vi "Lab Panel V4.0.vi"() -> ()   [LabVIEW 2013]
uses:
  <vilib>/Platform/TimedLoop/XDataNode/timing_clust.ctl
  <vilib>/Platform/TimedLoop/XDataNode/nitl_modes.ctl
  <vilib>/Platform/TimedLoop/XDataNode/wakeup.ctl
  Global 1.vi
  <vilib>/platform/TimedLoop/XDataNode/XDataNode.xnode
  <vilib>/Platform/TimedLoop/XDataNode/XDNodeRunTimeDep.lvlib
panel:
  out "TEMP update":bool
  out "AI update":bool
  in  "stop":bool
  in  "Tab Control 2":T1(tab)
  out "SIG LAB05-2":T2 {"PF" format="%.2f"; "AMPS" format="%.1f"}
  out "SIG LAB05-1":T2 {"PF" format="%.2f"; "AMPS" format="%.1f"}
  out "SIG LAB04-2":T2 {"PF" format="%.2f"; "AMPS" format="%.1f"}
  out "SIG LAB04-1":T2 {"PF" format="%.2f"; "AMPS" format="%.1f"}
  out "SIG LAB03-2":T2 {"PF" format="%.2f"; "AMPS" format="%.1f"}
  out "SIG LAB03-1":T2 {"PF" format="%.2f"; "AMPS" format="%.1f"}
  out "SIG LAB02-2":T2 {"PF" format="%.2f"; "AMPS" format="%.1f"}
  in  "RUN LAB01-1":bool
  in  "O/I  LAB05-1":bool
  in  "O/I  LAB05-2":bool
  in  "O/I  LAB04-1":bool
  in  "O/I  LAB04-2":bool
  in  "O/I  LAB02-1":bool
  in  "O/1  LAB02-2":bool
  in  "O/I  LAB01-2":bool
  in  "O/I  LAB01-1":bool
  in  "O/I  LAB03-1":bool
  in  "RUN LAB05-2":bool
  in  "RUN LAB05-1":bool
  in  "RUN LAB04-2":bool
  in  "RUN LAB04-1":bool
  in  "RUN LAB03-2":bool
  in  "RUN LAB03-1":bool
  in  "RUN LAB02-2":bool
  in  "RUN LAB02-1":bool
  in  "RUN LAB01-2":bool
  in  "SELECT LAB05-2":T3(radio)
  in  "SELECT LAB05-1":T3(radio)
  in  "SELECT LAB04-2":T3(radio)
  in  "SELECT LAB04-1":T3(radio)
  in  "SELECT LAB03-2":T3(radio)
  in  "SELECT LAB03-1":T3(radio)
  in  "SELECT LAB02-2":T3(radio)
  in  "SELECT LAB02-1":T3(radio)
  in  "SELECT LAB01-2":T3(radio)
  in  "SELECT LAB01-1":T3(radio)
  in  "O/I  LAB03-2":bool
  out "SIG LAB01-1":T2 {"PF" format="%.2f"; "AMPS" format="%.1f"}
  out "SIG LAB01-2":T2 {"PF" format="%.2f"; "AMPS" format="%.1f"}
  out "SIG LAB02-1":T2 {"PF" format="%.2f"; "AMPS" format="%.1f"}
  out "DISP LAB05-2":T4 {"MINS" format="%.2g"}
  out "DISP LAB05-1":T4 {"MINS" format="%.2g"}
  out "DISP LAB04-2":T4 {"MINS" format="%.2g"}
  out "DISP LAB04-1":T4 {"MINS" format="%.2g"}
  out "DISP LAB03-2":T4 {"MINS" format="%.2g"}
  out "DISP LAB03-1":T4 {"MINS" format="%.2g"}
  in  "SET LAB05-2":T5={"NAME"="", "DESCRIPTION"="", "CYCLES"=5.0, "T-RISE mins"=0.0, "T-RISE deg C"=0.0} {"CYCLES" min=5.0 step=1.0}
  in  "SET LAB05-1":T5={"NAME"="", "DESCRIPTION"="", "CYCLES"=5.0, "T-RISE mins"=0.0, "T-RISE deg C"=0.0} {"CYCLES" min=5.0 step=1.0}
  in  "SET LAB04-2":T5={"NAME"="", "DESCRIPTION"="", "CYCLES"=5.0, "T-RISE mins"=0.0, "T-RISE deg C"=0.0} {"CYCLES" min=5.0 step=1.0}
  in  "SET LAB04-1":T5={"NAME"="", "DESCRIPTION"="", "CYCLES"=5.0, "T-RISE mins"=0.0, "T-RISE deg C"=0.0} {"CYCLES" min=5.0 step=1.0}
  in  "SET LAB03-2":T5={"NAME"="", "DESCRIPTION"="", "CYCLES"=5.0, "T-RISE mins"=0.0, "T-RISE deg C"=0.0} {"CYCLES" min=5.0 step=1.0}
  in  "SET LAB03-1":T5={"NAME"="", "DESCRIPTION"="", "CYCLES"=5.0, "T-RISE mins"=0.0, "T-RISE deg C"=0.0} {"CYCLES" min=5.0 step=1.0}
  out "DISP LAB02-2":T4 {"MINS" format="%.2g"}
  out "DISP LAB02-1":T4 {"MINS" format="%.2g"}
  in  "SET LAB02-2":T5={"NAME"="", "DESCRIPTION"="", "CYCLES"=5.0, "T-RISE mins"=0.0, "T-RISE deg C"=0.0} {"CYCLES" min=5.0 step=1.0}
  in  "SET LAB02-1":T5={"NAME"="", "DESCRIPTION"="", "CYCLES"=5.0, "T-RISE mins"=0.0, "T-RISE deg C"=0.0} {"CYCLES" min=5.0 step=1.0}
  out "RESULT LAB05-2":bool
  out "RESULT LAB05-1":bool
  out "RESULT LAB04-2":bool
  out "RESULT LAB04-1":bool
  out "RESULT LAB03-2":bool
  out "RESULT LAB03-1":bool
  out "RESULT LAB02-2":bool
  out "RESULT LAB02-1":bool
  out "RESULT LAB01-2":bool
  out "RESULT LAB01-1":bool
  in  "SET LAB01-1":T5={"NAME"="", "DESCRIPTION"="", "CYCLES"=5.0, "T-RISE mins"=0.0, "T-RISE deg C"=0.0} {"CYCLES" min=5.0 step=1.0}
  in  "SET LAB01-2":T5={"NAME"="", "DESCRIPTION"="", "CYCLES"=5.0, "T-RISE mins"=0.0, "T-RISE deg C"=0.0} {"CYCLES" min=5.0 step=1.0}
  out "DISP LAB01-1":T4 {"MINS" format="%.2g"}
  out "DISP LAB01-2":T4 {"MINS" format="%.2f"}
  out "TEMP RISE LAB05-2":cluster{"TL":dbl, "TN":dbl}
  out "TEMP RISE LAB05-1":cluster{"TL":dbl, "TN":dbl}
  out "TEMP RISE LAB04-2":cluster{"TL":dbl, "TN":dbl}
  out "TEMP RISE LAB04-1":cluster{"TL":dbl, "TN":dbl}
  out "TEMP RISE LAB03-2":cluster{"TL":dbl, "TN":dbl}
  out "TEMP RISE LAB03-1":cluster{"TL":dbl, "TN":dbl}
  out "TEMP RISE LAB02-2":cluster{"TL":dbl, "TN":dbl}
  out "TEMP RISE LAB02-1":cluster{"TL":dbl, "TN":dbl}
  out "TEMP RISE LAB01-2":cluster{"TL":dbl, "TN":dbl}
  out "TEMP RISE LAB01-1":cluster{"TL":dbl, "TN":dbl}
  in  "JIG OFF TIME (S)":dbl=2.0 min=2.0 max=10.0 step=0.5 format="%.1g"
  in  "JIG ON TIME (S)":dbl=1.0 min=1.0 max=10.0 step=0.5 format="%.1g"
  out "JIG LAB05-2":bool
  out "JIG LAB05-1":bool
  out "JIG LAB04-2":bool
  out "JIG LAB04-1":bool
  out "JIG LAB03-2":bool
  out "JIG LAB03-1":bool
  out "JIG LAB02-2":bool
  out "JIG LAB02-1":bool
  out "JIG LAB01-2":bool
  out "JIG LAB01-1":bool
  out "TEMP START LAB01-1":cluster{"TL":dbl, "TN":dbl}
  out "TEMP START LAB02-1":cluster{"TL":dbl, "TN":dbl}
  out "TEMP START LAB03-1":cluster{"TL":dbl, "TN":dbl}
  out "TEMP START LAB04-1":cluster{"TL":dbl, "TN":dbl}
  out "TEMP START LAB01-2":cluster{"TL":dbl, "TN":dbl}
  out "TEMP START LAB02-2":cluster{"TL":dbl, "TN":dbl}
  out "TEMP START LAB03-2":cluster{"TL":dbl, "TN":dbl}
  out "TEMP START LAB04-2":cluster{"TL":dbl, "TN":dbl}
  out "TEMP START LAB05-2":cluster{"TL":dbl, "TN":dbl}
  out "TEMP START LAB05-1":cluster{"TL":dbl, "TN":dbl}
  in  "MAIL SETTINGS":T6
  out "MAIL REPORT":string
  in  "TO (string):":string
  in  "Send Mail Now":bool
  in  "Auto Mail Send":bool
  in  "Network Directory":path
  out "CAL LAB01":T7 {"2 (TN) cal" min=0.0 step=0.01 format="%.2f"; "2 (TL) cal" min=0.0 step=0.01 format="%.2f"; "2 (PF) cal" min=0.0 step=0.01 format="%.2f"; "2 (V) cal" min=0.0 step=0.01 format="%.2f"; "2 (A) cal" min=0.0 step=0.01 format="%.2f"; "1 (TN) cal" min=0.0 step=0.01 format="%.2f"; "1 (TL) cal" min=0.0 step=0.01 format="%.2f"; "1 (PF) cal" min=0.0 step=0.01 format="%.2f"; "1 (V) cal" min=0.0 step=0.01 format="%.2f"; "1  (A) cal" min=0.0 step=0.01 format="%.2f"}
  out "CAL LAB03":T7 {"2 (TN) cal" min=0.0 step=0.01 format="%.2f"; "2 (TL) cal" min=0.0 step=0.01 format="%.2f"; "2 (PF) cal" min=0.0 step=0.01 format="%.2f"; "2 (V) cal" min=0.0 step=0.01 format="%.2f"; "2 (A) cal" min=0.0 step=0.01 format="%.2f"; "1 (TN) cal" min=0.0 step=0.01 format="%.2f"; "1 (TL) cal" min=0.0 step=0.01 format="%.2f"; "1 (PF) cal" min=0.0 step=0.01 format="%.2f"; "1 (V) cal" min=0.0 step=0.01 format="%.2f"; "1  (A) cal" min=0.0 step=0.01 format="%.2f"}
  out "CAL LAB02":T8 {"2 (TN) cal" min=0.0 step=0.01 format="%.2f"; "2 (TL) cal" min=0.0 step=0.01 format="%.2f"; "2 (PF) cal" min=0.0 step=0.01 format="%.2f"; "2 (V) cal" min=0.0 step=0.01 format="%.2f"; "2 (A) cal" min=0.0 step=0.01 format="%.2f"; "1 (TN) cal" min=0.0 step=0.01 format="%.2f"; "1 (TL) cal" min=0.0 step=0.01 format="%.2f"; "1 (PF) cal" min=0.0 step=0.01 format="%.2f"; "1 (V) cal" min=0.0 step=0.01 format="%.2f"; "1 (A) cal" min=0.0 step=0.01 format="%.2f"}
  out "CAL LAB05":T7 {"2 (TN) cal" min=0.0 step=0.01 format="%.2f"; "2 (TL) cal" min=0.0 step=0.01 format="%.2f"; "2 (PF) cal" min=0.0 step=0.01 format="%.2f"; "2 (V) cal" min=0.0 step=0.01 format="%.2f"; "2 (A) cal" min=0.0 step=0.01 format="%.2f"; "1 (TN) cal" min=0.0 step=0.01 format="%.2f"; "1 (TL) cal" min=0.0 step=0.01 format="%.2f"; "1 (PF) cal" min=0.0 step=0.01 format="%.2f"; "1 (V) cal" min=0.0 step=0.01 format="%.2f"; "1  (A) cal" min=0.0 step=0.01 format="%.2f"}
  out "CAL LAB04":T7 {"2 (TN) cal" min=0.0 step=0.01 format="%.2f"; "2 (TL) cal" min=0.0 step=0.01 format="%.2f"; "2 (PF) cal" min=0.0 step=0.01 format="%.2f"; "2 (V) cal" min=0.0 step=0.01 format="%.2f"; "2 (A) cal" min=0.0 step=0.01 format="%.2f"; "1 (TN) cal" min=0.0 step=0.01 format="%.2f"; "1 (TL) cal" min=0.0 step=0.01 format="%.2f"; "1 (PF) cal" min=0.0 step=0.01 format="%.2f"; "1 (V) cal" min=0.0 step=0.01 format="%.2f"; "1  (A) cal" min=0.0 step=0.01 format="%.2f"}
  out "calibration file error out":errorcluster
  in  "CALIBRATE":bool
  in  "SHOW ADMIN PAGE":bool
  out "FAIL LAB05-2":cluster{"LO":dbl, "HI":dbl}
  out "FAIL LAB05-1":cluster{"LO":dbl, "HI":dbl}
  out "FAIL LAB04-2":cluster{"LO":dbl, "HI":dbl}
  out "FAIL LAB04-1":cluster{"LO":dbl, "HI":dbl}
  out "FAIL LAB03-2":cluster{"LO":dbl, "HI":dbl}
  out "FAIL LAB03-1":cluster{"LO":dbl, "HI":dbl}
  out "FAIL LAB02-2":cluster{"LO":dbl, "HI":dbl}
  out "FAIL LAB02-1":cluster{"LO":dbl, "HI":dbl}
  out "FAIL LAB01-2":cluster{"LO":dbl, "HI":dbl}
  out "FAIL LAB01-1":cluster{"LO":dbl, "HI":dbl}
  out "DATA LAB05-2":refnum<k1>
  out "DATA LAB05-1":refnum<k1>
  out "DATA LAB04-2":refnum<k1>
  out "DATA LAB04-1":refnum<k1>
  out "DATA LAB03-2":refnum<k1>
  out "DATA LAB03-1":refnum<k1>
  out "DATA LAB02-2":refnum<k1>
  out "DATA LAB02-1":refnum<k1>
  out "DATA LAB01-2":refnum<k1>
  in  "C drive data root dir":path
  out "run lab05-2":bool
  out "run lab05-1":bool
  out "run lab04-2":bool
  out "run lab04-1":bool
  out "run lab03-2":bool
  out "run lab03-1":bool
  out "run lab02-2":bool
  out "run lab02-1":bool
  out "run lab01-2":bool
  out "run lab01-1":bool
  out "stop2":bool
  in  "Tab Control":T9(tab)
  out "LAB01-2 (GRAPH)":dynamicdata(graph)
  out "LAB01-1 (GRAPH)":dynamicdata(graph)
  out "LAB02-2 (GRAPH)":dynamicdata(graph)
  out "LAB02-1 (GRAPH)":dynamicdata(graph)
  out "LAB03-2 (GRAPH)":dynamicdata(graph)
  out "LAB03-1 (GRAPH)":dynamicdata(graph)
  out "LAB04-2 (GRAPH)":dynamicdata(graph)
  out "LAB04-1 (GRAPH)":dynamicdata(graph)
  out "LAB05-2 (GRAPH)":dynamicdata(graph)
  out "LAB05-1 (GRAPH)":dynamicdata(graph)
  out "LAB05 TEMP":T10
  out "LAB04 TEMP":T10
  out "LAB02 TEMP":T10
  out "LAB01 TEMP":T10
  out "LAB03 TEMP":T10
  out "Analog Error Array":errorcluster[](array[cluster])
  out "AI loop time":dbl format="%.6g"
  out "loops":dbl
  in  "loop  delay(mS)":dbl
  out "on loops":dbl
  out "off loops":dbl
  out "jig cycle":dbl
  out "data file error":errorcluster
  out "mail control":string
  out "DATA LAB01-1":refnum<k1>
  # "LAB01"
  # "LAB02"
  # "LAB05"
  # "LAB03"
  # "LAB04"
  # "LAB01"
  # "LAB02"
  # "LAB03"
  # "LAB04"
  # "LAB05"
  # "JIG SET"
  # "(Enter recipients address seperated by comma)"
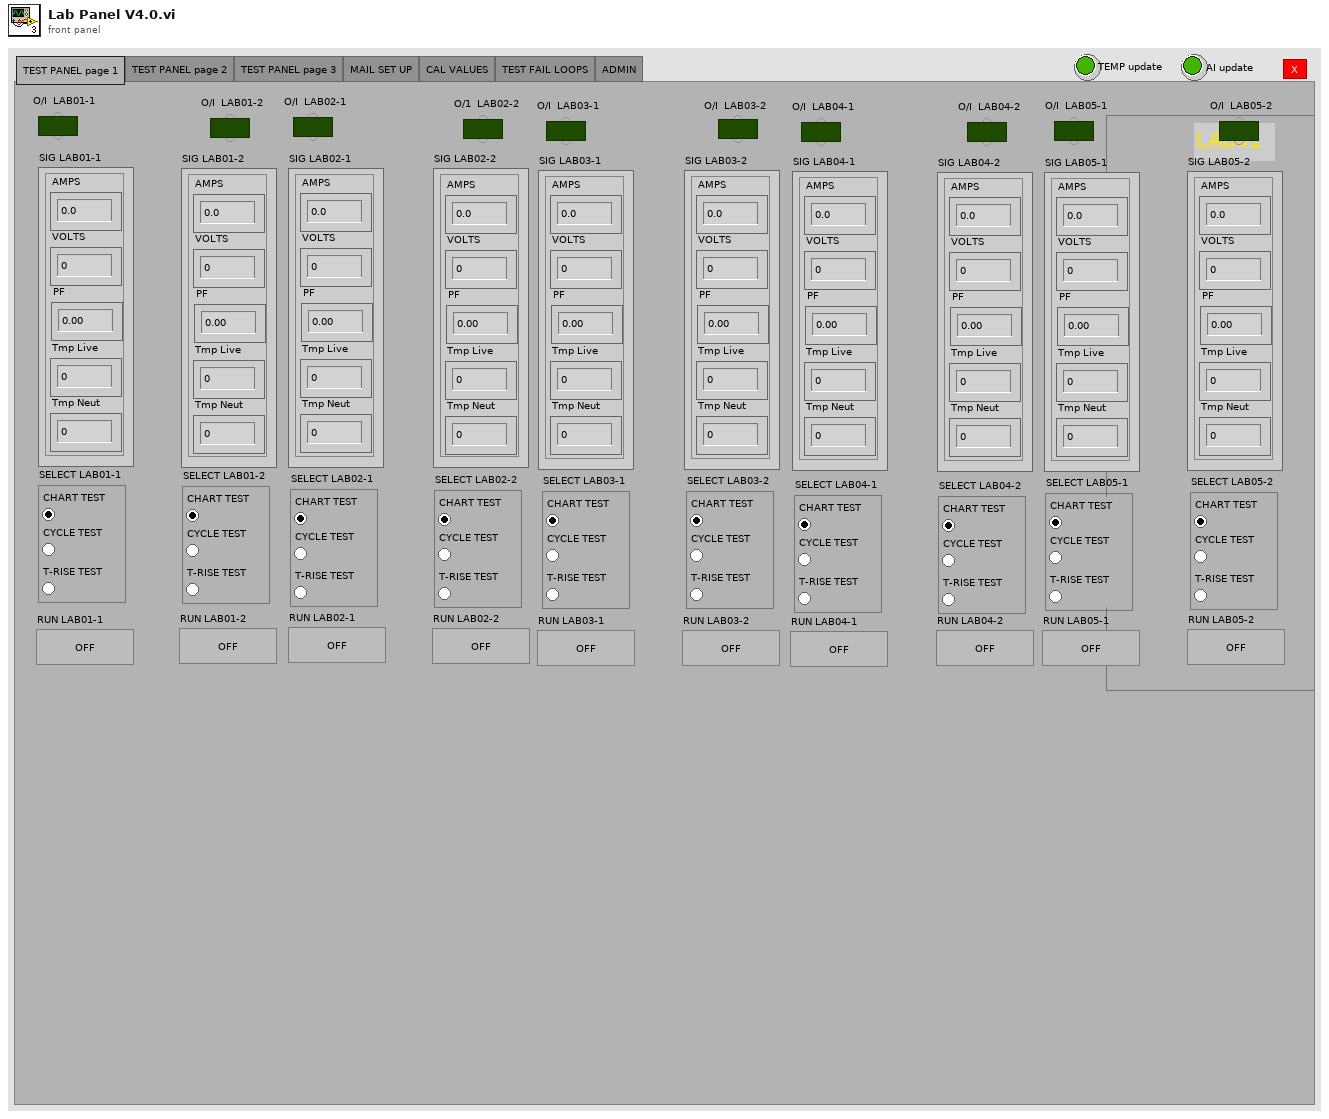
[diagram p1: front panel]
types:
  T1 = enum32{"TEST PANEL page 1", "TEST PANEL page 2", "TEST PANEL page 3", "MAIL SET UP", "CAL VALUES", "TEST FAIL LOOPS", "ADMIN"}
  T2 = cluster{"AMPS":dbl, "VOLTS":dbl, "PF":dbl, "Tmp Live":dbl, "Tmp Neut":dbl}
  T3 = enum32{"CHART TEST", "CYCLE TEST", "T-RISE TEST"}
  T4 = cluster{"CYCLE":dbl, "MINS":dbl, "STATUS":string}
  T5 = cluster{"NAME":string, "DESCRIPTION":string, "CYCLES":dbl, "T-RISE mins":dbl, "T-RISE deg C":dbl}
  T6 = cluster{"OUT SERVER ADDRESS":string, "FROM ACCOUNT":string, "USER NAME":string, "PASSWORD":string, "TEST MAIL":bool, "TEST MAIL STATUS":string, "mail error":errorcluster}
  T7 = cluster{"1  (A) cal":dbl, "1 (V) cal":dbl, "1 (PF) cal":dbl, "1 (TL) cal":dbl, "1 (TN) cal":dbl, "2 (A) cal":dbl, "2 (V) cal":dbl, "2 (PF) cal":dbl, "2 (TL) cal":dbl, "2 (TN) cal":dbl}
  T8 = cluster{"1 (A) cal":dbl, "1 (V) cal":dbl, "1 (PF) cal":dbl, "1 (TL) cal":dbl, "1 (TN) cal":dbl, "2 (A) cal":dbl, "2 (V) cal":dbl, "2 (PF) cal":dbl, "2 (TL) cal":dbl, "2 (TN) cal":dbl}
  T9 = enum32{"LAB01", "LAB02", "LAB03", "LAB04", "LAB05", "TEMPERATURE", "ERROR"}
  T10 = cluster{"T1 Live":dbl, "T1 Neut":dbl, "T2 Live":dbl, "T2 Neut":dbl, "ID":dbl, "ER":dbl}
  T11 = enum8{"Enabled", "Disabled", "Disabled and Grayed Out"}
  T12 = typedef "XDNodeRunTimeDep.lvlib/timing_clust.ctl" = cluster{"Expected End [f-1]":u64, "Actual End [f-1]":u64, "Finished Late? [f-1]":bool, "Expected End [i-1]":u64, "Actual End [i-1]":u64, "Finished Late? [i-1]":bool, "Expected Start [i]":u64, "Actual Start [i]":u64, "Expected Start [f]":u64, "Actual Start [f]":u64, "Source Name":string, "Structure Name":string, "Period":i64, "Deadline":i64, "Offset":i64, "Start":i64, "Priority":i32, "Timeout":i32, "Mode":T13, "Wakeup Reason":T14, "Error":errorcluster, "Source Type":string, "Secondary Source Type":string, "Global End Time":u64, "Global Start Time":u64, "Frame Duration":u64, "Iteration Duration":u64, "Assigned CPU":i32, "I/O Scan Engine Mode":u32}
  T13 = typedef "XDNodeRunTimeDep.lvlib/nitl_modes.ctl" = enum32{"No Change", "Process missed periods, maintain original phase", "Discard missed periods, maintain original phase", "Process missed periods, ignore original phase", "Discard missed periods, ignore original phase"}
  T14 = typedef "XDNodeRunTimeDep.lvlib/wakeup.ctl" = enum32{"Normal", "Aborted", "Asynchronous wakeup", "Timing source error", "Timed loop error", "Timeout"}
  T15 = enum16{"open", "replace", "create", "open or create", "replace or create", "replace or create with confirmation"}
  T16 = cluster{"SET LAB01-1":cluster{"NAME":string, "DESCRIPTION":string, "CYCLES":dbl, "T-RISE mins":dbl, "T-RISE deg C":dbl}, "SET LAB01-2":cluster{"NAME":string, "DESCRIPTION":string, "CYCLES":dbl, "T-RISE mins":dbl, "T-RISE deg C":dbl}, "SET LAB02-1":cluster{"NAME":string, "DESCRIPTION":string, "CYCLES":dbl, "T-RISE mins":dbl, "T-RISE deg C":dbl}, "SET LAB02-2":cluster{"NAME":string, "DESCRIPTION":string, "CYCLES":dbl, "T-RISE mins":dbl, "T-RISE deg C":dbl}, "SET LAB03-1":cluster{"NAME":string, "DESCRIPTION":string, "CYCLES":dbl, "T-RISE mins":dbl, "T-RISE deg C":dbl}, "SET LAB03-2":cluster{"NAME":string, "DESCRIPTION":string, "CYCLES":dbl, "T-RISE mins":dbl, "T-RISE deg C":dbl}, "SET LAB04-1":cluster{"NAME":string, "DESCRIPTION":string, "CYCLES":dbl, "T-RISE mins":dbl, "T-RISE deg C":dbl}, "SET LAB04-2":cluster{"NAME":string, "DESCRIPTION":string, "CYCLES":dbl, "T-RISE mins":dbl, "T-RISE deg C":dbl}, "SET LAB05-1":cluster{"NAME":string, "DESCRIPTION":string, "CYCLES":dbl, "T-RISE mins":dbl, "T-RISE deg C":dbl}, "SET LAB05-2":cluster{"NAME":string, "DESCRIPTION":string, "CYCLES":dbl, "T-RISE mins":dbl, "T-RISE deg C":dbl}, "Network Directory":path, "C drive data root dir":path}
  T17 = cluster{"MAIL SETTINGS":cluster{"OUT SERVER ADDRESS":string, "FROM ACCOUNT":string, "USER NAME":string, "PASSWORD":string, "TEST MAIL":bool, "TEST MAIL STATUS":string, "mail error":errorcluster}, "Auto Mail Send":bool, string}
  T18 = cluster{"SET LAB01-1":cluster{"NAME":string, "DESCRIPTION":string, "CYCLES":dbl, "T-RISE mins":dbl, "T-RISE deg C":dbl}, "SIG LAB01-1":cluster{"AMPS":dbl, "VOLTS":dbl, "PF":dbl, "Tmp Live":dbl, "Tmp Neut":dbl}, "DISP LAB01-1":cluster{"CYCLE":dbl, "MINS":dbl, "STATUS":string}}
  T19 = cluster{"SET LAB02-1":cluster{"NAME":string, "DESCRIPTION":string, "CYCLES":dbl, "T-RISE mins":dbl, "T-RISE deg C":dbl}, "SIG LAB02-1":cluster{"AMPS":dbl, "VOLTS":dbl, "PF":dbl, "Tmp Live":dbl, "Tmp Neut":dbl}, "DISP LAB02-1":cluster{"CYCLE":dbl, "MINS":dbl, "STATUS":string}}
  T20 = cluster{"SET LAB02-2":cluster{"NAME":string, "DESCRIPTION":string, "CYCLES":dbl, "T-RISE mins":dbl, "T-RISE deg C":dbl}, "SIG LAB02-2":cluster{"AMPS":dbl, "VOLTS":dbl, "PF":dbl, "Tmp Live":dbl, "Tmp Neut":dbl}, "DISP LAB02-2":cluster{"CYCLE":dbl, "MINS":dbl, "STATUS":string}}
  T21 = cluster{"SET LAB03-1":cluster{"NAME":string, "DESCRIPTION":string, "CYCLES":dbl, "T-RISE mins":dbl, "T-RISE deg C":dbl}, "SIG LAB03-1":cluster{"AMPS":dbl, "VOLTS":dbl, "PF":dbl, "Tmp Live":dbl, "Tmp Neut":dbl}, "DISP LAB03-1":cluster{"CYCLE":dbl, "MINS":dbl, "STATUS":string}}
  T22 = cluster{"SET LAB03-2":cluster{"NAME":string, "DESCRIPTION":string, "CYCLES":dbl, "T-RISE mins":dbl, "T-RISE deg C":dbl}, "SIG LAB03-2":cluster{"AMPS":dbl, "VOLTS":dbl, "PF":dbl, "Tmp Live":dbl, "Tmp Neut":dbl}, "DISP LAB03-2":cluster{"CYCLE":dbl, "MINS":dbl, "STATUS":string}}
  T23 = cluster{"SET LAB04-1":cluster{"NAME":string, "DESCRIPTION":string, "CYCLES":dbl, "T-RISE mins":dbl, "T-RISE deg C":dbl}, "SIG LAB04-1":cluster{"AMPS":dbl, "VOLTS":dbl, "PF":dbl, "Tmp Live":dbl, "Tmp Neut":dbl}, "DISP LAB04-1":cluster{"CYCLE":dbl, "MINS":dbl, "STATUS":string}}
  T24 = cluster{"SET LAB04-2":cluster{"NAME":string, "DESCRIPTION":string, "CYCLES":dbl, "T-RISE mins":dbl, "T-RISE deg C":dbl}, "SIG LAB04-2":cluster{"AMPS":dbl, "VOLTS":dbl, "PF":dbl, "Tmp Live":dbl, "Tmp Neut":dbl}, "DISP LAB04-2":cluster{"CYCLE":dbl, "MINS":dbl, "STATUS":string}}
  T25 = cluster{"SET LAB05-1":cluster{"NAME":string, "DESCRIPTION":string, "CYCLES":dbl, "T-RISE mins":dbl, "T-RISE deg C":dbl}, "SIG LAB05-1":cluster{"AMPS":dbl, "VOLTS":dbl, "PF":dbl, "Tmp Live":dbl, "Tmp Neut":dbl}, "DISP LAB05-1":cluster{"CYCLE":dbl, "MINS":dbl, "STATUS":string}}
  T26 = cluster{"SET LAB05-2":cluster{"NAME":string, "DESCRIPTION":string, "CYCLES":dbl, "T-RISE mins":dbl, "T-RISE deg C":dbl}, "SIG LAB05-2":cluster{"AMPS":dbl, "VOLTS":dbl, "PF":dbl, "Tmp Live":dbl, "Tmp Neut":dbl}, "DISP LAB05-2":cluster{"CYCLE":dbl, "MINS":dbl, "STATUS":string}}
  T27 = cluster{"T1":dbl, "T2":dbl, "T3":dbl, "T4":dbl, "ID":dbl, "ER":dbl}
  T28 = cluster{"LAB01-1 (A)":dbl, "LAB01-1 (V)":dbl, "LAB01-1 (PF)":dbl, "LAB01-2 (A)":dbl, "LAB01-2 (V)":dbl, "LAB01-2 (PF)":dbl}
  T29 = cluster{"LAB02-1 (A)":dbl, "LAB02-1 (V)":dbl, "LAB02-1 (PF)":dbl, "LAB02-2 (A)":dbl, "LAB02-2 (V)":dbl, "LAB02-2 (PF)":dbl}
  T30 = cluster{"LAB03-1 (A)":dbl, "LAB03-1 (V)":dbl, "LAB03-1 (PF)":dbl, "LAB03-2 (A)":dbl, "LAB03-2 (V)":dbl, "LAB03-2 (PF)":dbl}
  T31 = cluster{"LAB04-1 (A)":dbl, "LAB04-1 (V)":dbl, "LAB04-1 (PF)":dbl, "LAB04-2 (A)":dbl, "LAB04-2 (V)":dbl, "LAB04-2 (PF)":dbl}
  T32 = cluster{"LAB05-1 (A)":dbl, "LAB05-1 (V)":dbl, "LAB05-1 (PF)":dbl, "LAB05-2 (A)":dbl, "LAB05-2 (V)":dbl, "LAB05-2 (PF)":dbl}
  T33 = cluster{"SET LAB01-2":cluster{"NAME":string, "DESCRIPTION":string, "CYCLES":dbl, "T-RISE mins":dbl, "T-RISE deg C":dbl}, "SIG LAB01-2":cluster{"AMPS":dbl, "VOLTS":dbl, "PF":dbl, "Tmp Live":dbl, "Tmp Neut":dbl}, "DISP LAB01-2":cluster{"CYCLE":dbl, "MINS":dbl, "STATUS":string}}
  T34 = cluster{"FAIL LAB01-1":cluster{"LO":dbl, "HI":dbl}, "SIG LAB01-1":cluster{"AMPS":dbl, "VOLTS":dbl, "PF":dbl, "Tmp Live":dbl, "Tmp Neut":dbl}, "TEMP START LAB01-1":cluster{"TL":dbl, "TN":dbl}, "DISP LAB01-1":cluster{"CYCLE":dbl, "MINS":dbl, "STATUS":string}, "SET LAB01-1":cluster{"NAME":string, "DESCRIPTION":string, "CYCLES":dbl, "T-RISE mins":dbl, "T-RISE deg C":dbl}, "DATA LAB01-1":refnum<k1>}
  T35 = cluster{"FAIL LAB01-2":cluster{"LO":dbl, "HI":dbl}, "SIG LAB01-2":cluster{"AMPS":dbl, "VOLTS":dbl, "PF":dbl, "Tmp Live":dbl, "Tmp Neut":dbl}, "TEMP START LAB01-2":cluster{"TL":dbl, "TN":dbl}, "DISP LAB01-2":cluster{"CYCLE":dbl, "MINS":dbl, "STATUS":string}, "SET LAB01-2":cluster{"NAME":string, "DESCRIPTION":string, "CYCLES":dbl, "T-RISE mins":dbl, "T-RISE deg C":dbl}, "DATA LAB01-2":refnum<k1>}
  T36 = cluster{"FAIL LAB02-1":cluster{"LO":dbl, "HI":dbl}, "SIG LAB02-1":cluster{"AMPS":dbl, "VOLTS":dbl, "PF":dbl, "Tmp Live":dbl, "Tmp Neut":dbl}, "TEMP START LAB02-1":cluster{"TL":dbl, "TN":dbl}, "DISP LAB02-1":cluster{"CYCLE":dbl, "MINS":dbl, "STATUS":string}, "SET LAB02-1":cluster{"NAME":string, "DESCRIPTION":string, "CYCLES":dbl, "T-RISE mins":dbl, "T-RISE deg C":dbl}, "DATA LAB02-1":refnum<k1>}
  T37 = cluster{"FAIL LAB02-2":cluster{"LO":dbl, "HI":dbl}, "SIG LAB02-2":cluster{"AMPS":dbl, "VOLTS":dbl, "PF":dbl, "Tmp Live":dbl, "Tmp Neut":dbl}, "TEMP START LAB02-2":cluster{"TL":dbl, "TN":dbl}, "DISP LAB02-2":cluster{"CYCLE":dbl, "MINS":dbl, "STATUS":string}, "SET LAB02-2":cluster{"NAME":string, "DESCRIPTION":string, "CYCLES":dbl, "T-RISE mins":dbl, "T-RISE deg C":dbl}, "DATA LAB02-2":refnum<k1>}
  T38 = cluster{"FAIL LAB03-1":cluster{"LO":dbl, "HI":dbl}, "SIG LAB03-1":cluster{"AMPS":dbl, "VOLTS":dbl, "PF":dbl, "Tmp Live":dbl, "Tmp Neut":dbl}, "TEMP START LAB03-1":cluster{"TL":dbl, "TN":dbl}, "DISP LAB03-1":cluster{"CYCLE":dbl, "MINS":dbl, "STATUS":string}, "SET LAB03-1":cluster{"NAME":string, "DESCRIPTION":string, "CYCLES":dbl, "T-RISE mins":dbl, "T-RISE deg C":dbl}, "DATA LAB03-1":refnum<k1>}
  T39 = cluster{"FAIL LAB03-2":cluster{"LO":dbl, "HI":dbl}, "SIG LAB03-2":cluster{"AMPS":dbl, "VOLTS":dbl, "PF":dbl, "Tmp Live":dbl, "Tmp Neut":dbl}, "TEMP START LAB03-2":cluster{"TL":dbl, "TN":dbl}, "DISP LAB03-2":cluster{"CYCLE":dbl, "MINS":dbl, "STATUS":string}, "SET LAB03-2":cluster{"NAME":string, "DESCRIPTION":string, "CYCLES":dbl, "T-RISE mins":dbl, "T-RISE deg C":dbl}, "DATA LAB03-2":refnum<k1>}
  T40 = cluster{"FAIL LAB04-1":cluster{"LO":dbl, "HI":dbl}, "SIG LAB04-1":cluster{"AMPS":dbl, "VOLTS":dbl, "PF":dbl, "Tmp Live":dbl, "Tmp Neut":dbl}, "TEMP START LAB04-1":cluster{"TL":dbl, "TN":dbl}, "DISP LAB04-1":cluster{"CYCLE":dbl, "MINS":dbl, "STATUS":string}, "SET LAB04-1":cluster{"NAME":string, "DESCRIPTION":string, "CYCLES":dbl, "T-RISE mins":dbl, "T-RISE deg C":dbl}, "DATA LAB04-1":refnum<k1>}
  T41 = cluster{"FAIL LAB04-2":cluster{"LO":dbl, "HI":dbl}, "SIG LAB04-2":cluster{"AMPS":dbl, "VOLTS":dbl, "PF":dbl, "Tmp Live":dbl, "Tmp Neut":dbl}, "TEMP START LAB04-2":cluster{"TL":dbl, "TN":dbl}, "DISP LAB04-2":cluster{"CYCLE":dbl, "MINS":dbl, "STATUS":string}, "SET LAB04-2":cluster{"NAME":string, "DESCRIPTION":string, "CYCLES":dbl, "T-RISE mins":dbl, "T-RISE deg C":dbl}, "DATA LAB04-2":refnum<k1>}
  T42 = cluster{"FAIL LAB05-1":cluster{"LO":dbl, "HI":dbl}, "SIG LAB05-1":cluster{"AMPS":dbl, "VOLTS":dbl, "PF":dbl, "Tmp Live":dbl, "Tmp Neut":dbl}, "TEMP START LAB05-1":cluster{"TL":dbl, "TN":dbl}, "DISP LAB05-1":cluster{"CYCLE":dbl, "MINS":dbl, "STATUS":string}, "SET LAB05-1":cluster{"NAME":string, "DESCRIPTION":string, "CYCLES":dbl, "T-RISE mins":dbl, "T-RISE deg C":dbl}, "DATA LAB05-1":refnum<k1>}
  T43 = cluster{"FAIL LAB05-2":cluster{"LO":dbl, "HI":dbl}, "SIG LAB05-2":cluster{"AMPS":dbl, "VOLTS":dbl, "PF":dbl, "Tmp Live":dbl, "Tmp Neut":dbl}, "TEMP START LAB05-2":cluster{"TL":dbl, "TN":dbl}, "DISP LAB05-2":cluster{"CYCLE":dbl, "MINS":dbl, "STATUS":string}, "SET LAB05-2":cluster{"NAME":string, "DESCRIPTION":string, "CYCLES":dbl, "T-RISE mins":dbl, "T-RISE deg C":dbl}, "DATA LAB05-2":refnum<k1>}
  T44 = cluster{"MAIL SETTINGS":cluster{"OUT SERVER ADDRESS":string, "FROM ACCOUNT":string, "USER NAME":string, "PASSWORD":string, "TEST MAIL":bool, "TEST MAIL STATUS":string, "mail error":errorcluster}, "Auto Mail Send":bool, "TO (string):":string}
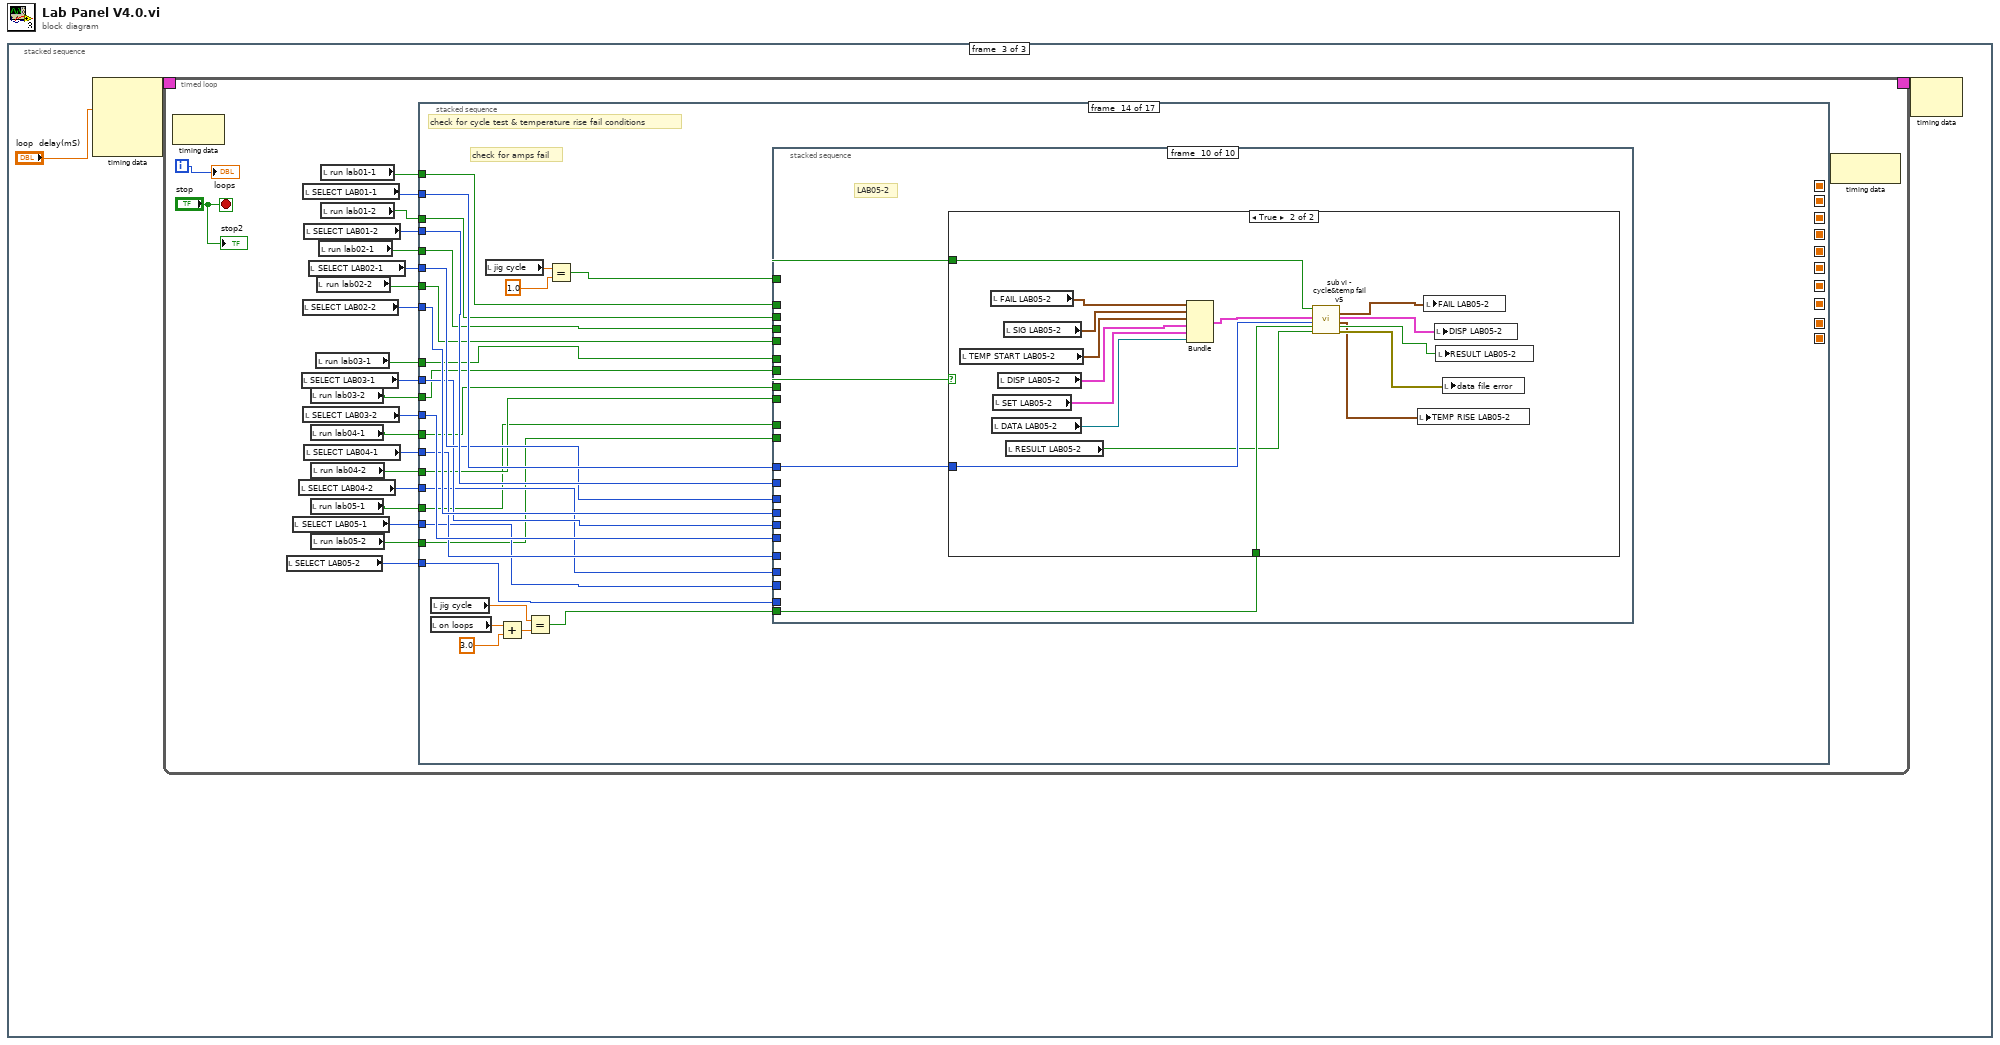
[diagram p0: block diagram]
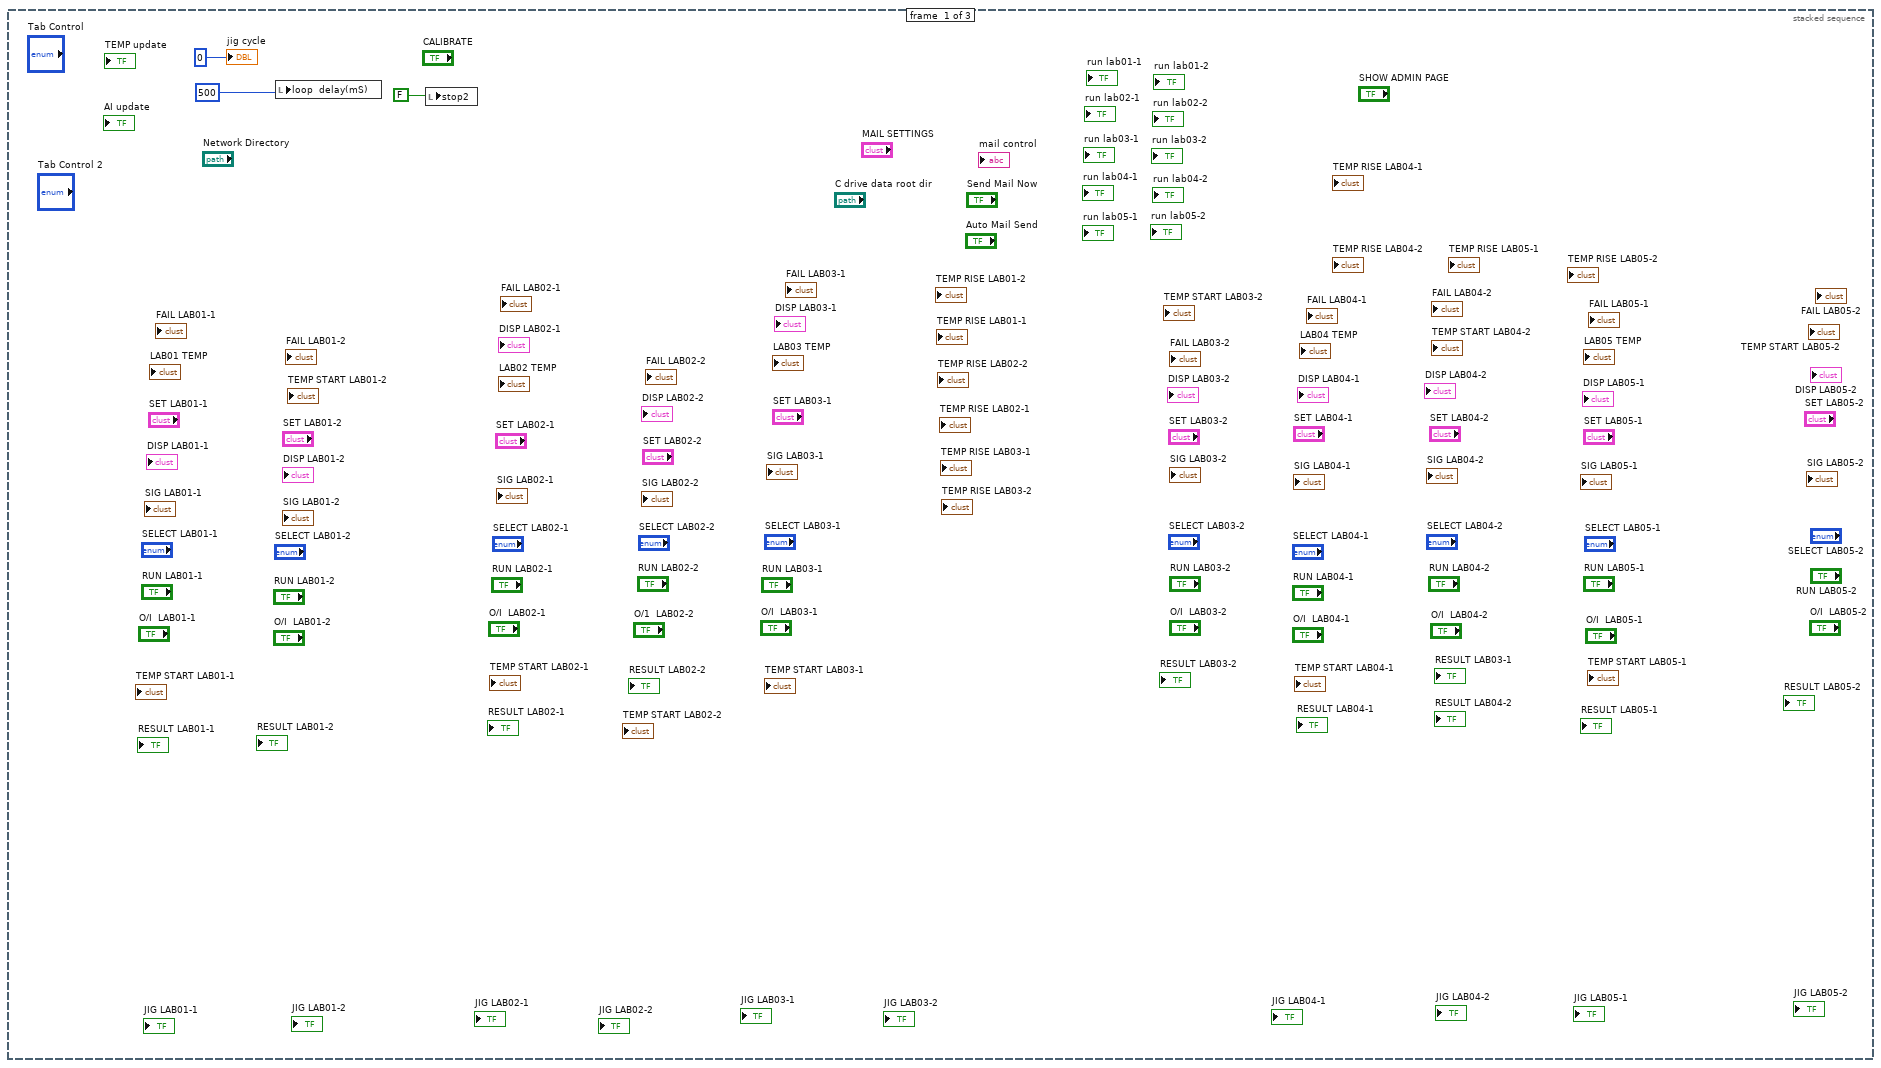
[diagram p2: hidden frame]
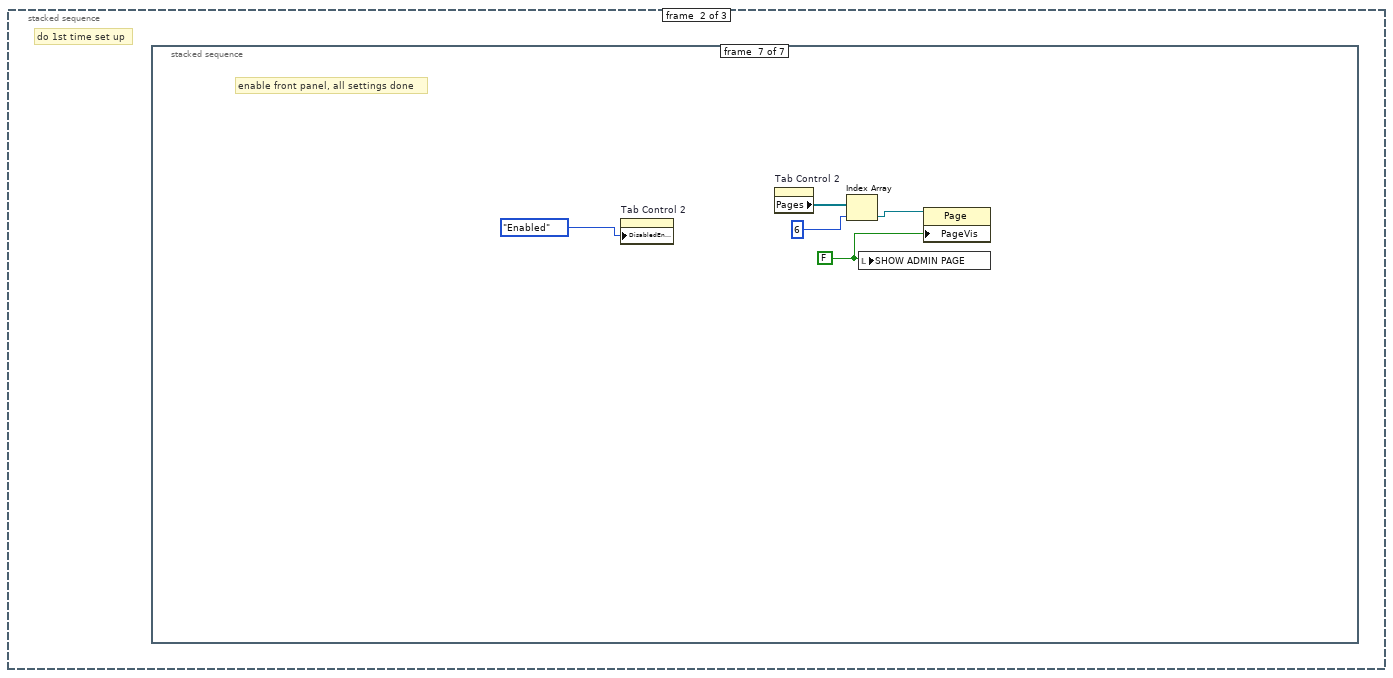
[diagram p3: hidden frame]
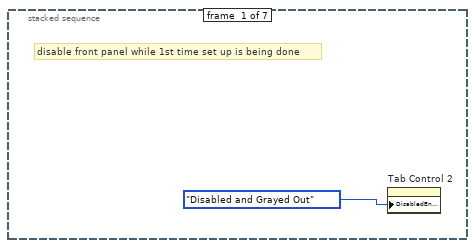
[diagram p4: hidden frame]
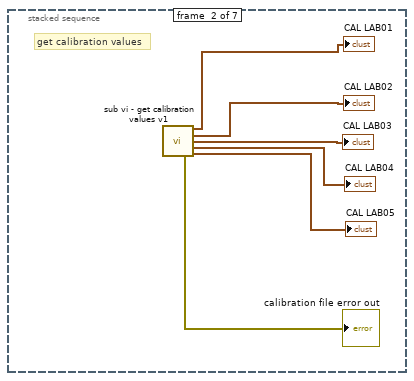
[diagram p5: hidden frame]
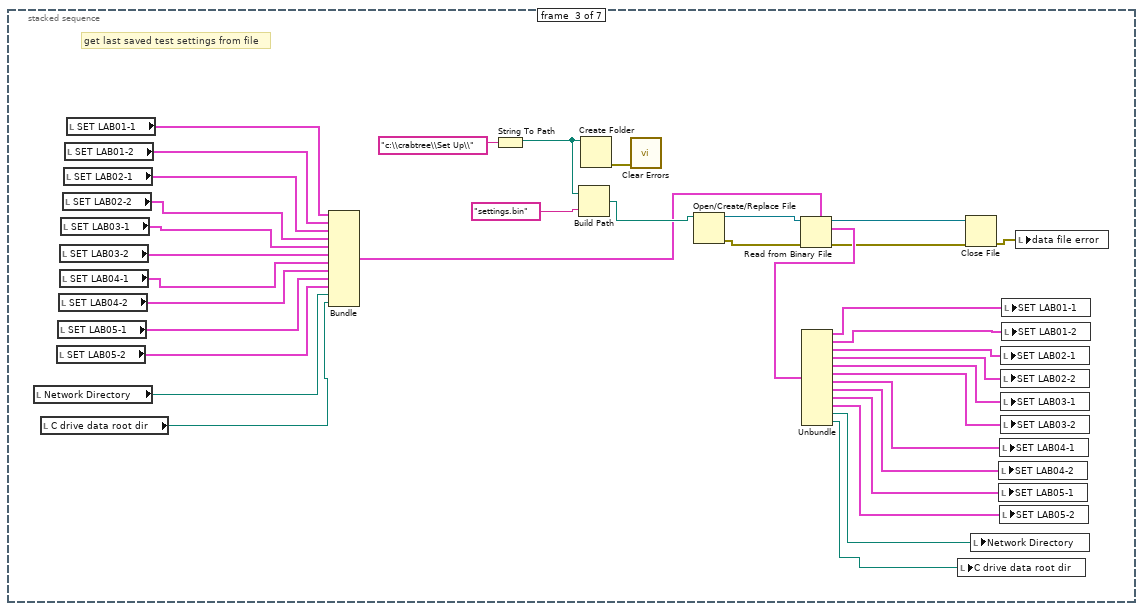
[diagram p6: hidden frame]
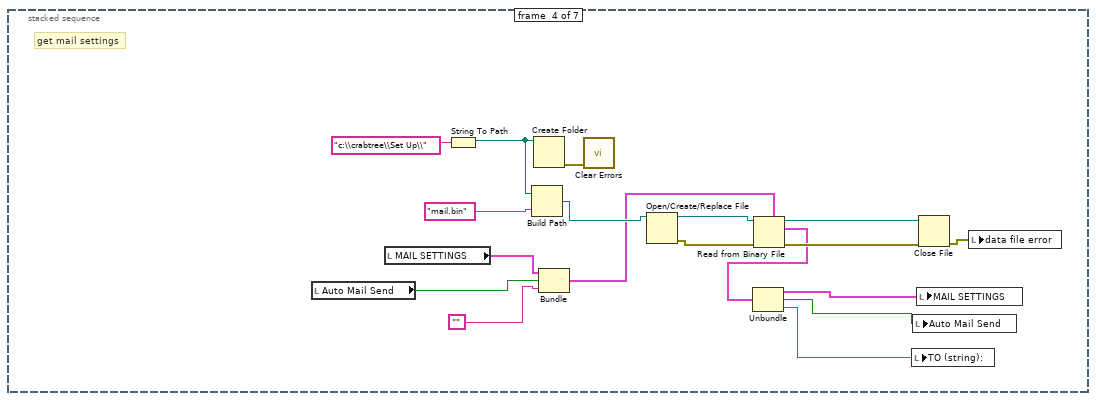
[diagram p7: hidden frame]
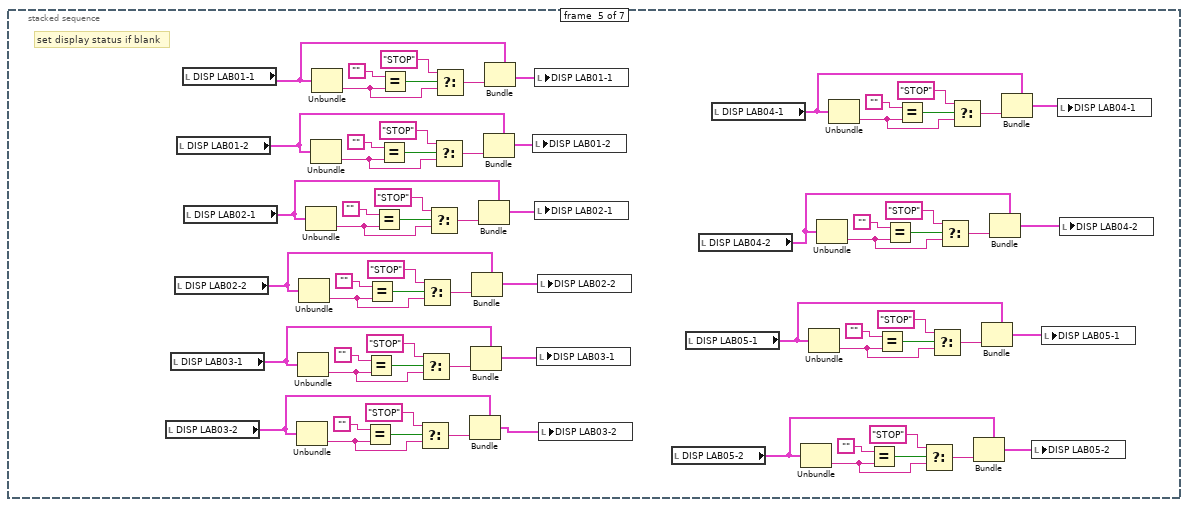
[diagram p8: hidden frame]
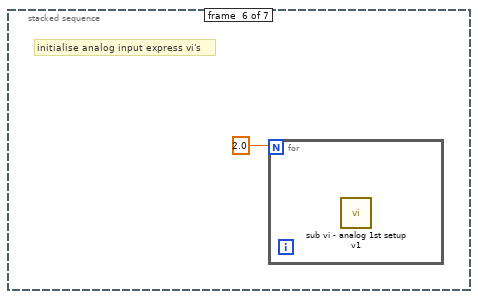
[diagram p9: hidden frame]
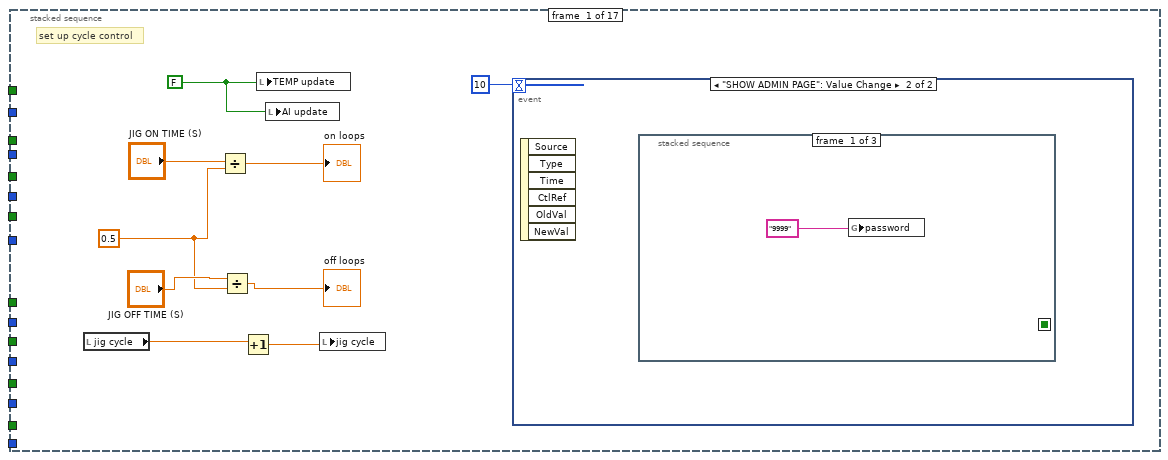
[diagram p10: hidden frame]
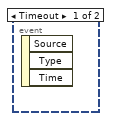
[diagram p11: hidden frame]
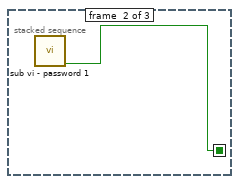
[diagram p12: hidden frame]
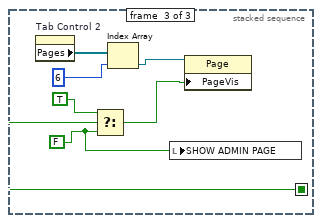
[diagram p13: hidden frame]
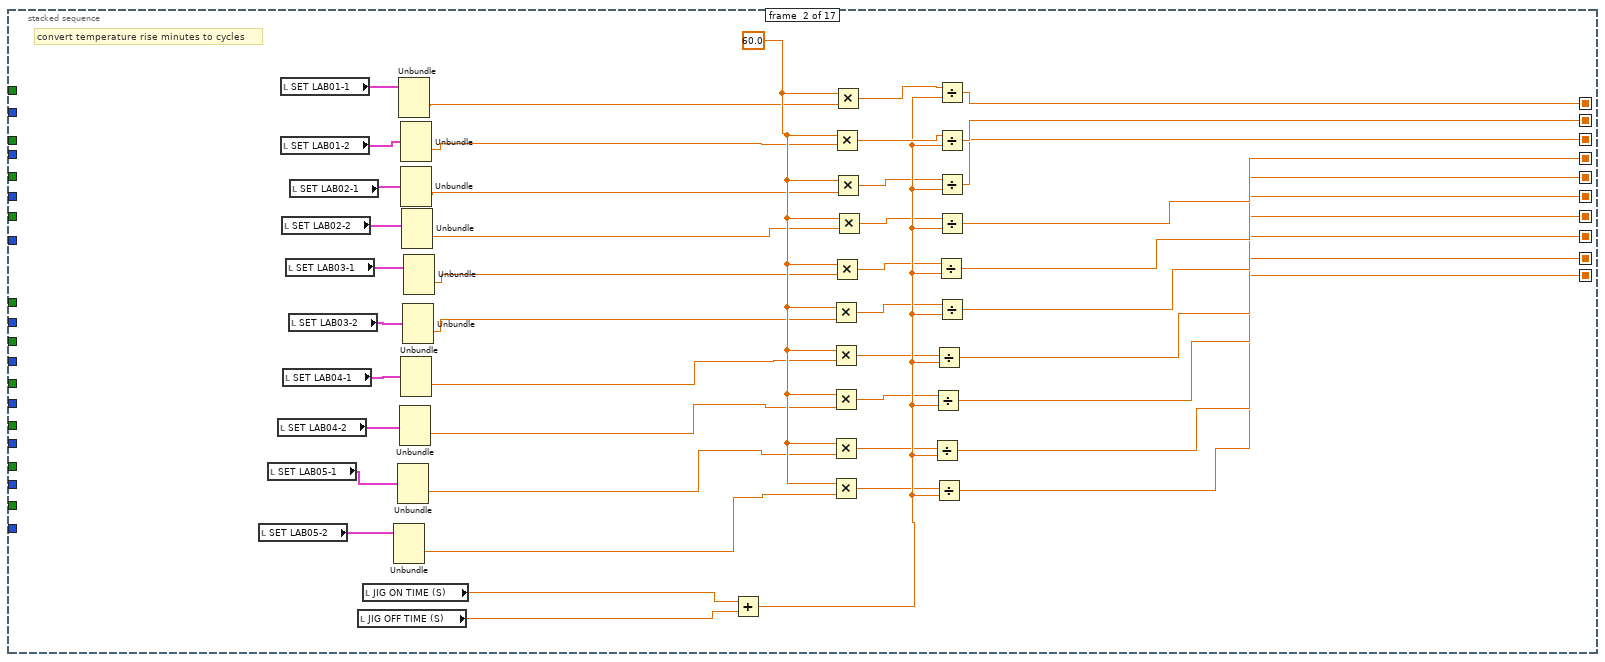
[diagram p14: hidden frame]
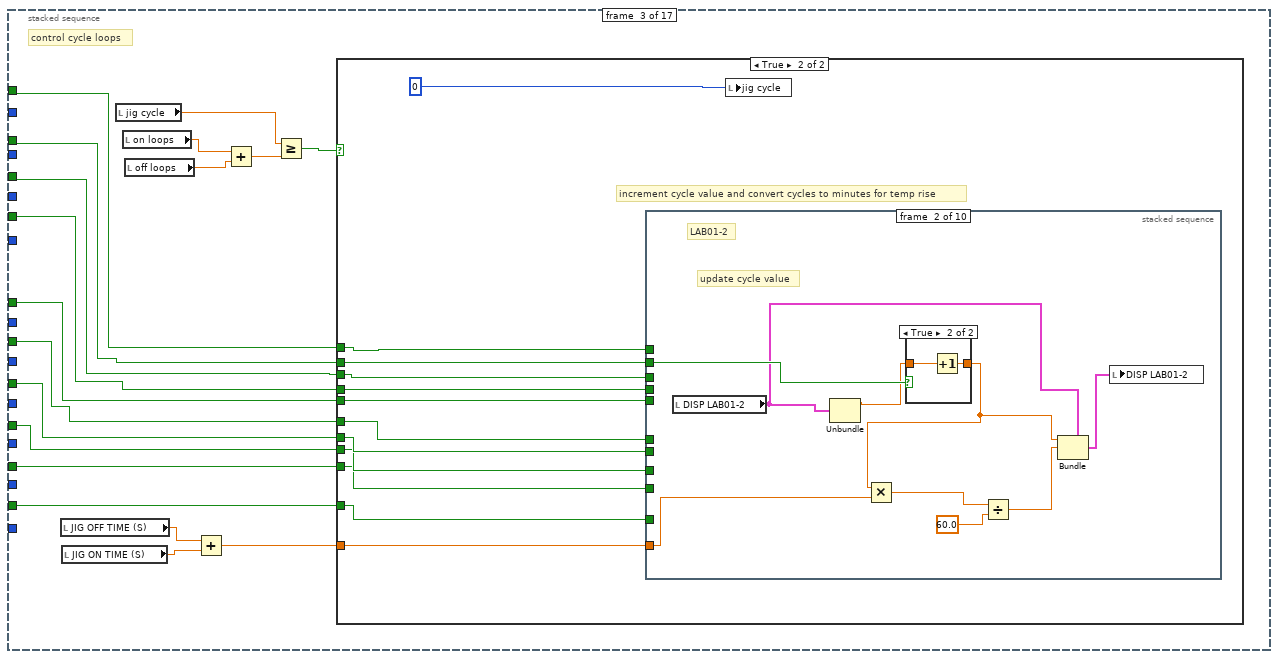
[diagram p15: hidden frame]
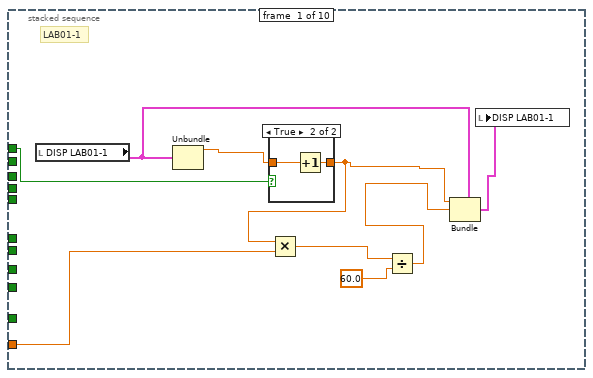
[diagram p17: hidden frame]
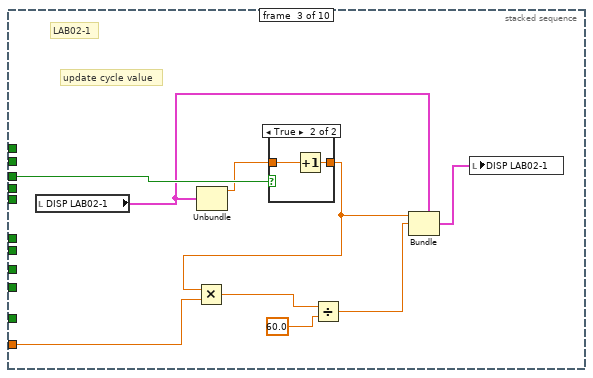
[diagram p20: hidden frame]
diagram:
  n1 = stacked-sequence {
    frame #0 {
      n2 = local write "loop  delay(mS)"(500) -> ()
      n3 = local write "stop2"(FALSE) -> ()
      "jig cycle" <- 0
    }
    frame #1 {
      # "do 1st time set up"
      n4 = stacked-sequence {
        frame #0 {
          # "disable front panel while 1st time set up is being done"
          n5 = property on="Tab Control 2" class="TabCtl (strict)"("DisabledEnum"=T11."Disabled and Grayed Out" ("Disabled")) -> ()  [unwired: 2 in, 2 out]
        }
        frame #1 {
          # "get calibration values"
          n6 = call "sub vi - get calibration values v1.vi"() -> ("LAB01 (CAL)"=→"CAL LAB01":T7, "LAB02 (CAL)"=→"CAL LAB02":T8, "LAB03 (CAL)"=→"CAL LAB03":T7, "LAB04 (CAL)"=→"CAL LAB04":T7, "calibration file error out"=→"calibration file error out":errorcluster, "LAB05 (CAL)"=→"CAL LAB05":T7)  [unwired: 10 in]
        }
        frame #2 {
          # "get last saved test settings from file"
          n7 = local read "Network Directory"() -> (w13:path)
          n8 = local read "C drive data root dir"() -> (w11:path)
          n9 = local read "SET LAB05-2"() -> (w43:T5)
          n10 = local read "SET LAB05-1"() -> (w44:T5)
          n11 = local read "SET LAB04-2"() -> (w45:T5)
          n12 = local read "SET LAB03-2"() -> (w42:T5)
          n13 = local read "SET LAB04-1"() -> (w46:T5)
          n14 = local read "SET LAB03-1"() -> (w41:T5)
          n15 = local read "SET LAB02-2"() -> (w40:T5)
          n16 = local read "SET LAB02-1"() -> (w39:T5)
          n17 = local read "SET LAB01-2"() -> (w38:T5)
          n18 = local read "SET LAB01-1"() -> (w37:T5)
          n19 = Bundle("SET LAB01-1"=w37, "SET LAB01-2"=w38, "SET LAB02-1"=w39, "SET LAB02-2"=w40, "SET LAB03-1"=w41, "SET LAB03-2"=w42, "SET LAB04-1"=w46, "SET LAB04-2"=w45, "SET LAB05-1"=w44, "SET LAB05-2"=w43, "Network Directory"=w13, "C drive data root dir"=w11) -> (w30:T16)  [unwired: 1 in]
          n20 = String To Path(string="c:\\crabtree\\Set Up\\") -> (path=w34:path)
          n21 = Build Path(base path=w34, name or relative path="settings.bin") -> (appended path=w32:path)
          n22 = Create Folder(path (use dialog)=w34) -> (error out=w36:errorcluster)  [unwired: 2 in, 2 out]
          n23 = call <vilib>:"Clear Errors.vi"("error in (no error)"=w36) -> ()  [unwired: 6 in, 1 out]
          n24 = Open/Create/Replace File(file path (use dialog)=w32) -> (refnum out=w29:refnum<file>, error out=w31:errorcluster)  [unwired: 5 in, 1 out]
          n25 = Read from Binary File(5:w30, 8:w31, 11:w29) -> (0:w26:errorcluster, 2:w28:T16, 3:w27:refnum<file>)  [unwired: 3 in, 1 out]
          n26 = Unbundle(w28) -> ("SET LAB01-1"=w24:T5, "SET LAB01-2"=w23:T5, "SET LAB02-1"=w22:T5, "SET LAB02-2"=w21:T5, "SET LAB03-1"=w20:T5, "SET LAB03-2"=w19:T5, "SET LAB04-1"=w18:T5, "SET LAB04-2"=w17:T5, "SET LAB05-1"=w16:T5, "SET LAB05-2"=w15:T5, "Network Directory"=w14:path, "C drive data root dir"=w12:path)
          n27 = local write "C drive data root dir"(w12) -> ()
          n28 = Close File(refnum=w27, error in=w26) -> (error out=w25:errorcluster)  [unwired: 1 out]
          n29 = local write "Network Directory"(w14) -> ()
          n30 = local write "SET LAB04-2"(w17) -> ()
          n31 = local write "SET LAB05-1"(w16) -> ()
          n32 = local write "SET LAB04-1"(w18) -> ()
          n33 = local write "SET LAB05-2"(w15) -> ()
          n34 = local write "SET LAB02-1"(w22) -> ()
          n35 = local write "SET LAB02-2"(w21) -> ()
          n36 = local write "SET LAB03-1"(w20) -> ()
          n37 = local write "SET LAB03-2"(w19) -> ()
          n38 = local write "SET LAB01-1"(w24) -> ()
          n39 = local write "SET LAB01-2"(w23) -> ()
          n40 = local write "data file error"(w25) -> ()
        }
        frame #3 {
          # "get mail settings"
          n41 = local read "Auto Mail Send"() -> (w50:bool)
          n42 = local read "MAIL SETTINGS"() -> (w54:T6)
          n43 = String To Path(string="c:\\crabtree\\Set Up\\") -> (path=w62:path)
          n44 = Build Path(base path=w62, name or relative path="mail.bin") -> (appended path=w60:path)
          n45 = Create Folder(path (use dialog)=w62) -> (error out=w64:errorcluster)  [unwired: 2 in, 2 out]
          n46 = Bundle("MAIL SETTINGS"=w54, "Auto Mail Send"=w50, "") -> (w53:T17)  [unwired: 1 in]
          n47 = call <vilib>:"Clear Errors.vi"("error in (no error)"=w64) -> ()  [unwired: 6 in, 1 out]
          n48 = Open/Create/Replace File(file path (use dialog)=w60) -> (refnum out=w58:refnum<file>, error out=w59:errorcluster)  [unwired: 5 in, 1 out]
          n49 = Read from Binary File(5:w53, 8:w59, 11:w58) -> (0:w56:errorcluster, 2:w52:T17, 3:w57:refnum<file>)  [unwired: 3 in, 1 out]
          n50 = Unbundle(w52) -> ("MAIL SETTINGS"=w51:T6, "Auto Mail Send"=w49:bool, w48:string)
          n51 = local write "TO (string):"(w48) -> ()
          n52 = local write "Auto Mail Send"(w49) -> ()
          n53 = local write "MAIL SETTINGS"(w51) -> ()
          n54 = Close File(refnum=w57, error in=w56) -> (error out=w55:errorcluster)  [unwired: 1 out]
          n55 = local write "data file error"(w55) -> ()
        }
        frame #4 {
          # "set display status if blank"
          n56 = local read "DISP LAB03-2"() -> (w94:T4)
          n57 = local read "DISP LAB03-1"() -> (w101:T4)
          n58 = local read "DISP LAB02-2"() -> (w108:T4)
          n59 = local read "DISP LAB01-2"() -> (w121:T4)
          n60 = local read "DISP LAB01-1"() -> (w130:T4)
          n61 = local read "DISP LAB02-1"() -> (w115:T4)
          n62 = Unbundle(w94) -> ("STATUS"=w96:string)  [unwired: 2 out]
          n63 = Unbundle(w101) -> ("STATUS"=w103:string)  [unwired: 2 out]
          n64 = Unbundle(w108) -> ("STATUS"=w110:string)  [unwired: 2 out]
          n65 = Unbundle(w115) -> ("STATUS"=w117:string)  [unwired: 2 out]
          n66 = Unbundle(w121) -> ("STATUS"=w124:string)  [unwired: 2 out]
          n67 = Unbundle(w130) -> ("STATUS"=w131:string)  [unwired: 2 out]
          n68 = Equal?(x="", y=w96) -> (x = y?=w98:bool)
          n69 = Equal?(x="", y=w103) -> (x = y?=w105:bool)
          n70 = Equal?(x="", y=w110) -> (x = y?=w112:bool)
          n71 = Equal?(x="", y=w117) -> (x = y?=w119:bool)
          n72 = Equal?(x="", y=w124) -> (x = y?=w126:bool)
          n73 = Equal?(x="", y=w131) -> (x = y?=w133:bool)
          n74 = Select(t="STOP", s=w98, f=w96) -> (s? t:f=w95:string)
          n75 = Select(t="STOP", s=w105, f=w103) -> (s? t:f=w102:string)
          n76 = Select(t="STOP", s=w112, f=w110) -> (s? t:f=w109:string)
          n77 = Select(t="STOP", s=w119, f=w117) -> (s? t:f=w116:string)
          n78 = Select(t="STOP", s=w126, f=w124) -> (s? t:f=w123:string)
          n79 = Select(t="STOP", s=w133, f=w131) -> (s? t:f=w129:string)
          n80 = Bundle(cluster=w94, "STATUS"=w95) -> (w93:T4)  [unwired: 2 in]
          n81 = Bundle(cluster=w101, "STATUS"=w102) -> (w100:T4)  [unwired: 2 in]
          n82 = Bundle(cluster=w108, "STATUS"=w109) -> (w107:T4)  [unwired: 2 in]
          n83 = Bundle(cluster=w115, "STATUS"=w116) -> (w114:T4)  [unwired: 2 in]
          n84 = Bundle(cluster=w121, "STATUS"=w123) -> (w122:T4)  [unwired: 2 in]
          n85 = Bundle(cluster=w130, "STATUS"=w129) -> (w128:T4)  [unwired: 2 in]
          n86 = local write "DISP LAB01-2"(w122) -> ()
          n87 = local write "DISP LAB01-1"(w128) -> ()
          n88 = local write "DISP LAB02-1"(w114) -> ()
          n89 = local write "DISP LAB03-1"(w100) -> ()
          n90 = local write "DISP LAB02-2"(w107) -> ()
          n91 = local write "DISP LAB03-2"(w93) -> ()
          n92 = local read "DISP LAB05-2"() -> (w66:T4)
          n93 = local read "DISP LAB05-1"() -> (w73:T4)
          n94 = local read "DISP LAB04-2"() -> (w75:T4)
          n95 = local read "DISP LAB04-1"() -> (w77:T4)
          n96 = Unbundle(w66) -> ("STATUS"=w68:string)  [unwired: 2 out]
          n97 = Unbundle(w73) -> ("STATUS"=w79:string)  [unwired: 2 out]
          n98 = Unbundle(w75) -> ("STATUS"=w84:string)  [unwired: 2 out]
          n99 = Unbundle(w77) -> ("STATUS"=w89:string)  [unwired: 2 out]
          n100 = Equal?(x="", y=w68) -> (x = y?=w70:bool)
          n101 = Equal?(x="", y=w79) -> (x = y?=w81:bool)
          n102 = Equal?(x="", y=w84) -> (x = y?=w86:bool)
          n103 = Equal?(x="", y=w89) -> (x = y?=w91:bool)
          n104 = Select(t="STOP", s=w70, f=w68) -> (s? t:f=w67:string)
          n105 = Select(t="STOP", s=w81, f=w79) -> (s? t:f=w78:string)
          n106 = Select(t="STOP", s=w86, f=w84) -> (s? t:f=w83:string)
          n107 = Select(t="STOP", s=w91, f=w89) -> (s? t:f=w88:string)
          n108 = Bundle(cluster=w66, "STATUS"=w67) -> (w65:T4)  [unwired: 2 in]
          n109 = Bundle(cluster=w73, "STATUS"=w78) -> (w72:T4)  [unwired: 2 in]
          n110 = Bundle(cluster=w75, "STATUS"=w83) -> (w74:T4)  [unwired: 2 in]
          n111 = Bundle(cluster=w77, "STATUS"=w88) -> (w76:T4)  [unwired: 2 in]
          n112 = local write "DISP LAB05-2"(w65) -> ()
          n113 = local write "DISP LAB05-1"(w72) -> ()
          n114 = local write "DISP LAB04-1"(w76) -> ()
          n115 = local write "DISP LAB04-2"(w74) -> ()
        }
        frame #5 {
          # "initialise analog input express vi's"
          n116 = for {
            N: 2.0 -> [_]
            n117 = call "sub vi - analog 1st setup v1.vi"() -> ()  [unwired: 11 in, 5 out]
          }
        }
        frame #6 {
          w136 = FALSE
          # "enable front panel, all settings done"
          n118 = property on="Tab Control 2" class="TabCtl (strict)"("DisabledEnum"=T11."Enabled" ("Disabled")) -> ()  [unwired: 2 in, 2 out]
          n119 = property on="Tab Control 2" class="TabCtl (strict)"() -> ("Pages"=w137:refnum<vi>[])  [unwired: 2 in, 2 out]
          n120 = Index Array(array=w137, index=6) -> (element=w139:refnum<vi>)
          n121 = local write "SHOW ADMIN PAGE"(w136) -> ()
          n122 = property class="Page"(reference=w139, "PageVis"=w136) -> ()  [unwired: 1 in, 2 out]
        }
      }
    }
    frame #2 {
      n123 = node-c288("loop  delay(mS)") -> (w143:T12)  [unwired: 3 in]
      n124 = timed-loop {
        timing: w143 -> [_]
        timing-out: [_] -> w142
        i -> [w165]
        stop <- "stop" stop-if-true
        n125 = node-c288() -> ()  [unwired: 1 in, 1 out]
        n126 = local read "SELECT LAB05-2"() -> (w145:T3)
        n127 = local read "SELECT LAB05-1"() -> (w146:T3)
        n128 = local read "SELECT LAB04-2"() -> (w147:T3)
        n129 = local read "SELECT LAB03-1"() -> (w150:T3)
        n130 = local read "SELECT LAB02-2"() -> (w151:T3)
        n131 = local read "SELECT LAB01-1"() -> (w154:T3)
        n132 = local read "SELECT LAB03-2"() -> (w149:T3)
        n133 = local read "SELECT LAB01-2"() -> (w153:T3)
        n134 = local read "SELECT LAB04-1"() -> (w148:T3)
        n135 = local read "SELECT LAB02-1"() -> (w152:T3)
        n136 = local read "run lab03-2"() -> (w159:bool)
        n137 = local read "run lab04-1"() -> (w158:bool)
        n138 = local read "run lab05-1"() -> (w156:bool)
        n139 = local read "run lab04-2"() -> (w157:bool)
        n140 = local read "run lab05-2"() -> (w155:bool)
        n141 = local read "run lab03-1"() -> (w160:bool)
        n142 = local read "run lab02-2"() -> (w161:bool)
        n143 = local read "run lab02-1"() -> (w162:bool)
        n144 = local read "run lab01-1"() -> (w164:bool)
        n145 = local read "run lab01-2"() -> (w163:bool)
        n146 = stacked-sequence {
          seq-local: [_ w227 _ _ _ _ _ _ _ _ _ _ _ _ _ _ _] -> [_ _ _ _ _ w1381 _ _ _ _ _ _ _ _ _ _ _]
          seq-local: [_ w226 _ _ _ _ _ _ _ _ _ _ _ _ _ _ _] -> [_ _ _ _ _ w1380 _ _ _ _ _ _ _ _ _ _ _]
          seq-local: [_ w213 _ _ _ _ _ _ _ _ _ _ _ _ _ _ _] -> [_ _ _ _ _ w1379 _ _ _ _ _ _ _ _ _ _ _]
          seq-local: [_ w212 _ _ _ _ _ _ _ _ _ _ _ _ _ _ _] -> [_ _ _ _ _ w1378 _ _ _ _ _ _ _ _ _ _ _]
          seq-local: [_ w211 _ _ _ _ _ _ _ _ _ _ _ _ _ _ _] -> [_ _ _ _ _ w1377 _ _ _ _ _ _ _ _ _ _ _]
          seq-local: [_ w210 _ _ _ _ _ _ _ _ _ _ _ _ _ _ _] -> [_ _ _ _ _ w1376 _ _ _ _ _ _ _ _ _ _ _]
          seq-local: [_ w209 _ _ _ _ _ _ _ _ _ _ _ _ _ _ _] -> [_ _ _ _ _ w1375 _ _ _ _ _ _ _ _ _ _ _]
          seq-local: [_ w208 _ _ _ _ _ _ _ _ _ _ _ _ _ _ _] -> [_ _ _ _ _ w1374 _ _ _ _ _ _ _ _ _ _ _]
          seq-local: [_ w207 _ _ _ _ _ _ _ _ _ _ _ _ _ _ _] -> [_ _ _ _ _ w1373 _ _ _ _ _ _ _ _ _ _ _]
          seq-local: [_ w206 _ _ _ _ _ _ _ _ _ _ _ _ _ _ _] -> [_ _ _ _ _ w1372 _ _ _ _ _ _ _ _ _ _ _]
          tunnel: w164 -> [_ _ w243 w408 w1031 w1401 w1661 w1876 _ _ _ _ w2321 w2429 _ _ w2704]
          tunnel: w163 -> [_ _ w242 w406 w1030 w1400 w1662 w1875 _ _ _ _ w2320 w2427 _ _ w2703]
          tunnel: w162 -> [_ _ w241 w404 w1029 w1399 w1660 w1874 _ _ _ _ w2319 w2425 _ _ w2702]
          tunnel: w161 -> [_ _ w240 w402 w1028 w1398 w1659 w1873 _ _ _ _ w2318 w2423 _ _ w2701]
          tunnel: w160 -> [_ _ w239 w400 w1027 w1397 w1658 w1872 _ _ _ _ w2317 w2421 _ _ w2700]
          tunnel: w159 -> [_ _ w238 w398 w1026 w1396 w1657 w1871 _ _ _ _ w2316 w2419 _ _ w2699]
          tunnel: w158 -> [_ _ w237 w396 w1025 w1395 w1656 w1870 _ _ _ _ w2315 w2417 _ _ w2698]
          tunnel: w157 -> [_ _ w236 w394 w1024 w1394 w1655 w1869 _ _ _ _ w2314 w2415 _ _ w2697]
          tunnel: w156 -> [_ _ w235 w392 w1023 w1393 w1654 w1868 _ _ _ _ w2313 w2413 _ _ w2696]
          tunnel: w155 -> [_ _ w234 w390 w1022 w1392 w1653 w1867 _ _ _ _ w2312 w2411 _ _ w2695]
          tunnel: w154 -> [_ _ _ w407 w1021 w1391 _ _ _ _ _ _ _ w2431 _ _ _]
          tunnel: w153 -> [_ _ _ w405 w1020 w1390 _ _ _ _ _ _ _ w2426 _ _ _]
          tunnel: w152 -> [_ _ _ w403 w1019 w1389 _ _ _ _ _ _ _ w2424 _ _ _]
          tunnel: w151 -> [_ _ _ w401 w1018 w1388 _ _ _ _ _ _ _ w2422 _ _ _]
          tunnel: w150 -> [_ _ _ w399 w1017 w1387 _ _ _ _ _ _ _ w2420 _ _ _]
          tunnel: w149 -> [_ _ _ w397 w1016 w1386 _ _ _ _ _ _ _ w2418 _ _ _]
          tunnel: w148 -> [_ _ _ w395 w1015 w1385 _ _ _ _ _ _ _ w2416 _ _ _]
          tunnel: w147 -> [_ _ _ w393 w1014 w1384 _ _ _ _ _ _ _ w2414 _ _ _]
          tunnel: w146 -> [_ _ _ w391 w1013 w1383 _ _ _ _ _ _ _ w2412 _ _ _]
          tunnel: w145 -> [_ _ _ w389 w1012 w1382 _ _ _ _ _ _ _ w2410 _ _ _]
          frame #0 {
            w169 = FALSE
            w174 = 0.5
            # "set up cycle control"
            n147 = local read "jig cycle"() -> (w173:dbl)
            n148 = Divide(x="JIG ON TIME (S)", y=w174) -> (x/y=→"on loops":dbl)
            n149 = Divide(x="JIG OFF TIME (S)", y=w174) -> (x/y=→"off loops":dbl)
            n150 = Increment(x=w173) -> (x+1=w172:dbl)
            n151 = local write "TEMP update"(w169) -> ()
            n152 = local write "AI update"(w169) -> ()
            n153 = local write "jig cycle"(w172) -> ()
            n154 = event shown="[1] \"SHOW ADMIN PAGE\": Value Change" {
              selector: _ -> [_ _]
              dyn-events: _ -> [_ _]
              timeout: 10 -> [_ _]
              event Timeout {
                n155 = event-data() -> ()  [unwired: 1 in, 3 out]
              }
              event "SHOW ADMIN PAGE": Value Change {
                n156 = event-data() -> ()  [unwired: 1 in, 6 out]
                n157 = stacked-sequence {
                  seq-local: [_ w178 _] -> [_ _ w179]
                  frame #0 {
                    n158 = global write "Global 1.vi" "password"("9999") -> ()
                  }
                  frame #1 {
                    n159 = call "sub vi - password 1.vi"() -> ("RESULT"=w178:bool)  [unwired: 11 in]
                  }
                  frame #2 {
                    w181 = FALSE
                    n160 = property on="Tab Control 2" class="TabCtl (strict)"() -> ("Pages"=w185:refnum<vi>[])  [unwired: 2 in, 2 out]
                    n161 = Select(t=TRUE, s=w179, f=w181) -> (s? t:f=w180:bool)
                    n162 = Index Array(array=w185, index=6) -> (element=w183:refnum<vi>)
                    n163 = local write "SHOW ADMIN PAGE"(w181) -> ()
                    n164 = property class="Page"(reference=w183, "PageVis"=w180) -> ()  [unwired: 1 in, 2 out]
                  }
                }
              }
            }
          }
          frame #1 {
            w223 = 60.0
            # "convert temperature rise minutes to cycles"
            n165 = local read "SET LAB05-2"() -> (w187:T5)
            n166 = local read "SET LAB05-1"() -> (w189:T5)
            n167 = local read "SET LAB04-2"() -> (w191:T5)
            n168 = local read "SET LAB01-1"() -> (w205:T5)
            n169 = local read "SET LAB01-2"() -> (w203:T5)
            n170 = local read "SET LAB02-2"() -> (w199:T5)
            n171 = local read "SET LAB04-1"() -> (w193:T5)
            n172 = local read "SET LAB03-1"() -> (w197:T5)
            n173 = local read "SET LAB03-2"() -> (w195:T5)
            n174 = local read "SET LAB02-1"() -> (w201:T5)
            n175 = local read "JIG OFF TIME (S)"() -> (w228:dbl)
            n176 = local read "JIG ON TIME (S)"() -> (w229:dbl)
            n177 = Unbundle(w187) -> ("T-RISE mins"=w186:dbl)  [unwired: 4 out]
            n178 = Unbundle(w189) -> ("T-RISE mins"=w188:dbl)  [unwired: 4 out]
            n179 = Unbundle(w205) -> ("T-RISE mins"=w204:dbl)  [unwired: 4 out]
            n180 = Unbundle(w191) -> ("T-RISE mins"=w190:dbl)  [unwired: 4 out]
            n181 = Unbundle(w203) -> ("T-RISE mins"=w202:dbl)  [unwired: 4 out]
            n182 = Unbundle(w201) -> ("T-RISE mins"=w200:dbl)  [unwired: 4 out]
            n183 = Unbundle(w193) -> ("T-RISE mins"=w192:dbl)  [unwired: 4 out]
            n184 = Unbundle(w199) -> ("T-RISE mins"=w198:dbl)  [unwired: 4 out]
            n185 = Unbundle(w195) -> ("T-RISE mins"=w194:dbl)  [unwired: 4 out]
            n186 = Unbundle(w197) -> ("T-RISE mins"=w196:dbl)  [unwired: 4 out]
            n187 = Add(x=w229, y=w228) -> (x+y=w222:dbl)
            n188 = Multiply(x=w223, y=w194) -> (x*y=w218:dbl)
            n189 = Multiply(x=w223, y=w192) -> (x*y=w217:dbl)
            n190 = Multiply(x=w223, y=w190) -> (x*y=w216:dbl)
            n191 = Multiply(x=w223, y=w188) -> (x*y=w215:dbl)
            n192 = Multiply(x=w223, y=w186) -> (x*y=w214:dbl)
            n193 = Multiply(x=w223, y=w202) -> (x*y=w224:dbl)
            n194 = Multiply(x=w223, y=w196) -> (x*y=w219:dbl)
            n195 = Multiply(x=w223, y=w204) -> (x*y=w225:dbl)
            n196 = Multiply(x=w223, y=w200) -> (x*y=w221:dbl)
            n197 = Multiply(x=w223, y=w198) -> (x*y=w220:dbl)
            n198 = Divide(x=w215, y=w222) -> (x/y=w207:dbl)
            n199 = Divide(x=w216, y=w222) -> (x/y=w208:dbl)
            n200 = Divide(x=w217, y=w222) -> (x/y=w209:dbl)
            n201 = Divide(x=w214, y=w222) -> (x/y=w206:dbl)
            n202 = Divide(x=w219, y=w222) -> (x/y=w211:dbl)
            n203 = Divide(x=w225, y=w222) -> (x/y=w227:dbl)
            n204 = Divide(x=w224, y=w222) -> (x/y=w226:dbl)
            n205 = Divide(x=w221, y=w222) -> (x/y=w213:dbl)
            n206 = Divide(x=w220, y=w222) -> (x/y=w212:dbl)
            n207 = Divide(x=w218, y=w222) -> (x/y=w210:dbl)
          }
          frame #2 {
            # "control cycle loops"
            n208 = local read "JIG OFF TIME (S)"() -> (w232:dbl)
            n209 = local read "JIG ON TIME (S)"() -> (w231:dbl)
            n210 = local read "jig cycle"() -> (w245:dbl)
            n211 = local read "on loops"() -> (w247:dbl)
            n212 = local read "off loops"() -> (w246:dbl)
            n213 = Add(x=w232, y=w231) -> (x+y=w230:dbl)
            n214 = Add(x=w247, y=w246) -> (x+y=w233:dbl)
            n215 = Greater Or Equal?(x=w245, y=w233) -> (x >= y?=w244:bool)
            n216 = case shown="True" w244 {
              tunnel: w243 -> [_ w258]
              tunnel: w242 -> [_ w257]
              tunnel: w241 -> [_ w256]
              tunnel: w240 -> [_ w255]
              tunnel: w239 -> [_ w254]
              tunnel: w238 -> [_ w253]
              tunnel: w237 -> [_ w252]
              tunnel: w236 -> [_ w251]
              tunnel: w235 -> [_ w250]
              tunnel: w234 -> [_ w249]
              tunnel: w230 -> [_ w248]
              frame False {
              }
              frame True {
                # "increment cycle value and convert cycles to minutes for temp rise"
                n217 = stacked-sequence {
                  tunnel: w258 -> [w268 _ _ _ _ _ _ _ _ _]
                  tunnel: w257 -> [_ w280 _ _ _ _ _ _ _ _]
                  tunnel: w256 -> [_ _ w292 _ _ _ _ _ _ _]
                  tunnel: w255 -> [_ _ _ w304 _ _ _ _ _ _]
                  tunnel: w254 -> [_ _ _ _ w316 _ _ _ _ _]
                  tunnel: w253 -> [_ _ _ _ _ w328 _ _ _ _]
                  tunnel: w252 -> [_ _ _ _ _ _ w340 _ _ _]
                  tunnel: w251 -> [_ _ _ _ _ _ _ w352 _ _]
                  tunnel: w250 -> [_ _ _ _ _ _ _ _ w364 _]
                  tunnel: w249 -> [_ _ _ _ _ _ _ _ _ w376]
                  tunnel: w248 -> [w265 w277 w289 w301 w313 w325 w337 w349 w361 w373]
                  frame #0 {
                    # "LAB01-1"
                    n218 = local read "DISP LAB01-1"() -> (w263:T4)
                    n219 = Unbundle(w263) -> ("CYCLE"=w264:dbl)  [unwired: 2 out]
                    n220 = case shown="True" w268 {
                      tunnel: w264 -> [w269 w271]
                      tunnel: [w269 w270] -> w262
                      frame False {
                      }
                      frame True {
                        n221 = Increment(x=w271) -> (x+1=w270:dbl)
                      }
                    }
                    n222 = Multiply(x=w262, y=w265) -> (x*y=w266:dbl)
                    n223 = Divide(x=w266, y=60.0) -> (x/y=w261:dbl)
                    n224 = Bundle(cluster=w263, "CYCLE"=w262, "MINS"=w261) -> (w260:T4)  [unwired: 1 in]
                    n225 = local write "DISP LAB01-1"(w260) -> ()
                  }
                  frame #1 {
                    # "update cycle value"
                    # "LAB01-2"
                    n226 = local read "DISP LAB01-2"() -> (w275:T4)
                    n227 = Unbundle(w275) -> ("CYCLE"=w276:dbl)  [unwired: 2 out]
                    n228 = case shown="True" w280 {
                      tunnel: w276 -> [w281 w283]
                      tunnel: [w281 w282] -> w273
                      frame False {
                      }
                      frame True {
                        n229 = Increment(x=w283) -> (x+1=w282:dbl)
                      }
                    }
                    n230 = Multiply(x=w273, y=w277) -> (x*y=w278:dbl)
                    n231 = Divide(x=w278, y=60.0) -> (x/y=w272:dbl)
                    n232 = Bundle(cluster=w275, "CYCLE"=w273, "MINS"=w272) -> (w274:T4)  [unwired: 1 in]
                    n233 = local write "DISP LAB01-2"(w274) -> ()
                  }
                  frame #2 {
                    # "update cycle value"
                    # "LAB02-1"
                    n234 = local read "DISP LAB02-1"() -> (w287:T4)
                    n235 = Unbundle(w287) -> ("CYCLE"=w288:dbl)  [unwired: 2 out]
                    n236 = case shown="True" w292 {
                      tunnel: [w293 w295] -> w285
                      tunnel: w288 -> [w293 w294]
                      frame False {
                      }
                      frame True {
                        n237 = Increment(x=w294) -> (x+1=w295:dbl)
                      }
                    }
                    n238 = Multiply(x=w285, y=w289) -> (x*y=w290:dbl)
                    n239 = Divide(x=w290, y=60.0) -> (x/y=w284:dbl)
                    n240 = Bundle(cluster=w287, "CYCLE"=w285, "MINS"=w284) -> (w286:T4)  [unwired: 1 in]
                    n241 = local write "DISP LAB02-1"(w286) -> ()
                  }
                  frame #3 {
                    # "update cycle value"
                    # "LAB02-2"
                    n242 = local read "DISP LAB02-2"() -> (w299:T4)
                    n243 = Unbundle(w299) -> ("CYCLE"=w300:dbl)  [unwired: 2 out]
                    n244 = case shown="True" w304 {
                      tunnel: [w305 w307] -> w298
                      tunnel: w300 -> [w305 w306]
                      frame False {
                      }
                      frame True {
                        n245 = Increment(x=w306) -> (x+1=w307:dbl)
                      }
                    }
                    n246 = Multiply(x=w298, y=w301) -> (x*y=w302:dbl)
                    n247 = Divide(x=w302, y=60.0) -> (x/y=w297:dbl)
                    n248 = Bundle(cluster=w299, "CYCLE"=w298, "MINS"=w297) -> (w296:T4)  [unwired: 1 in]
                    n249 = local write "DISP LAB02-2"(w296) -> ()
                  }
                  frame #4 {
                    # "update cycle value"
                    # "LAB03-1"
                    n250 = local read "DISP LAB03-1"() -> (w311:T4)
                    n251 = Unbundle(w311) -> ("CYCLE"=w312:dbl)  [unwired: 2 out]
                    n252 = case shown="True" w316 {
                      tunnel: [w317 w319] -> w308
                      tunnel: w312 -> [w317 w318]
                      frame False {
                      }
                      frame True {
                        n253 = Increment(x=w318) -> (x+1=w319:dbl)
                      }
                    }
                    n254 = Multiply(x=w308, y=w313) -> (x*y=w314:dbl)
                    n255 = Divide(x=w314, y=60.0) -> (x/y=w309:dbl)
                    n256 = Bundle(cluster=w311, "CYCLE"=w308, "MINS"=w309) -> (w310:T4)  [unwired: 1 in]
                    n257 = local write "DISP LAB03-1"(w310) -> ()
                  }
                  frame #5 {
                    # "update cycle value"
                    # "LAB03-2"
                    n258 = local read "DISP LAB03-2"() -> (w323:T4)
                    n259 = Unbundle(w323) -> ("CYCLE"=w324:dbl)  [unwired: 2 out]
                    n260 = case shown="False" w328 {
                      tunnel: [w329 w331] -> w322
                      tunnel: w324 -> [w329 w330]
                      frame False {
                      }
                      frame True {
                        n261 = Increment(x=w330) -> (x+1=w331:dbl)
                      }
                    }
                    n262 = Multiply(x=w322, y=w325) -> (x*y=w326:dbl)
                    n263 = Divide(x=w326, y=60.0) -> (x/y=w321:dbl)
                    n264 = Bundle(cluster=w323, "CYCLE"=w322, "MINS"=w321) -> (w320:T4)  [unwired: 1 in]
                    n265 = local write "DISP LAB03-2"(w320) -> ()
                  }
                  frame #6 {
                    # "update cycle value"
                    # "LAB04-1"
                    n266 = local read "DISP LAB04-1"() -> (w335:T4)
                    n267 = Unbundle(w335) -> ("CYCLE"=w336:dbl)  [unwired: 2 out]
                    n268 = case shown="True" w340 {
                      tunnel: [w341 w343] -> w333
                      tunnel: w336 -> [w341 w342]
                      frame False {
                      }
                      frame True {
                        n269 = Increment(x=w342) -> (x+1=w343:dbl)
                      }
                    }
                    n270 = Multiply(x=w333, y=w337) -> (x*y=w338:dbl)
                    n271 = Divide(x=w338, y=60.0) -> (x/y=w332:dbl)
                    n272 = Bundle(cluster=w335, "CYCLE"=w333, "MINS"=w332) -> (w334:T4)  [unwired: 1 in]
                    n273 = local write "DISP LAB04-1"(w334) -> ()
                  }
                  frame #7 {
                    # "update cycle value"
                    # "LAB04-2"
                    n274 = local read "DISP LAB04-2"() -> (w347:T4)
                    n275 = Unbundle(w347) -> ("CYCLE"=w348:dbl)  [unwired: 2 out]
                    n276 = case shown="True" w352 {
                      tunnel: [w353 w355] -> w345
                      tunnel: w348 -> [w353 w354]
                      frame False {
                      }
                      frame True {
                        n277 = Increment(x=w354) -> (x+1=w355:dbl)
                      }
                    }
                    n278 = Multiply(x=w345, y=w349) -> (x*y=w351:dbl)
                    n279 = Divide(x=w351, y=60.0) -> (x/y=w344:dbl)
                    n280 = Bundle(cluster=w347, "CYCLE"=w345, "MINS"=w344) -> (w346:T4)  [unwired: 1 in]
                    n281 = local write "DISP LAB04-2"(w346) -> ()
                  }
                  frame #8 {
                    # "update cycle value"
                    # "LAB05-1"
                    n282 = local read "DISP LAB05-1"() -> (w359:T4)
                    n283 = Unbundle(w359) -> ("CYCLE"=w360:dbl)  [unwired: 2 out]
                    n284 = case shown="True" w364 {
                      tunnel: [w365 w367] -> w357
                      tunnel: w360 -> [w365 w366]
                      frame False {
                      }
                      frame True {
                        n285 = Increment(x=w366) -> (x+1=w367:dbl)
                      }
                    }
                    n286 = Multiply(x=w357, y=w361) -> (x*y=w362:dbl)
                    n287 = Divide(x=w362, y=60.0) -> (x/y=w356:dbl)
                    n288 = Bundle(cluster=w359, "CYCLE"=w357, "MINS"=w356) -> (w358:T4)  [unwired: 1 in]
                    n289 = local write "DISP LAB05-1"(w358) -> ()
                  }
                  frame #9 {
                    # "update cycle value"
                    # "LAB05-2"
                    n290 = local read "DISP LAB05-2"() -> (w372:T4)
                    n291 = Unbundle(w372) -> ("CYCLE"=w371:dbl)  [unwired: 2 out]
                    n292 = case shown="True" w376 {
                      tunnel: [w377 w379] -> w370
                      tunnel: w371 -> [w377 w378]
                      frame False {
                      }
                      frame True {
                        n293 = Increment(x=w378) -> (x+1=w379:dbl)
                      }
                    }
                    n294 = Multiply(x=w370, y=w373) -> (x*y=w374:dbl)
                    n295 = Divide(x=w374, y=60.0) -> (x/y=w369:dbl)
                    n296 = Bundle(cluster=w372, "CYCLE"=w370, "MINS"=w369) -> (w368:T4)  [unwired: 1 in]
                    n297 = local write "DISP LAB05-2"(w368) -> ()
                  }
                }
                n298 = local write "jig cycle"(0) -> ()
              }
            }
          }
          frame #3 {
            (unwired) "c:\\BAT\\labdatav2\\"
            # "START & STOP test RUN switch change, start test if true and stop test if false"
            n299 = Get Date/Time In Seconds() -> (seconds since 1Jan1904=w387:timestamp)
            n300 = local read "C drive data root dir"() -> (w380:path)
            n301 = Format Date/Time String(time format string (%c)="%b%d", seconds (now)=w387) -> (date/time string=w411:string)  [unwired: 1 in]
            n302 = Format Date/Time String(time format string (%c)="%H%M", seconds (now)=w387) -> (date/time string=w409:string)  [unwired: 1 in]
            n303 = Format Date/Time String(time format string (%c)="%Y", seconds (now)=w387) -> (date/time string=w386:string)  [unwired: 1 in]
            n304 = Path To String(path=w380) -> (string=w383:string)
            n305 = global write "Global 1.vi" "C drive root path"(w380) -> ()
            n306 = Concatenate Strings(w383, "\\") -> (w381:string)
            n307 = event shown="[1] \"RUN LAB01-1\": Value Change" {
              selector: _ -> [_ _ _ _ _ _ _ _ _ _ _]
              dyn-events: _ -> [_ _ _ _ _ _ _ _ _ _ _]
              timeout: 10 -> [_ _ _ _ _ _ _ _ _ _ _]
              tunnel: w381 -> [_ w419 w479 w539 w599 w659 w719 w778 w838 w898 w958]
              tunnel: w411 -> [_ w418 w478 w538 w598 w658 w718 w777 w837 w897 w957]
              tunnel: w409 -> [_ w416 w476 w537 w597 w657 w717 w776 w836 w896 w956]
              tunnel: w407 -> [_ w417 w477 _ _ _ _ _ _ _ _]
              tunnel: w408 -> [_ _ _ _ _ _ _ _ _ _ _]
              tunnel: w406 -> [_ _ _ _ _ _ _ _ _ _ _]
              tunnel: w405 -> [_ _ _ _ _ _ _ _ _ _ _]
              tunnel: w404 -> [_ _ _ _ _ _ _ _ _ _ _]
              tunnel: w403 -> [_ _ _ w536 _ _ _ _ _ _ _]
              tunnel: w402 -> [_ _ _ _ _ _ _ _ _ _ _]
              tunnel: w401 -> [_ _ _ _ w596 _ _ _ _ _ _]
              tunnel: w400 -> [_ _ _ _ _ _ _ _ _ _ _]
              tunnel: w399 -> [_ _ _ _ _ w656 _ _ _ _ _]
              tunnel: w398 -> [_ _ _ _ _ _ _ _ _ _ _]
              tunnel: w397 -> [_ _ _ _ _ _ w716 _ _ _ _]
              tunnel: w396 -> [_ _ _ _ _ _ _ _ _ _ _]
              tunnel: w395 -> [_ _ _ _ _ _ _ w775 _ _ _]
              tunnel: w394 -> [_ _ _ _ _ _ _ _ _ _ _]
              tunnel: w393 -> [_ _ _ _ _ _ _ _ w835 _ _]
              tunnel: w392 -> [_ _ _ _ _ _ _ _ _ _ _]
              tunnel: w391 -> [_ _ _ _ _ _ _ _ _ w895 _]
              tunnel: w390 -> [_ _ _ _ _ _ _ _ _ _ _]
              tunnel: w389 -> [_ _ _ _ _ _ _ _ _ _ w955]
              tunnel: w386 -> [_ w415 w475 w535 w595 w655 w715 w774 w834 w894 w954]
              tunnel: [_ w414 w474 w534 w594 w654 w714 w773 w833 w893 w953] -> w384
              event Timeout {
                n308 = event-data() -> ()  [unwired: 1 in, 3 out]
              }
              event "RUN LAB01-1": Value Change {
                n309 = event-data() -> ("NewVal"=w413:bool)  [unwired: 1 in, 5 out]
                n310 = local write "run lab01-1"(w413) -> ()
                n311 = case shown="True" w413 {
                  tunnel: w419 -> [_ w435]
                  tunnel: w418 -> [_ w434]
                  tunnel: w417 -> [w421 w433]
                  tunnel: w416 -> [_ w432]
                  tunnel: w415 -> [_ w431]
                  tunnel: [w420 w430] -> w414
                  frame False {
                    # "stop test"
                    n312 = stacked-sequence {
                      tunnel: w421 -> [_ _ _]
                      tunnel: [_ w426 _] -> w420
                      frame #0 {
                        n313 = local read "DISP LAB01-1"() -> (w424:T4)
                        n314 = Bundle(cluster=w424, "STATUS"="STOP") -> (w422:T4)  [unwired: 2 in]
                        n315 = local write "DISP LAB01-1"(w422) -> ()
                      }
                      frame #1 {
                        n316 = local read "DATA LAB01-1"() -> (w425:refnum<k1>)
                        n317 = Close File(refnum=w425) -> (error out=w426:errorcluster)  [unwired: 1 in, 1 out]
                      }
                      frame #2 {
                        n318 = call "Save data file to network drive v1.vi"("panel id"="LAB01-1") -> ("network file save error"=w427:errorcluster)  [unwired: 9 in, 1 out]
                        n319 = local write "RESULT LAB01-1"(FALSE) -> ()
                        n320 = local write "data file error"(w427) -> ()
                      }
                    }
                  }
                  frame True {
                    # "start new test and create test file"
                    n321 = stacked-sequence {
                      seq-local: [w436 _ _ _] -> [_ w463 _ _]
                      tunnel: w435 -> [w441 _ _ _]
                      tunnel: w434 -> [w437 _ _ _]
                      tunnel: w433 -> [w451 _ _ _]
                      tunnel: w432 -> [w444 _ _ _]
                      tunnel: w431 -> [w439 _ _ _]
                      tunnel: [_ w455 _ _] -> w430
                      frame #0 {
                        w438 = "\\"
                        n322 = local read "SET LAB01-1"() -> (w446:T5)
                        n323 = case shown="\"CHART TEST\", Default" w451 {
                          tunnel: ["CHART TEST-" "CYCLE TEST-" "T-RISE TEST-"] -> w447
                          frame "CHART TEST", Default {
                          }
                          frame "CYCLE TEST" {
                          }
                          frame "T-RISE TEST" {
                          }
                        }
                        n324 = Unbundle(w446) -> ("DESCRIPTION"=w445:string)  [unwired: 4 out]
                        n325 = Concatenate Strings(w441, "LAB01-1\\", w439, w438, w437, w438) -> (w448:string)
                        n326 = String To Path(string=w448) -> (path=w450:path)
                        n327 = Concatenate Strings(w448, w447, w445, "-", w444, ".dat") -> (w436:string)
                        n328 = Create Folder(path (use dialog)=w450) -> (error out=w449:errorcluster)  [unwired: 2 in, 2 out]
                        n329 = call <vilib>:"Clear Errors.vi"("error in (no error)"=w449) -> ()  [unwired: 6 in, 1 out]
                        n330 = global write "Global 1.vi" "LAB01-1 FILE"(w436) -> ()
                      }
                      frame #1 {
                        n331 = local read "SET LAB01-1"() -> (w461:T5)
                        n332 = local read "DISP LAB01-1"() -> (w459:T4)
                        n333 = local read "SIG LAB01-1"() -> (w460:T2)
                        n334 = Bundle("SET LAB01-1"=w461, "SIG LAB01-1"=w460, "DISP LAB01-1"=w459) -> (w458:T18)  [unwired: 1 in]
                        n335 = String To Path(string=w463) -> (path=w456:path)
                        n336 = Open/Create/Replace Datalog(5:w458, 10:T15."replace or create" ("operation (0:open)"), 11:w456) -> (0:w455:errorcluster, 3:→"DATA LAB01-1":refnum<k1>)  [unwired: 3 in, 1 out]
                      }
                      frame #2 {
                        w464 = 0.0
                        n337 = local read "DISP LAB01-1"() -> (w467:T4)
                        n338 = Bundle(cluster=w467, "CYCLE"=w464, "MINS"=w464, "STATUS"="RUN") -> (w466:T4)
                        n339 = local write "DISP LAB01-1"(w466) -> ()
                      }
                      frame #3 {
                        n340 = local read "SIG LAB01-1"() -> (w470:T2)
                        n341 = local read "TEMP START LAB01-1"() -> (w472:cluster{"TL":dbl, "TN":dbl})
                        n342 = Unbundle(w470) -> ("Tmp Live"=w469:dbl, "Tmp Neut"=w468:dbl)  [unwired: 3 out]
                        n343 = Bundle(cluster=w472, "TL"=w469, "TN"=w468) -> (w471:cluster{"TL":dbl, "TN":dbl})
                        n344 = local write "TEMP START LAB01-1"(w471) -> ()
                      }
                    }
                  }
                }
              }
              event "RUN LAB01-2": Value Change {
                n345 = event-data() -> ("NewVal"=w473:bool)  [unwired: 1 in, 5 out]
                n346 = local write "run lab01-2"(w473) -> ()
                n347 = case shown="True" w473 {
                  tunnel: w479 -> [_ w495]
                  tunnel: w478 -> [_ w494]
                  tunnel: w477 -> [w481 w493]
                  tunnel: w476 -> [_ w492]
                  tunnel: w475 -> [_ w491]
                  tunnel: [w480 w490] -> w474
                  frame False {
                    # "stop test"
                    n348 = stacked-sequence {
                      tunnel: w481 -> [_ _ _]
                      tunnel: [_ w485 _] -> w480
                      frame #0 {
                        n349 = local read "DISP LAB01-2"() -> (w484:T4)
                        n350 = Bundle(cluster=w484, "STATUS"="STOP") -> (w482:T4)  [unwired: 2 in]
                        n351 = local write "DISP LAB01-2"(w482) -> ()
                      }
                      frame #1 {
                        n352 = local read "DATA LAB01-2"() -> (w486:refnum<k1>)
                        n353 = Close File(refnum=w486) -> (error out=w485:errorcluster)  [unwired: 1 in, 1 out]
                      }
                      frame #2 {
                        n354 = call "Save data file to network drive v1.vi"("panel id"="LAB01-2") -> ("network file save error"=w487:errorcluster)  [unwired: 9 in, 1 out]
                        n355 = local write "RESULT LAB01-2"(FALSE) -> ()
                        n356 = local write "data file error"(w487) -> ()
                      }
                    }
                  }
                  frame True {
                    # "start new test and create test file"
                    n357 = stacked-sequence {
                      seq-local: [w496 _ _ _] -> [_ w523 _ _]
                      tunnel: w495 -> [w501 _ _ _]
                      tunnel: w494 -> [w497 _ _ _]
                      tunnel: w493 -> [w511 _ _ _]
                      tunnel: w492 -> [w504 _ _ _]
                      tunnel: w491 -> [w499 _ _ _]
                      tunnel: [_ w516 _ _] -> w490
                      frame #0 {
                        w498 = "\\"
                        n358 = local read "SET LAB01-2"() -> (w506:T5)
                        n359 = case shown="\"CHART TEST\", Default" w511 {
                          tunnel: ["CHART TEST-" "CYCLE TEST-" "T-RISE TEST-"] -> w507
                          frame "CHART TEST", Default {
                          }
                          frame "CYCLE TEST" {
                          }
                          frame "T-RISE TEST" {
                          }
                        }
                        n360 = Unbundle(w506) -> ("DESCRIPTION"=w505:string)  [unwired: 4 out]
                        n361 = Concatenate Strings(w501, "LAB01-2\\", w499, w498, w497, w498) -> (w508:string)
                        n362 = String To Path(string=w508) -> (path=w510:path)
                        n363 = Concatenate Strings(w508, w507, w505, "-", w504, ".dat") -> (w496:string)
                        n364 = Create Folder(path (use dialog)=w510) -> (error out=w509:errorcluster)  [unwired: 2 in, 2 out]
                        n365 = call <vilib>:"Clear Errors.vi"("error in (no error)"=w509) -> ()  [unwired: 6 in, 1 out]
                        n366 = global write "Global 1.vi" "LAB01-2 FILE"(w496) -> ()
                      }
                      frame #1 {
                        n367 = local read "SET LAB01-1"() -> (w521:T5)
                        n368 = local read "DISP LAB01-1"() -> (w519:T4)
                        n369 = local read "SIG LAB01-1"() -> (w520:T2)
                        n370 = Bundle("SET LAB01-1"=w521, "SIG LAB01-1"=w520, "DISP LAB01-1"=w519) -> (w518:T18)  [unwired: 1 in]
                        n371 = String To Path(string=w523) -> (path=w517:path)
                        n372 = Open/Create/Replace Datalog(5:w518, 10:T15."replace or create" ("operation (0:open)"), 11:w517) -> (0:w516:errorcluster, 3:→"DATA LAB01-2":refnum<k1>)  [unwired: 3 in, 1 out]
                      }
                      frame #2 {
                        w524 = 0.0
                        n373 = local read "DISP LAB01-1"() -> (w527:T4)
                        n374 = Bundle(cluster=w527, "CYCLE"=w524, "MINS"=w524, "STATUS"="RUN") -> (w526:T4)
                        n375 = local write "DISP LAB01-1"(w526) -> ()
                      }
                      frame #3 {
                        n376 = local read "SIG LAB01-1"() -> (w530:T2)
                        n377 = local read "TEMP START LAB01-1"() -> (w532:cluster{"TL":dbl, "TN":dbl})
                        n378 = Unbundle(w530) -> ("Tmp Live"=w529:dbl, "Tmp Neut"=w528:dbl)  [unwired: 3 out]
                        n379 = Bundle(cluster=w532, "TL"=w529, "TN"=w528) -> (w531:cluster{"TL":dbl, "TN":dbl})
                        n380 = local write "TEMP START LAB01-1"(w531) -> ()
                      }
                    }
                  }
                }
              }
              event "RUN LAB02-1": Value Change {
                n381 = event-data() -> ("NewVal"=w533:bool)  [unwired: 1 in, 5 out]
                n382 = local write "run lab02-1"(w533) -> ()
                n383 = case shown="True" w533 {
                  tunnel: w539 -> [_ w555]
                  tunnel: w538 -> [_ w554]
                  tunnel: w536 -> [w541 w553]
                  tunnel: w537 -> [_ w552]
                  tunnel: w535 -> [_ w551]
                  tunnel: [w540 w550] -> w534
                  frame False {
                    # "stop test"
                    n384 = stacked-sequence {
                      tunnel: w541 -> [_ _]
                      tunnel: [_ w546] -> w540
                      frame #0 {
                        n385 = local read "DISP LAB02-1"() -> (w544:T4)
                        n386 = Bundle(cluster=w544, "STATUS"="STOP") -> (w542:T4)  [unwired: 2 in]
                        n387 = local write "DISP LAB02-1"(w542) -> ()
                      }
                      frame #1 {
                        n388 = local read "DATA LAB02-1"() -> (w545:refnum<k1>)
                        n389 = Close File(refnum=w545) -> (error out=w546:errorcluster)  [unwired: 1 in, 1 out]
                        n390 = local write "RESULT LAB02-1"(FALSE) -> ()
                        n391 = call "Save data file to network drive v1.vi"("panel id"="LAB02-1") -> ("network file save error"=w547:errorcluster)  [unwired: 9 in, 1 out]
                        n392 = local write "data file error"(w547) -> ()
                      }
                    }
                  }
                  frame True {
                    # "start new test and create test file"
                    n393 = stacked-sequence {
                      seq-local: [w556 _ _ _] -> [_ w583 _ _]
                      tunnel: w555 -> [w561 _ _ _]
                      tunnel: w554 -> [w558 _ _ _]
                      tunnel: w553 -> [w571 _ _ _]
                      tunnel: w552 -> [w564 _ _ _]
                      tunnel: w551 -> [w559 _ _ _]
                      tunnel: [_ w576 _ _] -> w550
                      frame #0 {
                        w557 = "\\"
                        n394 = local read "SET LAB02-1"() -> (w566:T5)
                        n395 = case shown="\"CHART TEST\", Default" w571 {
                          tunnel: ["CHART TEST-" "CYCLE TEST-" "T-RISE TEST-"] -> w567
                          frame "CHART TEST", Default {
                          }
                          frame "CYCLE TEST" {
                          }
                          frame "T-RISE TEST" {
                          }
                        }
                        n396 = Unbundle(w566) -> ("DESCRIPTION"=w565:string)  [unwired: 4 out]
                        n397 = Concatenate Strings(w561, "LAB02-1\\", w559, w557, w558, w557) -> (w568:string)
                        n398 = String To Path(string=w568) -> (path=w570:path)
                        n399 = Concatenate Strings(w568, w567, w565, "-", w564, ".dat") -> (w556:string)
                        n400 = Create Folder(path (use dialog)=w570) -> (error out=w569:errorcluster)  [unwired: 2 in, 2 out]
                        n401 = global write "Global 1.vi" "LAB02-1 FILE"(w556) -> ()
                        n402 = call <vilib>:"Clear Errors.vi"("error in (no error)"=w569) -> ()  [unwired: 6 in, 1 out]
                      }
                      frame #1 {
                        n403 = local read "DISP LAB02-1"() -> (w580:T4)
                        n404 = local read "SET LAB02-1"() -> (w582:T5)
                        n405 = local read "SIG LAB02-1"() -> (w581:T2)
                        n406 = String To Path(string=w583) -> (path=w579:path)
                        n407 = Bundle("SET LAB02-1"=w582, "SIG LAB02-1"=w581, "DISP LAB02-1"=w580) -> (w578:T19)  [unwired: 1 in]
                        n408 = Open/Create/Replace Datalog(5:w578, 10:T15."open or create" ("operation (0:open)"), 11:w579) -> (0:w576:errorcluster, 3:→"DATA LAB02-1":refnum<k1>)  [unwired: 3 in, 1 out]
                      }
                      frame #2 {
                        w585 = 0.0
                        n409 = local read "DISP LAB02-1"() -> (w587:T4)
                        n410 = Bundle(cluster=w587, "CYCLE"=w585, "MINS"=w585, "STATUS"="RUN") -> (w586:T4)
                        n411 = local write "DISP LAB02-1"(w586) -> ()
                      }
                      frame #3 {
                        n412 = local read "SIG LAB02-1"() -> (w590:T2)
                        n413 = local read "TEMP START LAB02-1"() -> (w592:cluster{"TL":dbl, "TN":dbl})
                        n414 = Unbundle(w590) -> ("Tmp Live"=w589:dbl, "Tmp Neut"=w588:dbl)  [unwired: 3 out]
                        n415 = Bundle(cluster=w592, "TL"=w589, "TN"=w588) -> (w591:cluster{"TL":dbl, "TN":dbl})
                        n416 = local write "TEMP START LAB02-1"(w591) -> ()
                      }
                    }
                  }
                }
              }
              event "RUN LAB02-2": Value Change {
                n417 = event-data() -> ("NewVal"=w593:bool)  [unwired: 1 in, 5 out]
                n418 = local write "run lab02-2"(w593) -> ()
                n419 = case shown="False" w593 {
                  tunnel: w599 -> [_ w615]
                  tunnel: w598 -> [_ w614]
                  tunnel: w596 -> [w601 w613]
                  tunnel: w597 -> [_ w612]
                  tunnel: w595 -> [_ w611]
                  tunnel: [w600 w610] -> w594
                  frame False {
                    # "stop test"
                    n420 = stacked-sequence {
                      tunnel: w601 -> [_ _]
                      tunnel: [_ w605] -> w600
                      frame #0 {
                        n421 = local read "DISP LAB02-2"() -> (w604:T4)
                        n422 = Bundle(cluster=w604, "STATUS"="STOP") -> (w602:T4)  [unwired: 2 in]
                        n423 = local write "DISP LAB02-2"(w602) -> ()
                      }
                      frame #1 {
                        n424 = local read "DATA LAB02-2"() -> (w606:refnum<k1>)
                        n425 = call "Save data file to network drive v1.vi"("panel id"="LAB02-2") -> ("network file save error"=w607:errorcluster)  [unwired: 9 in, 1 out]
                        n426 = local write "RESULT LAB02-2"(FALSE) -> ()
                        n427 = local write "data file error"(w607) -> ()
                        n428 = Close File(refnum=w606) -> (error out=w605:errorcluster)  [unwired: 1 in, 1 out]
                      }
                    }
                  }
                  frame True {
                    # "start new test and create test file"
                    n429 = stacked-sequence {
                      seq-local: [w616 _ _ _] -> [_ w643 _ _]
                      tunnel: w615 -> [w621 _ _ _]
                      tunnel: w614 -> [w618 _ _ _]
                      tunnel: w613 -> [w631 _ _ _]
                      tunnel: w612 -> [w624 _ _ _]
                      tunnel: w611 -> [w619 _ _ _]
                      tunnel: [_ w635 _ _] -> w610
                      frame #0 {
                        w617 = "\\"
                        n430 = local read "SET LAB02-2"() -> (w626:T5)
                        n431 = case shown="\"CHART TEST\", Default" w631 {
                          tunnel: ["CHART TEST-" "CYCLE TEST-" "T-RISE TEST-"] -> w627
                          frame "CHART TEST", Default {
                          }
                          frame "CYCLE TEST" {
                          }
                          frame "T-RISE TEST" {
                          }
                        }
                        n432 = Unbundle(w626) -> ("DESCRIPTION"=w625:string)  [unwired: 4 out]
                        n433 = Concatenate Strings(w621, "LAB02-2\\", w619, w617, w618, w617) -> (w628:string)
                        n434 = String To Path(string=w628) -> (path=w630:path)
                        n435 = Concatenate Strings(w628, w627, w625, "-", w624, ".dat") -> (w616:string)
                        n436 = Create Folder(path (use dialog)=w630) -> (error out=w629:errorcluster)  [unwired: 2 in, 2 out]
                        n437 = global write "Global 1.vi" "LAB02-2 FILE"(w616) -> ()
                        n438 = call <vilib>:"Clear Errors.vi"("error in (no error)"=w629) -> ()  [unwired: 6 in, 1 out]
                      }
                      frame #1 {
                        n439 = local read "SET LAB02-2"() -> (w642:T5)
                        n440 = local read "DISP LAB02-2"() -> (w640:T4)
                        n441 = local read "SIG LAB02-2"() -> (w641:T2)
                        n442 = String To Path(string=w643) -> (path=w638:path)
                        n443 = Bundle("SET LAB02-2"=w642, "SIG LAB02-2"=w641, "DISP LAB02-2"=w640) -> (w637:T20)  [unwired: 1 in]
                        n444 = Open/Create/Replace Datalog(5:w637, 10:T15."open or create" ("operation (0:open)"), 11:w638) -> (0:w635:errorcluster, 3:→"DATA LAB02-2":refnum<k1>)  [unwired: 3 in, 1 out]
                      }
                      frame #2 {
                        w645 = 0.0
                        n445 = local read "DISP LAB02-2"() -> (w647:T4)
                        n446 = Bundle(cluster=w647, "CYCLE"=w645, "MINS"=w645, "STATUS"="RUN") -> (w646:T4)
                        n447 = local write "DISP LAB02-2"(w646) -> ()
                      }
                      frame #3 {
                        n448 = local read "SIG LAB02-2"() -> (w650:T2)
                        n449 = local read "TEMP START LAB02-2"() -> (w652:cluster{"TL":dbl, "TN":dbl})
                        n450 = Unbundle(w650) -> ("Tmp Live"=w649:dbl, "Tmp Neut"=w648:dbl)  [unwired: 3 out]
                        n451 = Bundle(cluster=w652, "TL"=w649, "TN"=w648) -> (w651:cluster{"TL":dbl, "TN":dbl})
                        n452 = local write "TEMP START LAB02-2"(w651) -> ()
                      }
                    }
                  }
                }
              }
              event "RUN LAB03-1": Value Change {
                n453 = event-data() -> ("NewVal"=w653:bool)  [unwired: 1 in, 5 out]
                n454 = local write "run lab03-1"(w653) -> ()
                n455 = case shown="False" w653 {
                  tunnel: w659 -> [_ w675]
                  tunnel: w658 -> [_ w674]
                  tunnel: w656 -> [w661 w673]
                  tunnel: w657 -> [_ w672]
                  tunnel: w655 -> [_ w671]
                  tunnel: [w660 w670] -> w654
                  frame False {
                    # "stop test"
                    n456 = stacked-sequence {
                      tunnel: w661 -> [_ _]
                      tunnel: [_ w665] -> w660
                      frame #0 {
                        n457 = local read "DISP LAB03-1"() -> (w664:T4)
                        n458 = Bundle(cluster=w664, "STATUS"="STOP") -> (w662:T4)  [unwired: 2 in]
                        n459 = local write "DISP LAB03-1"(w662) -> ()
                      }
                      frame #1 {
                        n460 = local read "DATA LAB03-1"() -> (w666:refnum<k1>)
                        n461 = call "Save data file to network drive v1.vi"("panel id"="LAB03-1") -> ("network file save error"=w667:errorcluster)  [unwired: 9 in, 1 out]
                        n462 = local write "RESULT LAB03-1"(FALSE) -> ()
                        n463 = local write "data file error"(w667) -> ()
                        n464 = Close File(refnum=w666) -> (error out=w665:errorcluster)  [unwired: 1 in, 1 out]
                      }
                    }
                  }
                  frame True {
                    # "start new test and create test file"
                    n465 = stacked-sequence {
                      seq-local: [w676 _ _ _] -> [_ w703 _ _]
                      tunnel: w675 -> [w681 _ _ _]
                      tunnel: w674 -> [w678 _ _ _]
                      tunnel: w673 -> [w691 _ _ _]
                      tunnel: w672 -> [w684 _ _ _]
                      tunnel: w671 -> [w679 _ _ _]
                      tunnel: [_ w695 _ _] -> w670
                      frame #0 {
                        w677 = "\\"
                        n466 = local read "SET LAB03-1"() -> (w686:T5)
                        n467 = case shown="\"CHART TEST\", Default" w691 {
                          tunnel: ["CHART TEST-" "CYCLE TEST-" "T-RISE TEST-"] -> w687
                          frame "CHART TEST", Default {
                          }
                          frame "CYCLE TEST" {
                          }
                          frame "T-RISE TEST" {
                          }
                        }
                        n468 = Unbundle(w686) -> ("DESCRIPTION"=w685:string)  [unwired: 4 out]
                        n469 = Concatenate Strings(w681, "LAB03-1\\", w679, w677, w678, w677) -> (w688:string)
                        n470 = String To Path(string=w688) -> (path=w690:path)
                        n471 = Concatenate Strings(w688, w687, w685, "-", w684, ".dat") -> (w676:string)
                        n472 = Create Folder(path (use dialog)=w690) -> (error out=w689:errorcluster)  [unwired: 2 in, 2 out]
                        n473 = global write "Global 1.vi" "LAB03-1 FILE"(w676) -> ()
                        n474 = call <vilib>:"Clear Errors.vi"("error in (no error)"=w689) -> ()  [unwired: 6 in, 1 out]
                      }
                      frame #1 {
                        n475 = local read "DISP LAB03-1"() -> (w700:T4)
                        n476 = local read "SIG LAB03-1"() -> (w701:T2)
                        n477 = local read "SET LAB03-1"() -> (w702:T5)
                        n478 = String To Path(string=w703) -> (path=w699:path)
                        n479 = Bundle("SET LAB03-1"=w702, "SIG LAB03-1"=w701, "DISP LAB03-1"=w700) -> (w698:T21)  [unwired: 1 in]
                        n480 = Open/Create/Replace Datalog(5:w698, 10:T15."open or create" ("operation (0:open)"), 11:w699) -> (0:w695:errorcluster, 3:→"DATA LAB03-1":refnum<k1>)  [unwired: 3 in, 1 out]
                      }
                      frame #2 {
                        w705 = 0.0
                        n481 = local read "DISP LAB03-1"() -> (w707:T4)
                        n482 = Bundle(cluster=w707, "CYCLE"=w705, "MINS"=w705, "STATUS"="RUN") -> (w706:T4)
                        n483 = local write "DISP LAB03-1"(w706) -> ()
                      }
                      frame #3 {
                        n484 = local read "SIG LAB03-1"() -> (w710:T2)
                        n485 = local read "TEMP START LAB03-1"() -> (w712:cluster{"TL":dbl, "TN":dbl})
                        n486 = Unbundle(w710) -> ("Tmp Live"=w709:dbl, "Tmp Neut"=w708:dbl)  [unwired: 3 out]
                        n487 = Bundle(cluster=w712, "TL"=w709, "TN"=w708) -> (w711:cluster{"TL":dbl, "TN":dbl})
                        n488 = local write "TEMP START LAB03-1"(w711) -> ()
                      }
                    }
                  }
                }
              }
              event "RUN LAB03-2": Value Change {
                n489 = event-data() -> ("NewVal"=w713:bool)  [unwired: 1 in, 5 out]
                n490 = local write "run lab03-2"(w713) -> ()
                n491 = case shown="False" w713 {
                  tunnel: w719 -> [_ w735]
                  tunnel: w718 -> [_ w734]
                  tunnel: w716 -> [w721 w733]
                  tunnel: w717 -> [_ w732]
                  tunnel: w715 -> [_ w731]
                  tunnel: [w720 w730] -> w714
                  frame False {
                    # "stop test"
                    n492 = stacked-sequence {
                      tunnel: w721 -> [_ _]
                      tunnel: [_ w725] -> w720
                      frame #0 {
                        n493 = local read "DISP LAB03-2"() -> (w724:T4)
                        n494 = Bundle(cluster=w724, "STATUS"="STOP") -> (w722:T4)  [unwired: 2 in]
                        n495 = local write "DISP LAB03-2"(w722) -> ()
                      }
                      frame #1 {
                        n496 = local read "DATA LAB03-2"() -> (w726:refnum<k1>)
                        n497 = call "Save data file to network drive v1.vi"("panel id"="LAB03-2") -> ("network file save error"=w727:errorcluster)  [unwired: 9 in, 1 out]
                        n498 = local write "RESULT LAB03-2"(FALSE) -> ()
                        n499 = local write "data file error"(w727) -> ()
                        n500 = Close File(refnum=w726) -> (error out=w725:errorcluster)  [unwired: 1 in, 1 out]
                      }
                    }
                  }
                  frame True {
                    # "start new test and create test file"
                    n501 = stacked-sequence {
                      seq-local: [w736 _ _ _] -> [_ w762 _ _]
                      tunnel: w735 -> [w741 _ _ _]
                      tunnel: w734 -> [w738 _ _ _]
                      tunnel: w733 -> [w751 _ _ _]
                      tunnel: w732 -> [w744 _ _ _]
                      tunnel: w731 -> [w739 _ _ _]
                      tunnel: [_ w755 _ _] -> w730
                      frame #0 {
                        w737 = "\\"
                        n502 = local read "SET LAB03-2"() -> (w746:T5)
                        n503 = case shown="\"CHART TEST\", Default" w751 {
                          tunnel: ["CHART TEST-" "CYCLE TEST-" "T-RISE TEST-"] -> w747
                          frame "CHART TEST", Default {
                          }
                          frame "CYCLE TEST" {
                          }
                          frame "T-RISE TEST" {
                          }
                        }
                        n504 = Unbundle(w746) -> ("DESCRIPTION"=w745:string)  [unwired: 4 out]
                        n505 = Concatenate Strings(w741, "LAB03-2\\", w739, w737, w738, w737) -> (w748:string)
                        n506 = String To Path(string=w748) -> (path=w750:path)
                        n507 = Concatenate Strings(w748, w747, w745, "-", w744, ".dat") -> (w736:string)
                        n508 = Create Folder(path (use dialog)=w750) -> (error out=w749:errorcluster)  [unwired: 2 in, 2 out]
                        n509 = global write "Global 1.vi" "LAB03-2 FILE"(w736) -> ()
                        n510 = call <vilib>:"Clear Errors.vi"("error in (no error)"=w749) -> ()  [unwired: 6 in, 1 out]
                      }
                      frame #1 {
                        n511 = local read "DISP LAB03-2"() -> (w759:T4)
                        n512 = local read "SET LAB03-2"() -> (w761:T5)
                        n513 = local read "SIG LAB03-2"() -> (w760:T2)
                        n514 = String To Path(string=w762) -> (path=w756:path)
                        n515 = Bundle("SET LAB03-2"=w761, "SIG LAB03-2"=w760, "DISP LAB03-2"=w759) -> (w757:T22)  [unwired: 1 in]
                        n516 = Open/Create/Replace Datalog(5:w757, 10:T15."open or create" ("operation (0:open)"), 11:w756) -> (0:w755:errorcluster)  [unwired: 3 in, 2 out]
                      }
                      frame #2 {
                        w764 = 0.0
                        n517 = local read "DISP LAB03-2"() -> (w766:T4)
                        n518 = Bundle(cluster=w766, "CYCLE"=w764, "MINS"=w764, "STATUS"="RUN") -> (w765:T4)
                        n519 = local write "DISP LAB03-2"(w765) -> ()
                      }
                      frame #3 {
                        n520 = local read "SIG LAB03-2"() -> (w769:T2)
                        n521 = local read "TEMP START LAB03-2"() -> (w771:cluster{"TL":dbl, "TN":dbl})
                        n522 = Unbundle(w769) -> ("Tmp Live"=w768:dbl, "Tmp Neut"=w767:dbl)  [unwired: 3 out]
                        n523 = Bundle(cluster=w771, "TL"=w768, "TN"=w767) -> (w770:cluster{"TL":dbl, "TN":dbl})
                        n524 = local write "TEMP START LAB03-2"(w770) -> ()
                      }
                    }
                  }
                }
              }
              event "RUN LAB04-1": Value Change {
                n525 = event-data() -> ("NewVal"=w772:bool)  [unwired: 1 in, 5 out]
                n526 = local write "run lab04-1"(w772) -> ()
                n527 = case shown="False" w772 {
                  tunnel: w778 -> [_ w794]
                  tunnel: w777 -> [_ w793]
                  tunnel: w775 -> [w780 w792]
                  tunnel: w776 -> [_ w791]
                  tunnel: w774 -> [_ w790]
                  tunnel: [w779 w789] -> w773
                  frame False {
                    # "stop test"
                    n528 = stacked-sequence {
                      tunnel: w780 -> [_ _]
                      tunnel: [_ w784] -> w779
                      frame #0 {
                        n529 = local read "DISP LAB04-1"() -> (w783:T4)
                        n530 = Bundle(cluster=w783, "STATUS"="STOP") -> (w781:T4)  [unwired: 2 in]
                        n531 = local write "DISP LAB04-1"(w781) -> ()
                      }
                      frame #1 {
                        n532 = local read "DATA LAB04-1"() -> (w785:refnum<k1>)
                        n533 = call "Save data file to network drive v1.vi"("panel id"="LAB04-1") -> ("network file save error"=w786:errorcluster)  [unwired: 9 in, 1 out]
                        n534 = local write "RESULT LAB04-1"(FALSE) -> ()
                        n535 = local write "data file error"(w786) -> ()
                        n536 = Close File(refnum=w785) -> (error out=w784:errorcluster)  [unwired: 1 in, 1 out]
                      }
                    }
                  }
                  frame True {
                    # "start new test and create test file"
                    n537 = stacked-sequence {
                      seq-local: [w795 _ _ _] -> [_ w822 _ _]
                      tunnel: w794 -> [w800 _ _ _]
                      tunnel: w793 -> [w796 _ _ _]
                      tunnel: w792 -> [w810 _ _ _]
                      tunnel: w791 -> [w803 _ _ _]
                      tunnel: w790 -> [w798 _ _ _]
                      tunnel: [_ w815 _ _] -> w789
                      frame #0 {
                        w797 = "\\"
                        n538 = local read "SET LAB04-1"() -> (w805:T5)
                        n539 = case shown="\"CHART TEST\", Default" w810 {
                          tunnel: ["CHART TEST-" "CYCLE TEST-" "T-RISE TEST-"] -> w806
                          frame "CHART TEST", Default {
                          }
                          frame "CYCLE TEST" {
                          }
                          frame "T-RISE TEST" {
                          }
                        }
                        n540 = Unbundle(w805) -> ("DESCRIPTION"=w804:string)  [unwired: 4 out]
                        n541 = Concatenate Strings(w800, "LAB04-1\\", w798, w797, w796, w797) -> (w807:string)
                        n542 = String To Path(string=w807) -> (path=w809:path)
                        n543 = Concatenate Strings(w807, w806, w804, "-", w803, ".dat") -> (w795:string)
                        n544 = Create Folder(path (use dialog)=w809) -> (error out=w808:errorcluster)  [unwired: 2 in, 2 out]
                        n545 = global write "Global 1.vi" "LAB04-1 FILE"(w795) -> ()
                        n546 = call <vilib>:"Clear Errors.vi"("error in (no error)"=w808) -> ()  [unwired: 6 in, 1 out]
                      }
                      frame #1 {
                        n547 = local read "DISP LAB04-1"() -> (w819:T4)
                        n548 = local read "SET LAB04-1"() -> (w821:T5)
                        n549 = local read "SIG LAB04-1"() -> (w820:T2)
                        n550 = String To Path(string=w822) -> (path=w816:path)
                        n551 = Bundle("SET LAB04-1"=w821, "SIG LAB04-1"=w820, "DISP LAB04-1"=w819) -> (w817:T23)  [unwired: 1 in]
                        n552 = Open/Create/Replace Datalog(5:w817, 10:T15."open or create" ("operation (0:open)"), 11:w816) -> (0:w815:errorcluster, 3:→"DATA LAB04-1":refnum<k1>)  [unwired: 3 in, 1 out]
                      }
                      frame #2 {
                        w824 = 0.0
                        n553 = local read "DISP LAB04-1"() -> (w826:T4)
                        n554 = Bundle(cluster=w826, "CYCLE"=w824, "MINS"=w824, "STATUS"="RUN") -> (w825:T4)
                        n555 = local write "DISP LAB04-1"(w825) -> ()
                      }
                      frame #3 {
                        n556 = local read "SIG LAB04-1"() -> (w829:T2)
                        n557 = local read "TEMP START LAB04-1"() -> (w831:cluster{"TL":dbl, "TN":dbl})
                        n558 = Unbundle(w829) -> ("Tmp Live"=w828:dbl, "Tmp Neut"=w827:dbl)  [unwired: 3 out]
                        n559 = Bundle(cluster=w831, "TL"=w828, "TN"=w827) -> (w830:cluster{"TL":dbl, "TN":dbl})
                        n560 = local write "TEMP START LAB04-1"(w830) -> ()
                      }
                    }
                  }
                }
              }
              event "RUN LAB04-2": Value Change {
                n561 = event-data() -> ("NewVal"=w832:bool)  [unwired: 1 in, 5 out]
                n562 = local write "run lab04-2"(w832) -> ()
                n563 = case shown="False" w832 {
                  tunnel: w838 -> [_ w854]
                  tunnel: w837 -> [_ w853]
                  tunnel: w835 -> [w840 w852]
                  tunnel: w836 -> [_ w851]
                  tunnel: w834 -> [_ w850]
                  tunnel: [w839 w849] -> w833
                  frame False {
                    # "stop test"
                    n564 = stacked-sequence {
                      tunnel: w840 -> [_ _]
                      tunnel: [_ w844] -> w839
                      frame #0 {
                        n565 = local read "DISP LAB04-2"() -> (w843:T4)
                        n566 = Bundle(cluster=w843, "STATUS"="STOP") -> (w841:T4)  [unwired: 2 in]
                        n567 = local write "DISP LAB04-2"(w841) -> ()
                      }
                      frame #1 {
                        n568 = local read "DATA LAB04-2"() -> (w845:refnum<k1>)
                        n569 = call "Save data file to network drive v1.vi"("panel id"="LAB04-2") -> ("network file save error"=w846:errorcluster)  [unwired: 9 in, 1 out]
                        n570 = local write "RESULT LAB04-2"(FALSE) -> ()
                        n571 = local write "data file error"(w846) -> ()
                        n572 = Close File(refnum=w845) -> (error out=w844:errorcluster)  [unwired: 1 in, 1 out]
                      }
                    }
                  }
                  frame True {
                    # "start new test and create test file"
                    n573 = stacked-sequence {
                      seq-local: [w855 _ _ _] -> [_ w882 _ _]
                      tunnel: w854 -> [w860 _ _ _]
                      tunnel: w853 -> [w856 _ _ _]
                      tunnel: w852 -> [w870 _ _ _]
                      tunnel: w851 -> [w863 _ _ _]
                      tunnel: w850 -> [w858 _ _ _]
                      tunnel: [_ w874 _ _] -> w849
                      frame #0 {
                        w857 = "\\"
                        n574 = local read "SET LAB04-2"() -> (w865:T5)
                        n575 = case shown="\"CHART TEST\", Default" w870 {
                          tunnel: ["CHART TEST-" "CYCLE TEST-" "T-RISE TEST-"] -> w866
                          frame "CHART TEST", Default {
                          }
                          frame "CYCLE TEST" {
                          }
                          frame "T-RISE TEST" {
                          }
                        }
                        n576 = Unbundle(w865) -> ("DESCRIPTION"=w864:string)  [unwired: 4 out]
                        n577 = Concatenate Strings(w860, "LAB04-2\\", w858, w857, w856, w857) -> (w867:string)
                        n578 = String To Path(string=w867) -> (path=w869:path)
                        n579 = Concatenate Strings(w867, w866, w864, "-", w863, ".tdms") -> (w855:string)
                        n580 = Create Folder(path (use dialog)=w869) -> (error out=w868:errorcluster)  [unwired: 2 in, 2 out]
                        n581 = global write "Global 1.vi" "LAB04-2 FILE"(w855) -> ()
                        n582 = call <vilib>:"Clear Errors.vi"("error in (no error)"=w868) -> ()  [unwired: 6 in, 1 out]
                      }
                      frame #1 {
                        n583 = local read "DISP LAB04-2"() -> (w879:T4)
                        n584 = local read "SET LAB04-2"() -> (w881:T5)
                        n585 = local read "SIG LAB04-2"() -> (w880:T2)
                        n586 = String To Path(string=w882) -> (path=w877:path)
                        n587 = Bundle("SET LAB04-2"=w881, "SIG LAB04-2"=w880, "DISP LAB04-2"=w879) -> (w878:T24)  [unwired: 1 in]
                        n588 = Open/Create/Replace Datalog(5:w878, 10:T15."open or create" ("operation (0:open)"), 11:w877) -> (0:w874:errorcluster, 3:→"DATA LAB04-2":refnum<k1>)  [unwired: 3 in, 1 out]
                      }
                      frame #2 {
                        w884 = 0.0
                        n589 = local read "DISP LAB04-2"() -> (w886:T4)
                        n590 = Bundle(cluster=w886, "CYCLE"=w884, "MINS"=w884, "STATUS"="RUN") -> (w885:T4)
                        n591 = local write "DISP LAB04-2"(w885) -> ()
                      }
                      frame #3 {
                        n592 = local read "SIG LAB04-2"() -> (w889:T2)
                        n593 = local read "TEMP START LAB04-2"() -> (w891:cluster{"TL":dbl, "TN":dbl})
                        n594 = Unbundle(w889) -> ("Tmp Live"=w888:dbl, "Tmp Neut"=w887:dbl)  [unwired: 3 out]
                        n595 = Bundle(cluster=w891, "TL"=w888, "TN"=w887) -> (w890:cluster{"TL":dbl, "TN":dbl})
                        n596 = local write "TEMP START LAB04-2"(w890) -> ()
                      }
                    }
                  }
                }
              }
              event "RUN LAB05-1": Value Change {
                n597 = event-data() -> ("NewVal"=w892:bool)  [unwired: 1 in, 5 out]
                n598 = local write "run lab05-1"(w892) -> ()
                n599 = case shown="False" w892 {
                  tunnel: w898 -> [_ w914]
                  tunnel: w897 -> [_ w913]
                  tunnel: w895 -> [w900 w912]
                  tunnel: w896 -> [_ w911]
                  tunnel: w894 -> [_ w910]
                  tunnel: [w899 w909] -> w893
                  frame False {
                    # "stop test"
                    n600 = stacked-sequence {
                      tunnel: w900 -> [_ _]
                      tunnel: [_ w904] -> w899
                      frame #0 {
                        n601 = local read "DISP LAB05-1"() -> (w903:T4)
                        n602 = Bundle(cluster=w903, "STATUS"="STOP") -> (w901:T4)  [unwired: 2 in]
                        n603 = local write "DISP LAB05-1"(w901) -> ()
                      }
                      frame #1 {
                        n604 = local read "DATA LAB05-1"() -> (w905:refnum<k1>)
                        n605 = call "Save data file to network drive v1.vi"("panel id"="LAB05-1") -> ("network file save error"=w906:errorcluster)  [unwired: 9 in, 1 out]
                        n606 = local write "RESULT LAB05-1"(FALSE) -> ()
                        n607 = local write "data file error"(w906) -> ()
                        n608 = Close File(refnum=w905) -> (error out=w904:errorcluster)  [unwired: 1 in, 1 out]
                      }
                    }
                  }
                  frame True {
                    # "start new test and create test file"
                    n609 = stacked-sequence {
                      seq-local: [w915 _ _ _] -> [_ w942 _ _]
                      tunnel: w914 -> [w920 _ _ _]
                      tunnel: w913 -> [w916 _ _ _]
                      tunnel: w912 -> [w930 _ _ _]
                      tunnel: w911 -> [w923 _ _ _]
                      tunnel: w910 -> [w918 _ _ _]
                      tunnel: [_ w935 _ _] -> w909
                      frame #0 {
                        w917 = "\\"
                        n610 = local read "SET LAB05-1"() -> (w925:T5)
                        n611 = case shown="\"CHART TEST\", Default" w930 {
                          tunnel: ["CHART TEST-" "CYCLE TEST-" "T-RISE TEST-"] -> w926
                          frame "CHART TEST", Default {
                          }
                          frame "CYCLE TEST" {
                          }
                          frame "T-RISE TEST" {
                          }
                        }
                        n612 = Unbundle(w925) -> ("DESCRIPTION"=w924:string)  [unwired: 4 out]
                        n613 = Concatenate Strings(w920, "LAB05-1\\", w918, w917, w916, w917) -> (w927:string)
                        n614 = String To Path(string=w927) -> (path=w929:path)
                        n615 = Concatenate Strings(w927, w926, w924, "-", w923, ".dat") -> (w915:string)
                        n616 = Create Folder(path (use dialog)=w929) -> (error out=w928:errorcluster)  [unwired: 2 in, 2 out]
                        n617 = global write "Global 1.vi" "LAB05-1 FILE"(w915) -> ()
                        n618 = call <vilib>:"Clear Errors.vi"("error in (no error)"=w928) -> ()  [unwired: 6 in, 1 out]
                      }
                      frame #1 {
                        n619 = local read "DISP LAB05-1"() -> (w938:T4)
                        n620 = local read "SET LAB05-1"() -> (w940:T5)
                        n621 = local read "SIG LAB05-1"() -> (w939:T2)
                        n622 = String To Path(string=w942) -> (path=w936:path)
                        n623 = Bundle("SET LAB05-1"=w940, "SIG LAB05-1"=w939, "DISP LAB05-1"=w938) -> (w937:T25)  [unwired: 1 in]
                        n624 = Open/Create/Replace Datalog(5:w937, 10:T15."open or create" ("operation (0:open)"), 11:w936) -> (0:w935:errorcluster, 3:→"DATA LAB05-1":refnum<k1>)  [unwired: 3 in, 1 out]
                      }
                      frame #2 {
                        w944 = 0.0
                        n625 = local read "DISP LAB05-1"() -> (w946:T4)
                        n626 = Bundle(cluster=w946, "CYCLE"=w944, "MINS"=w944, "STATUS"="RUN") -> (w945:T4)
                        n627 = local write "DISP LAB05-1"(w945) -> ()
                      }
                      frame #3 {
                        n628 = local read "SIG LAB05-1"() -> (w949:T2)
                        n629 = local read "TEMP START LAB05-1"() -> (w951:cluster{"TL":dbl, "TN":dbl})
                        n630 = Unbundle(w949) -> ("Tmp Live"=w948:dbl, "Tmp Neut"=w947:dbl)  [unwired: 3 out]
                        n631 = Bundle(cluster=w951, "TL"=w948, "TN"=w947) -> (w950:cluster{"TL":dbl, "TN":dbl})
                        n632 = local write "TEMP START LAB05-1"(w950) -> ()
                      }
                    }
                  }
                }
              }
              event "RUN LAB05-2": Value Change {
                n633 = event-data() -> ("NewVal"=w952:bool)  [unwired: 1 in, 5 out]
                n634 = local write "run lab05-2"(w952) -> ()
                n635 = case shown="True" w952 {
                  tunnel: w958 -> [_ w974]
                  tunnel: w957 -> [_ w973]
                  tunnel: w955 -> [w960 w972]
                  tunnel: w956 -> [_ w971]
                  tunnel: w954 -> [_ w970]
                  tunnel: [w959 w969] -> w953
                  frame False {
                    # "stop test"
                    n636 = stacked-sequence {
                      tunnel: w960 -> [_ _]
                      tunnel: [_ w964] -> w959
                      frame #0 {
                        n637 = local read "DISP LAB05-2"() -> (w963:T4)
                        n638 = Bundle(cluster=w963, "STATUS"="STOP") -> (w962:T4)  [unwired: 2 in]
                        n639 = local write "DISP LAB05-2"(w962) -> ()
                      }
                      frame #1 {
                        n640 = local read "DATA LAB05-2"() -> (w965:refnum<k1>)
                        n641 = local write "RESULT LAB05-2"(FALSE) -> ()
                        n642 = call "Save data file to network drive v1.vi"("panel id"="LAB05-2") -> ("network file save error"=w966:errorcluster)  [unwired: 9 in, 1 out]
                        n643 = Close File(refnum=w965) -> (error out=w964:errorcluster)  [unwired: 1 in, 1 out]
                        n644 = local write "data file error"(w966) -> ()
                      }
                    }
                  }
                  frame True {
                    # "start new test and create test file"
                    n645 = stacked-sequence {
                      seq-local: [w975 _ _ _] -> [_ w1002 _ _]
                      tunnel: w974 -> [w980 _ _ _]
                      tunnel: w973 -> [w976 _ _ _]
                      tunnel: w972 -> [w990 _ _ _]
                      tunnel: w971 -> [w983 _ _ _]
                      tunnel: w970 -> [w978 _ _ _]
                      tunnel: [_ w995 _ _] -> w969
                      frame #0 {
                        w977 = "\\"
                        n646 = local read "SET LAB05-2"() -> (w985:T5)
                        n647 = case shown="\"CHART TEST\", Default" w990 {
                          tunnel: ["CHART TEST-" "CYCLE TEST-" "T-RISE TEST-"] -> w986
                          frame "CHART TEST", Default {
                          }
                          frame "CYCLE TEST" {
                          }
                          frame "T-RISE TEST" {
                          }
                        }
                        n648 = Unbundle(w985) -> ("DESCRIPTION"=w984:string)  [unwired: 4 out]
                        n649 = Concatenate Strings(w980, "LAB05-2\\", w978, w977, w976, w977) -> (w987:string)
                        n650 = String To Path(string=w987) -> (path=w989:path)
                        n651 = Concatenate Strings(w987, w986, w984, "-", w983, ".dat") -> (w975:string)
                        n652 = Create Folder(path (use dialog)=w989) -> (error out=w988:errorcluster)  [unwired: 2 in, 2 out]
                        n653 = global write "Global 1.vi" "LAB05-2 FILE"(w975) -> ()
                        n654 = call <vilib>:"Clear Errors.vi"("error in (no error)"=w988) -> ()  [unwired: 6 in, 1 out]
                      }
                      frame #1 {
                        n655 = local read "DISP LAB05-2"() -> (w999:T4)
                        n656 = local read "SET LAB05-2"() -> (w1001:T5)
                        n657 = local read "SIG LAB05-2"() -> (w1000:T2)
                        n658 = String To Path(string=w1002) -> (path=w996:path)
                        n659 = Bundle("SET LAB05-2"=w1001, "SIG LAB05-2"=w1000, "DISP LAB05-2"=w999) -> (w997:T26)  [unwired: 1 in]
                        n660 = Open/Create/Replace Datalog(5:w997, 10:T15."open or create" ("operation (0:open)"), 11:w996) -> (0:w995:errorcluster, 3:→"DATA LAB05-2":refnum<k1>)  [unwired: 3 in, 1 out]
                      }
                      frame #2 {
                        w1004 = 0.0
                        n661 = local read "DISP LAB05-2"() -> (w1006:T4)
                        n662 = Bundle(cluster=w1006, "CYCLE"=w1004, "MINS"=w1004, "STATUS"="RUN") -> (w1005:T4)
                        n663 = local write "DISP LAB05-2"(w1005) -> ()
                      }
                      frame #3 {
                        n664 = local read "SIG LAB05-2"() -> (w1009:T2)
                        n665 = local read "TEMP START LAB05-2"() -> (w1011:cluster{"TL":dbl, "TN":dbl})
                        n666 = Unbundle(w1009) -> ("Tmp Live"=w1008:dbl, "Tmp Neut"=w1007:dbl)  [unwired: 3 out]
                        n667 = Bundle(cluster=w1011, "TL"=w1008, "TN"=w1007) -> (w1010:cluster{"TL":dbl, "TN":dbl})
                        n668 = local write "TEMP START LAB05-2"(w1010) -> ()
                      }
                    }
                  }
                }
              }
            }
            n669 = local write "data file error"(w384) -> ()
          }
          frame #4 {
            # "check if test cycles reached for cycle tests, if so then test pass"
            n670 = stacked-sequence {
              tunnel: w1031 -> [_ _ _ _ _ _ _ _ _ _]
              tunnel: w1030 -> [_ _ _ _ _ _ _ _ _ _]
              tunnel: w1029 -> [_ _ _ _ _ _ _ _ _ _]
              tunnel: w1028 -> [_ _ _ _ _ _ _ _ _ _]
              tunnel: w1027 -> [_ _ _ _ _ _ _ _ _ _]
              tunnel: w1026 -> [_ _ _ _ _ _ _ _ _ _]
              tunnel: w1025 -> [_ _ _ _ _ _ _ _ _ _]
              tunnel: w1024 -> [_ _ _ _ _ _ _ _ _ _]
              tunnel: w1023 -> [_ _ _ _ _ _ _ _ _ _]
              tunnel: w1022 -> [_ _ _ _ _ _ _ _ _ _]
              tunnel: w1021 -> [w1036 _ _ _ _ _ _ _ _ _]
              tunnel: w1020 -> [_ w1066 _ _ _ _ _ _ _ _]
              tunnel: w1019 -> [_ _ w1100 _ _ _ _ _ _ _]
              tunnel: w1018 -> [_ _ _ w1134 _ _ _ _ _ _]
              tunnel: w1017 -> [_ _ _ _ w1168 _ _ _ _ _]
              tunnel: w1016 -> [_ _ _ _ _ w1202 _ _ _ _]
              tunnel: w1015 -> [_ _ _ _ _ _ w1236 _ _ _]
              tunnel: w1014 -> [_ _ _ _ _ _ _ w1270 _ _]
              tunnel: w1013 -> [_ _ _ _ _ _ _ _ w1304 _]
              tunnel: w1012 -> [_ _ _ _ _ _ _ _ _ w1338]
              frame #0 {
                # "LAB01-1"
                n671 = Less?(x=w1036, y=2) -> (x < y?=w1034:bool)
                n672 = local read "DISP LAB01-1"() -> (w1037:T4)
                n673 = Unbundle(w1037) -> ("STATUS"=w1038:string)  [unwired: 2 out]
                n674 = Equal?(x=w1038, y="RUN") -> (x = y?=w1033:bool)
                n675 = And(x=w1033, y=w1034) -> (x .and. y?=w1032:bool)
                n676 = case shown="True" w1032 {
                  tunnel: w1037 -> [_ w1041]
                  tunnel: w1036 -> [_ w1046]
                  frame False {
                  }
                  frame True {
                    n677 = local read "SET LAB01-1"() -> (w1048:T5)
                    n678 = local read "DATA LAB01-1"() -> (w1040:refnum<k1>)
                    n679 = Unbundle(w1041) -> ("CYCLE"=w1047:dbl)  [unwired: 2 out]
                    n680 = Unbundle(w1048) -> ("CYCLES"=w1043:dbl, "T-RISE mins"=w1045:dbl)  [unwired: 3 out]
                    n681 = case shown="\"CHART TEST\", Default" w1046 {
                      tunnel: w1045 -> [_ _ w1055]
                      tunnel: [w1050 w1052 w1055] -> w1044
                      tunnel: w1043 -> [w1050 w1052 _]
                      tunnel: ["CHART TEST" "CYCLES" "T-RISE TEST"] -> w1042
                      frame "CHART TEST", Default {
                      }
                      frame "CYCLE TEST" {
                      }
                      frame "T-RISE TEST" {
                      }
                    }
                    n682 = Greater Or Equal?(x=w1047, y=w1043) -> (x >= y?=w1049:bool)
                    n683 = case shown="True" w1049 {
                      tunnel: w1044 -> [w1059 _]
                      tunnel: w1042 -> [w1058 _]
                      tunnel: w1041 -> [w1057 _]
                      tunnel: w1040 -> [w1056 _]
                      frame True {
                        n684 = stacked-sequence {
                          tunnel: w1059 -> [_ _]
                          tunnel: w1058 -> [_ _]
                          tunnel: w1057 -> [_ w1064]
                          tunnel: w1056 -> [w1061 _]
                          frame #0 {
                            n685 = Close File(refnum=w1061) -> (error out=w1060:errorcluster)  [unwired: 1 in, 1 out]
                            n686 = local write "data file error"(w1060) -> ()
                          }
                          frame #1 {
                            n687 = Bundle(cluster=w1064, "STATUS"="CYCLE PASS") -> (w1062:T4)  [unwired: 2 in]
                            n688 = local write "RESULT LAB01-1"(TRUE) -> ()
                            n689 = local write "DISP LAB01-1"(w1062) -> ()
                          }
                        }
                      }
                      frame False {
                      }
                    }
                  }
                }
              }
              frame #1 {
                # "LAB01-2"
                n690 = Less?(x=w1066, y=2) -> (x < y?=w1069:bool)
                n691 = local read "DISP LAB01-2"() -> (w1071:T4)
                n692 = Unbundle(w1071) -> ("STATUS"=w1072:string)  [unwired: 2 out]
                n693 = Equal?(x=w1072, y="RUN") -> (x = y?=w1068:bool)
                n694 = And(x=w1068, y=w1069) -> (x .and. y?=w1067:bool)
                n695 = case shown="True" w1067 {
                  tunnel: w1071 -> [_ w1075]
                  tunnel: w1066 -> [_ w1080]
                  frame False {
                  }
                  frame True {
                    n696 = local read "SET LAB01-2"() -> (w1082:T5)
                    n697 = local read "DATA LAB01-2"() -> (w1074:refnum<k1>)
                    n698 = Unbundle(w1075) -> ("CYCLE"=w1081:dbl)  [unwired: 2 out]
                    n699 = Unbundle(w1082) -> ("CYCLES"=w1077:dbl, "T-RISE mins"=w1079:dbl)  [unwired: 3 out]
                    n700 = case shown="\"CHART TEST\", Default" w1080 {
                      tunnel: w1079 -> [_ _ w1089]
                      tunnel: [w1084 w1086 w1089] -> w1078
                      tunnel: w1077 -> [w1084 w1086 _]
                      tunnel: ["CHART TEST " "CYCLES" "T-RISE TEST"] -> w1076
                      frame "CHART TEST", Default {
                      }
                      frame "CYCLE TEST" {
                      }
                      frame "T-RISE TEST" {
                      }
                    }
                    n701 = Greater Or Equal?(x=w1081, y=w1077) -> (x >= y?=w1083:bool)
                    n702 = case shown="True" w1083 {
                      tunnel: w1078 -> [w1093 _]
                      tunnel: w1076 -> [w1092 _]
                      tunnel: w1075 -> [w1091 _]
                      tunnel: w1074 -> [w1090 _]
                      frame True {
                        n703 = stacked-sequence {
                          tunnel: w1093 -> [_ _]
                          tunnel: w1092 -> [_ _]
                          tunnel: w1091 -> [_ w1098]
                          tunnel: w1090 -> [w1095 _]
                          frame #0 {
                            n704 = Close File(refnum=w1095) -> (error out=w1094:errorcluster)  [unwired: 1 in, 1 out]
                            n705 = local write "data file error"(w1094) -> ()
                          }
                          frame #1 {
                            n706 = Bundle(cluster=w1098, "STATUS"="CYCLE PASS") -> (w1096:T4)  [unwired: 2 in]
                            n707 = local write "RESULT LAB01-2"(TRUE) -> ()
                            n708 = local write "DISP LAB01-2"(w1096) -> ()
                          }
                        }
                      }
                      frame False {
                      }
                    }
                  }
                }
              }
              frame #2 {
                # "LAB02-1"
                n709 = Less?(x=w1100, y=2) -> (x < y?=w1103:bool)
                n710 = local read "DISP LAB02-1"() -> (w1105:T4)
                n711 = Unbundle(w1105) -> ("STATUS"=w1106:string)  [unwired: 2 out]
                n712 = Equal?(x=w1106, y="RUN") -> (x = y?=w1102:bool)
                n713 = And(x=w1102, y=w1103) -> (x .and. y?=w1101:bool)
                n714 = case shown="True" w1101 {
                  tunnel: w1105 -> [_ w1109]
                  tunnel: w1100 -> [_ w1114]
                  frame False {
                  }
                  frame True {
                    n715 = local read "SET LAB02-1"() -> (w1116:T5)
                    n716 = local read "DATA LAB02-1"() -> (w1108:refnum<k1>)
                    n717 = Unbundle(w1109) -> ("CYCLE"=w1115:dbl)  [unwired: 2 out]
                    n718 = Unbundle(w1116) -> ("CYCLES"=w1111:dbl, "T-RISE mins"=w1113:dbl)  [unwired: 3 out]
                    n719 = case shown="\"CHART TEST\", Default" w1114 {
                      tunnel: w1113 -> [_ _ w1123]
                      tunnel: [w1118 w1120 w1123] -> w1112
                      tunnel: w1111 -> [w1118 w1120 _]
                      tunnel: ["CHART TEST" "CYCLES" "T-RISE TEST"] -> w1110
                      frame "CHART TEST", Default {
                      }
                      frame "CYCLE TEST" {
                      }
                      frame "T-RISE TEST" {
                      }
                    }
                    n720 = Greater Or Equal?(x=w1115, y=w1111) -> (x >= y?=w1117:bool)
                    n721 = case shown="True" w1117 {
                      tunnel: w1112 -> [w1127 _]
                      tunnel: w1110 -> [w1126 _]
                      tunnel: w1109 -> [w1125 _]
                      tunnel: w1108 -> [w1124 _]
                      frame True {
                        n722 = stacked-sequence {
                          tunnel: w1127 -> [_ _]
                          tunnel: w1126 -> [_ _]
                          tunnel: w1125 -> [_ w1132]
                          tunnel: w1124 -> [w1129 _]
                          frame #0 {
                            n723 = Close File(refnum=w1129) -> (error out=w1128:errorcluster)  [unwired: 1 in, 1 out]
                            n724 = local write "data file error"(w1128) -> ()
                          }
                          frame #1 {
                            n725 = Bundle(cluster=w1132, "STATUS"="CYCLE PASS") -> (w1130:T4)  [unwired: 2 in]
                            n726 = local write "RESULT LAB02-1"(TRUE) -> ()
                            n727 = local write "DISP LAB02-1"(w1130) -> ()
                          }
                        }
                      }
                      frame False {
                      }
                    }
                  }
                }
              }
              frame #3 {
                # "LAB02-2"
                n728 = Less?(x=w1134, y=2) -> (x < y?=w1137:bool)
                n729 = local read "DISP LAB02-2"() -> (w1139:T4)
                n730 = Unbundle(w1139) -> ("STATUS"=w1140:string)  [unwired: 2 out]
                n731 = Equal?(x=w1140, y="RUN") -> (x = y?=w1136:bool)
                n732 = And(x=w1136, y=w1137) -> (x .and. y?=w1135:bool)
                n733 = case shown="True" w1135 {
                  tunnel: w1139 -> [_ w1143]
                  tunnel: w1134 -> [_ w1148]
                  frame False {
                  }
                  frame True {
                    n734 = local read "SET LAB02-2"() -> (w1150:T5)
                    n735 = local read "DATA LAB02-2"() -> (w1142:refnum<k1>)
                    n736 = Unbundle(w1143) -> ("CYCLE"=w1149:dbl)  [unwired: 2 out]
                    n737 = Unbundle(w1150) -> ("CYCLES"=w1145:dbl, "T-RISE mins"=w1147:dbl)  [unwired: 3 out]
                    n738 = case shown="\"CHART TEST\", Default" w1148 {
                      tunnel: w1147 -> [_ _ w1157]
                      tunnel: [w1152 w1154 w1157] -> w1146
                      tunnel: w1145 -> [w1152 w1154 _]
                      tunnel: ["CHART TEST" "CYCLES" "T-RISE TEST"] -> w1144
                      frame "CHART TEST", Default {
                      }
                      frame "CYCLE TEST" {
                      }
                      frame "T-RISE TEST" {
                      }
                    }
                    n739 = Greater Or Equal?(x=w1149, y=w1145) -> (x >= y?=w1151:bool)
                    n740 = case shown="True" w1151 {
                      tunnel: w1146 -> [w1161 _]
                      tunnel: w1144 -> [w1160 _]
                      tunnel: w1143 -> [w1159 _]
                      tunnel: w1142 -> [w1158 _]
                      frame True {
                        n741 = stacked-sequence {
                          tunnel: w1161 -> [_ _]
                          tunnel: w1160 -> [_ _]
                          tunnel: w1159 -> [_ w1166]
                          tunnel: w1158 -> [w1163 _]
                          frame #0 {
                            n742 = Close File(refnum=w1163) -> (error out=w1162:errorcluster)  [unwired: 1 in, 1 out]
                            n743 = local write "data file error"(w1162) -> ()
                          }
                          frame #1 {
                            n744 = Bundle(cluster=w1166, "STATUS"="CYCLE PASS") -> (w1164:T4)  [unwired: 2 in]
                            n745 = local write "RESULT LAB02-2"(TRUE) -> ()
                            n746 = local write "DISP LAB02-2"(w1164) -> ()
                          }
                        }
                      }
                      frame False {
                      }
                    }
                  }
                }
              }
              frame #4 {
                # "LAB03-1"
                n747 = Less?(x=w1168, y=2) -> (x < y?=w1171:bool)
                n748 = local read "DISP LAB03-1"() -> (w1173:T4)
                n749 = Unbundle(w1173) -> ("STATUS"=w1174:string)  [unwired: 2 out]
                n750 = Equal?(x=w1174, y="RUN") -> (x = y?=w1170:bool)
                n751 = And(x=w1170, y=w1171) -> (x .and. y?=w1169:bool)
                n752 = case shown="True" w1169 {
                  tunnel: w1173 -> [_ w1177]
                  tunnel: w1168 -> [_ w1182]
                  frame False {
                  }
                  frame True {
                    n753 = local read "SET LAB03-1"() -> (w1184:T5)
                    n754 = local read "DATA LAB03-1"() -> (w1176:refnum<k1>)
                    n755 = Unbundle(w1177) -> ("CYCLE"=w1183:dbl)  [unwired: 2 out]
                    n756 = Unbundle(w1184) -> ("CYCLES"=w1179:dbl, "T-RISE mins"=w1181:dbl)  [unwired: 3 out]
                    n757 = case shown="\"CHART TEST\", Default" w1182 {
                      tunnel: w1181 -> [_ _ w1191]
                      tunnel: [w1186 w1188 w1191] -> w1180
                      tunnel: w1179 -> [w1186 w1188 _]
                      tunnel: ["CHART TEST" "CYCLES" "T-RISE TEST"] -> w1178
                      frame "CHART TEST", Default {
                      }
                      frame "CYCLE TEST" {
                      }
                      frame "T-RISE TEST" {
                      }
                    }
                    n758 = Greater Or Equal?(x=w1183, y=w1179) -> (x >= y?=w1185:bool)
                    n759 = case shown="True" w1185 {
                      tunnel: w1180 -> [w1195 _]
                      tunnel: w1178 -> [w1194 _]
                      tunnel: w1177 -> [w1193 _]
                      tunnel: w1176 -> [w1192 _]
                      frame True {
                        n760 = stacked-sequence {
                          tunnel: w1195 -> [_ _]
                          tunnel: w1194 -> [_ _]
                          tunnel: w1193 -> [_ w1200]
                          tunnel: w1192 -> [w1197 _]
                          frame #0 {
                            n761 = Close File(refnum=w1197) -> (error out=w1196:errorcluster)  [unwired: 1 in, 1 out]
                            n762 = local write "data file error"(w1196) -> ()
                          }
                          frame #1 {
                            n763 = Bundle(cluster=w1200, "STATUS"="CYCLE PASS") -> (w1198:T4)  [unwired: 2 in]
                            n764 = local write "RESULT LAB03-1"(TRUE) -> ()
                            n765 = local write "DISP LAB03-1"(w1198) -> ()
                          }
                        }
                      }
                      frame False {
                      }
                    }
                  }
                }
              }
              frame #5 {
                # "LAB03-2"
                n766 = Less?(x=w1202, y=2) -> (x < y?=w1205:bool)
                n767 = local read "DISP LAB03-2"() -> (w1207:T4)
                n768 = Unbundle(w1207) -> ("STATUS"=w1208:string)  [unwired: 2 out]
                n769 = Equal?(x=w1208, y="RUN") -> (x = y?=w1204:bool)
                n770 = And(x=w1204, y=w1205) -> (x .and. y?=w1203:bool)
                n771 = case shown="True" w1203 {
                  tunnel: w1207 -> [_ w1211]
                  tunnel: w1202 -> [_ w1216]
                  frame False {
                  }
                  frame True {
                    n772 = local read "SET LAB03-2"() -> (w1218:T5)
                    n773 = local read "DATA LAB03-2"() -> (w1210:refnum<k1>)
                    n774 = Unbundle(w1211) -> ("CYCLE"=w1217:dbl)  [unwired: 2 out]
                    n775 = Unbundle(w1218) -> ("CYCLES"=w1213:dbl, "T-RISE mins"=w1215:dbl)  [unwired: 3 out]
                    n776 = case shown="\"CHART TEST\", Default" w1216 {
                      tunnel: w1215 -> [_ _ w1225]
                      tunnel: [w1220 w1222 w1225] -> w1214
                      tunnel: w1213 -> [w1220 w1222 _]
                      tunnel: ["CHART TEST" "CYCLES" "T-RISE TEST"] -> w1212
                      frame "CHART TEST", Default {
                      }
                      frame "CYCLE TEST" {
                      }
                      frame "T-RISE TEST" {
                      }
                    }
                    n777 = Greater Or Equal?(x=w1217, y=w1213) -> (x >= y?=w1219:bool)
                    n778 = case shown="True" w1219 {
                      tunnel: w1214 -> [w1229 _]
                      tunnel: w1212 -> [w1228 _]
                      tunnel: w1211 -> [w1227 _]
                      tunnel: w1210 -> [w1226 _]
                      frame True {
                        n779 = stacked-sequence {
                          tunnel: w1229 -> [_ _]
                          tunnel: w1228 -> [_ _]
                          tunnel: w1227 -> [_ w1234]
                          tunnel: w1226 -> [w1231 _]
                          frame #0 {
                            n780 = Close File(refnum=w1231) -> (error out=w1230:errorcluster)  [unwired: 1 in, 1 out]
                            n781 = local write "data file error"(w1230) -> ()
                          }
                          frame #1 {
                            n782 = Bundle(cluster=w1234, "STATUS"="CYCLE PASS") -> (w1232:T4)  [unwired: 2 in]
                            n783 = local write "RESULT LAB03-2"(TRUE) -> ()
                            n784 = local write "DISP LAB03-2"(w1232) -> ()
                          }
                        }
                      }
                      frame False {
                      }
                    }
                  }
                }
              }
              frame #6 {
                # "LAB04-1"
                n785 = Less?(x=w1236, y=2) -> (x < y?=w1239:bool)
                n786 = local read "DISP LAB04-1"() -> (w1241:T4)
                n787 = Unbundle(w1241) -> ("STATUS"=w1242:string)  [unwired: 2 out]
                n788 = Equal?(x=w1242, y="RUN") -> (x = y?=w1238:bool)
                n789 = And(x=w1238, y=w1239) -> (x .and. y?=w1237:bool)
                n790 = case shown="True" w1237 {
                  tunnel: w1241 -> [_ w1245]
                  tunnel: w1236 -> [_ w1250]
                  frame False {
                  }
                  frame True {
                    n791 = local read "SET LAB04-1"() -> (w1252:T5)
                    n792 = local read "DATA LAB04-1"() -> (w1244:refnum<k1>)
                    n793 = Unbundle(w1245) -> ("CYCLE"=w1251:dbl)  [unwired: 2 out]
                    n794 = Unbundle(w1252) -> ("CYCLES"=w1247:dbl, "T-RISE mins"=w1249:dbl)  [unwired: 3 out]
                    n795 = case shown="\"CHART TEST\", Default" w1250 {
                      tunnel: w1249 -> [_ _ w1259]
                      tunnel: [w1254 w1256 w1259] -> w1248
                      tunnel: w1247 -> [w1254 w1256 _]
                      tunnel: ["CHART TEST" "CYCLES" "T-RISE TEST"] -> w1246
                      frame "CHART TEST", Default {
                      }
                      frame "CYCLE TEST" {
                      }
                      frame "T-RISE TEST" {
                      }
                    }
                    n796 = Greater Or Equal?(x=w1251, y=w1247) -> (x >= y?=w1253:bool)
                    n797 = case shown="True" w1253 {
                      tunnel: w1248 -> [w1263 _]
                      tunnel: w1246 -> [w1262 _]
                      tunnel: w1245 -> [w1261 _]
                      tunnel: w1244 -> [w1260 _]
                      frame True {
                        n798 = stacked-sequence {
                          tunnel: w1263 -> [_ _]
                          tunnel: w1262 -> [_ _]
                          tunnel: w1261 -> [_ w1268]
                          tunnel: w1260 -> [w1265 _]
                          frame #0 {
                            n799 = Close File(refnum=w1265) -> (error out=w1264:errorcluster)  [unwired: 1 in, 1 out]
                            n800 = local write "data file error"(w1264) -> ()
                          }
                          frame #1 {
                            n801 = Bundle(cluster=w1268, "STATUS"="CYCLE PASS") -> (w1266:T4)  [unwired: 2 in]
                            n802 = local write "RESULT LAB04-1"(TRUE) -> ()
                            n803 = local write "DISP LAB04-1"(w1266) -> ()
                          }
                        }
                      }
                      frame False {
                      }
                    }
                  }
                }
              }
              frame #7 {
                # "LAB04-2"
                n804 = Less?(x=w1270, y=2) -> (x < y?=w1273:bool)
                n805 = local read "DISP LAB04-2"() -> (w1275:T4)
                n806 = Unbundle(w1275) -> ("STATUS"=w1276:string)  [unwired: 2 out]
                n807 = Equal?(x=w1276, y="RUN") -> (x = y?=w1272:bool)
                n808 = And(x=w1272, y=w1273) -> (x .and. y?=w1271:bool)
                n809 = case shown="True" w1271 {
                  tunnel: w1275 -> [_ w1279]
                  tunnel: w1270 -> [_ w1284]
                  frame False {
                  }
                  frame True {
                    n810 = local read "SET LAB04-2"() -> (w1286:T5)
                    n811 = local read "DATA LAB04-2"() -> (w1278:refnum<k1>)
                    n812 = Unbundle(w1279) -> ("CYCLE"=w1285:dbl)  [unwired: 2 out]
                    n813 = Unbundle(w1286) -> ("CYCLES"=w1281:dbl, "T-RISE mins"=w1283:dbl)  [unwired: 3 out]
                    n814 = case shown="\"CHART TEST\", Default" w1284 {
                      tunnel: w1283 -> [_ _ w1293]
                      tunnel: [w1288 w1290 w1293] -> w1282
                      tunnel: w1281 -> [w1288 w1290 _]
                      tunnel: ["CHART TEST" "CYCLES" "T-RISE TEST"] -> w1280
                      frame "CHART TEST", Default {
                      }
                      frame "CYCLE TEST" {
                      }
                      frame "T-RISE TEST" {
                      }
                    }
                    n815 = Greater Or Equal?(x=w1285, y=w1281) -> (x >= y?=w1287:bool)
                    n816 = case shown="True" w1287 {
                      tunnel: w1282 -> [w1297 _]
                      tunnel: w1280 -> [w1296 _]
                      tunnel: w1279 -> [w1295 _]
                      tunnel: w1278 -> [w1294 _]
                      frame True {
                        n817 = stacked-sequence {
                          tunnel: w1297 -> [_ _]
                          tunnel: w1296 -> [_ _]
                          tunnel: w1295 -> [_ w1302]
                          tunnel: w1294 -> [w1299 _]
                          frame #0 {
                            n818 = Close File(refnum=w1299) -> (error out=w1298:errorcluster)  [unwired: 1 in, 1 out]
                            n819 = local write "data file error"(w1298) -> ()
                          }
                          frame #1 {
                            n820 = Bundle(cluster=w1302, "STATUS"="CYCLE PASS") -> (w1300:T4)  [unwired: 2 in]
                            n821 = local write "RESULT LAB04-2"(TRUE) -> ()
                            n822 = local write "DISP LAB04-2"(w1300) -> ()
                          }
                        }
                      }
                      frame False {
                      }
                    }
                  }
                }
              }
              frame #8 {
                # "LAB05-1"
                n823 = Less?(x=w1304, y=2) -> (x < y?=w1307:bool)
                n824 = local read "DISP LAB05-1"() -> (w1309:T4)
                n825 = Unbundle(w1309) -> ("STATUS"=w1310:string)  [unwired: 2 out]
                n826 = Equal?(x=w1310, y="RUN") -> (x = y?=w1306:bool)
                n827 = And(x=w1306, y=w1307) -> (x .and. y?=w1305:bool)
                n828 = case shown="True" w1305 {
                  tunnel: w1309 -> [_ w1313]
                  tunnel: w1304 -> [_ w1318]
                  frame False {
                  }
                  frame True {
                    n829 = local read "SET LAB05-1"() -> (w1320:T5)
                    n830 = local read "DATA LAB05-1"() -> (w1312:refnum<k1>)
                    n831 = Unbundle(w1313) -> ("CYCLE"=w1319:dbl)  [unwired: 2 out]
                    n832 = Unbundle(w1320) -> ("CYCLES"=w1315:dbl, "T-RISE mins"=w1317:dbl)  [unwired: 3 out]
                    n833 = case shown="\"CHART TEST\", Default" w1318 {
                      tunnel: w1317 -> [_ _ w1327]
                      tunnel: [w1322 w1324 w1327] -> w1316
                      tunnel: w1315 -> [w1322 w1324 _]
                      tunnel: ["CHART TEST" "CYCLES" "T-RISE TEST"] -> w1314
                      frame "CHART TEST", Default {
                      }
                      frame "CYCLE TEST" {
                      }
                      frame "T-RISE TEST" {
                      }
                    }
                    n834 = Greater Or Equal?(x=w1319, y=w1315) -> (x >= y?=w1321:bool)
                    n835 = case shown="True" w1321 {
                      tunnel: w1316 -> [w1331 _]
                      tunnel: w1314 -> [w1330 _]
                      tunnel: w1313 -> [w1329 _]
                      tunnel: w1312 -> [w1328 _]
                      frame True {
                        n836 = stacked-sequence {
                          tunnel: w1331 -> [_ _]
                          tunnel: w1330 -> [_ _]
                          tunnel: w1329 -> [_ w1336]
                          tunnel: w1328 -> [w1333 _]
                          frame #0 {
                            n837 = Close File(refnum=w1333) -> (error out=w1332:errorcluster)  [unwired: 1 in, 1 out]
                            n838 = local write "data file error"(w1332) -> ()
                          }
                          frame #1 {
                            n839 = Bundle(cluster=w1336, "STATUS"="CYCLE PASS") -> (w1334:T4)  [unwired: 2 in]
                            n840 = local write "RESULT LAB05-1"(TRUE) -> ()
                            n841 = local write "DISP LAB05-1"(w1334) -> ()
                          }
                        }
                      }
                      frame False {
                      }
                    }
                  }
                }
              }
              frame #9 {
                # "LAB05-2"
                n842 = Less?(x=w1338, y=2) -> (x < y?=w1341:bool)
                n843 = local read "DISP LAB05-2"() -> (w1343:T4)
                n844 = Unbundle(w1343) -> ("STATUS"=w1344:string)  [unwired: 2 out]
                n845 = Equal?(x=w1344, y="RUN") -> (x = y?=w1340:bool)
                n846 = And(x=w1340, y=w1341) -> (x .and. y?=w1339:bool)
                n847 = case shown="True" w1339 {
                  tunnel: w1343 -> [_ w1347]
                  tunnel: w1338 -> [_ w1352]
                  frame False {
                  }
                  frame True {
                    n848 = local read "SET LAB05-2"() -> (w1354:T5)
                    n849 = local read "DATA LAB05-2"() -> (w1346:refnum<k1>)
                    n850 = Unbundle(w1347) -> ("CYCLE"=w1353:dbl)  [unwired: 2 out]
                    n851 = Unbundle(w1354) -> ("CYCLES"=w1349:dbl, "T-RISE mins"=w1351:dbl)  [unwired: 3 out]
                    n852 = case shown="\"CHART TEST\", Default" w1352 {
                      tunnel: w1351 -> [_ _ w1361]
                      tunnel: [w1356 w1358 w1361] -> w1350
                      tunnel: w1349 -> [w1356 w1358 _]
                      tunnel: ["CHART TEST" "CYCLES" "T-RISE TEST"] -> w1348
                      frame "CHART TEST", Default {
                      }
                      frame "CYCLE TEST" {
                      }
                      frame "T-RISE TEST" {
                      }
                    }
                    n853 = Greater Or Equal?(x=w1353, y=w1349) -> (x >= y?=w1355:bool)
                    n854 = case shown="True" w1355 {
                      tunnel: w1350 -> [w1365 _]
                      tunnel: w1348 -> [w1364 _]
                      tunnel: w1347 -> [w1363 _]
                      tunnel: w1346 -> [w1362 _]
                      frame True {
                        n855 = stacked-sequence {
                          tunnel: w1365 -> [_ _]
                          tunnel: w1364 -> [_ _]
                          tunnel: w1363 -> [_ w1370]
                          tunnel: w1362 -> [w1367 _]
                          frame #0 {
                            n856 = Close File(refnum=w1367) -> (error out=w1366:errorcluster)  [unwired: 1 in, 1 out]
                            n857 = local write "data file error"(w1366) -> ()
                          }
                          frame #1 {
                            n858 = Bundle(cluster=w1370, "STATUS"="CYCLE PASS") -> (w1368:T4)  [unwired: 2 in]
                            n859 = local write "RESULT LAB05-2"(TRUE) -> ()
                            n860 = local write "DISP LAB05-2"(w1368) -> ()
                          }
                        }
                      }
                      frame False {
                      }
                    }
                  }
                }
              }
            }
          }
          frame #5 {
            # "check if test cycles reached for temperature rise test"
            n861 = stacked-sequence {
              tunnel: w1401 -> [_ _ _ _ _ _ _ _ _ _]
              tunnel: w1400 -> [_ _ _ _ _ _ _ _ _ _]
              tunnel: w1399 -> [_ _ _ _ _ _ _ _ _ _]
              tunnel: w1398 -> [_ _ _ _ _ _ _ _ _ _]
              tunnel: w1397 -> [_ _ _ _ _ _ _ _ _ _]
              tunnel: w1396 -> [_ _ _ _ _ _ _ _ _ _]
              tunnel: w1395 -> [_ _ _ _ _ _ _ _ _ _]
              tunnel: w1394 -> [_ _ _ _ _ _ _ _ _ _]
              tunnel: w1393 -> [_ _ _ _ _ _ _ _ _ _]
              tunnel: w1392 -> [_ _ _ _ _ _ _ _ _ _]
              tunnel: w1391 -> [w1407 _ _ _ _ _ _ _ _ _]
              tunnel: w1381 -> [w1402 _ _ _ _ _ _ _ _ _]
              tunnel: w1390 -> [_ w1428 _ _ _ _ _ _ _ _]
              tunnel: w1389 -> [_ _ w1453 _ _ _ _ _ _ _]
              tunnel: w1388 -> [_ _ _ w1478 _ _ _ _ _ _]
              tunnel: w1387 -> [_ _ _ _ w1503 _ _ _ _ _]
              tunnel: w1386 -> [_ _ _ _ _ w1528 _ _ _ _]
              tunnel: w1385 -> [_ _ _ _ _ _ w1553 _ _ _]
              tunnel: w1384 -> [_ _ _ _ _ _ _ w1578 _ _]
              tunnel: w1383 -> [_ _ _ _ _ _ _ _ w1603 _]
              tunnel: w1382 -> [_ _ _ _ _ _ _ _ _ w1628]
              tunnel: w1380 -> [_ w1427 _ _ _ _ _ _ _ _]
              tunnel: w1379 -> [_ _ w1452 _ _ _ _ _ _ _]
              tunnel: w1378 -> [_ _ _ w1477 _ _ _ _ _ _]
              tunnel: w1377 -> [_ _ _ _ w1502 _ _ _ _ _]
              tunnel: w1376 -> [_ _ _ _ _ w1527 _ _ _ _]
              tunnel: w1375 -> [_ _ _ _ _ _ w1552 _ _ _]
              tunnel: w1374 -> [_ _ _ _ _ _ _ w1577 _ _]
              tunnel: w1373 -> [_ _ _ _ _ _ _ _ w1602 _]
              tunnel: w1372 -> [_ _ _ _ _ _ _ _ _ w1627]
              frame #0 {
                # "LAB01-1"
                n862 = Equal?(x=w1407, y=2) -> (x = y?=w1405:bool)
                n863 = local read "DISP LAB01-1"() -> (w1408:T4)
                n864 = Unbundle(w1408) -> ("STATUS"=w1409:string)  [unwired: 2 out]
                n865 = Equal?(x=w1409, y="RUN") -> (x = y?=w1404:bool)
                n866 = And(x=w1404, y=w1405) -> (x .and. y?=w1403:bool)
                n867 = case shown="True" w1403 {
                  tunnel: w1408 -> [_ w1412]
                  tunnel: w1402 -> [_ w1415]
                  frame False {
                  }
                  frame True {
                    n868 = local read "SET LAB01-1"() -> (w1414:T5)
                    n869 = local read "DATA LAB01-1"() -> (w1411:refnum<k1>)
                    n870 = Unbundle(w1412) -> ("CYCLE"=w1416:dbl)  [unwired: 2 out]
                    n871 = Unbundle(w1414) -> ("T-RISE mins"=w1413:dbl)  [unwired: 4 out]
                    n872 = Greater Or Equal?(x=w1416, y=w1415) -> (x >= y?=w1417:bool)
                    n873 = case shown="True" w1417 {
                      tunnel: w1413 -> [w1420 _]
                      tunnel: w1412 -> [w1419 _]
                      tunnel: w1411 -> [w1418 _]
                      frame True {
                        n874 = stacked-sequence {
                          tunnel: w1420 -> [_ _]
                          tunnel: w1419 -> [_ w1423]
                          tunnel: w1418 -> [w1422 _]
                          frame #0 {
                            n875 = Close File(refnum=w1422) -> (error out=w1421:errorcluster)  [unwired: 1 in, 1 out]
                            n876 = local write "data file error"(w1421) -> ()
                          }
                          frame #1 {
                            n877 = Bundle(cluster=w1423, "STATUS"="T-RISE PASS") -> (w1425:T4)  [unwired: 2 in]
                            n878 = local write "RESULT LAB01-1"(TRUE) -> ()
                            n879 = local write "DISP LAB01-1"(w1425) -> ()
                          }
                        }
                      }
                      frame False {
                      }
                    }
                  }
                }
              }
              frame #1 {
                # "LAB01-2"
                n880 = Equal?(x=w1428, y=2) -> (x = y?=w1431:bool)
                n881 = local read "DISP LAB01-2"() -> (w1433:T4)
                n882 = Unbundle(w1433) -> ("STATUS"=w1434:string)  [unwired: 2 out]
                n883 = Equal?(x=w1434, y="RUN") -> (x = y?=w1430:bool)
                n884 = And(x=w1430, y=w1431) -> (x .and. y?=w1429:bool)
                n885 = case shown="True" w1429 {
                  tunnel: w1433 -> [_ w1437]
                  tunnel: w1427 -> [_ w1440]
                  frame False {
                  }
                  frame True {
                    n886 = local read "SET LAB01-2"() -> (w1439:T5)
                    n887 = local read "DATA LAB01-2"() -> (w1436:refnum<k1>)
                    n888 = Unbundle(w1437) -> ("CYCLE"=w1441:dbl)  [unwired: 2 out]
                    n889 = Unbundle(w1439) -> ("T-RISE mins"=w1438:dbl)  [unwired: 4 out]
                    n890 = Greater Or Equal?(x=w1441, y=w1440) -> (x >= y?=w1442:bool)
                    n891 = case shown="True" w1442 {
                      tunnel: w1438 -> [w1445 _]
                      tunnel: w1437 -> [w1444 _]
                      tunnel: w1436 -> [w1443 _]
                      frame True {
                        n892 = stacked-sequence {
                          tunnel: w1445 -> [_ _]
                          tunnel: w1444 -> [_ w1448]
                          tunnel: w1443 -> [w1447 _]
                          frame #0 {
                            n893 = Close File(refnum=w1447) -> (error out=w1446:errorcluster)  [unwired: 1 in, 1 out]
                            n894 = local write "data file error"(w1446) -> ()
                          }
                          frame #1 {
                            n895 = Bundle(cluster=w1448, "STATUS"="T-RISE PASS") -> (w1450:T4)  [unwired: 2 in]
                            n896 = local write "RESULT LAB01-2"(TRUE) -> ()
                            n897 = local write "DISP LAB01-2"(w1450) -> ()
                          }
                        }
                      }
                      frame False {
                      }
                    }
                  }
                }
              }
              frame #2 {
                # "LAB02-1"
                n898 = Equal?(x=w1453, y=2) -> (x = y?=w1456:bool)
                n899 = local read "DISP LAB02-1"() -> (w1458:T4)
                n900 = Unbundle(w1458) -> ("STATUS"=w1459:string)  [unwired: 2 out]
                n901 = Equal?(x=w1459, y="RUN") -> (x = y?=w1455:bool)
                n902 = And(x=w1455, y=w1456) -> (x .and. y?=w1454:bool)
                n903 = case shown="True" w1454 {
                  tunnel: w1458 -> [_ w1462]
                  tunnel: w1452 -> [_ w1465]
                  frame False {
                  }
                  frame True {
                    n904 = local read "SET LAB02-1"() -> (w1464:T5)
                    n905 = local read "DATA LAB02-1"() -> (w1461:refnum<k1>)
                    n906 = Unbundle(w1462) -> ("CYCLE"=w1466:dbl)  [unwired: 2 out]
                    n907 = Unbundle(w1464) -> ("T-RISE mins"=w1463:dbl)  [unwired: 4 out]
                    n908 = Greater Or Equal?(x=w1466, y=w1465) -> (x >= y?=w1467:bool)
                    n909 = case shown="True" w1467 {
                      tunnel: w1463 -> [w1470 _]
                      tunnel: w1462 -> [w1469 _]
                      tunnel: w1461 -> [w1468 _]
                      frame True {
                        n910 = stacked-sequence {
                          tunnel: w1470 -> [_ _]
                          tunnel: w1469 -> [_ w1473]
                          tunnel: w1468 -> [w1472 _]
                          frame #0 {
                            n911 = Close File(refnum=w1472) -> (error out=w1471:errorcluster)  [unwired: 1 in, 1 out]
                            n912 = local write "data file error"(w1471) -> ()
                          }
                          frame #1 {
                            n913 = Bundle(cluster=w1473, "STATUS"="T-RISE PASS") -> (w1475:T4)  [unwired: 2 in]
                            n914 = local write "RESULT LAB02-1"(TRUE) -> ()
                            n915 = local write "DISP LAB02-1"(w1475) -> ()
                          }
                        }
                      }
                      frame False {
                      }
                    }
                  }
                }
              }
              frame #3 {
                # "LAB02-2"
                n916 = Equal?(x=w1478, y=2) -> (x = y?=w1481:bool)
                n917 = local read "DISP LAB02-2"() -> (w1483:T4)
                n918 = Unbundle(w1483) -> ("STATUS"=w1484:string)  [unwired: 2 out]
                n919 = Equal?(x=w1484, y="RUN") -> (x = y?=w1480:bool)
                n920 = And(x=w1480, y=w1481) -> (x .and. y?=w1479:bool)
                n921 = case shown="True" w1479 {
                  tunnel: w1483 -> [_ w1487]
                  tunnel: w1477 -> [_ w1490]
                  frame False {
                  }
                  frame True {
                    n922 = local read "SET LAB02-2"() -> (w1489:T5)
                    n923 = local read "DATA LAB02-2"() -> (w1486:refnum<k1>)
                    n924 = Unbundle(w1487) -> ("CYCLE"=w1491:dbl)  [unwired: 2 out]
                    n925 = Unbundle(w1489) -> ("T-RISE mins"=w1488:dbl)  [unwired: 4 out]
                    n926 = Greater Or Equal?(x=w1491, y=w1490) -> (x >= y?=w1492:bool)
                    n927 = case shown="True" w1492 {
                      tunnel: w1488 -> [w1495 _]
                      tunnel: w1487 -> [w1494 _]
                      tunnel: w1486 -> [w1493 _]
                      frame True {
                        n928 = stacked-sequence {
                          tunnel: w1495 -> [_ _]
                          tunnel: w1494 -> [_ w1498]
                          tunnel: w1493 -> [w1497 _]
                          frame #0 {
                            n929 = Close File(refnum=w1497) -> (error out=w1496:errorcluster)  [unwired: 1 in, 1 out]
                            n930 = local write "data file error"(w1496) -> ()
                          }
                          frame #1 {
                            n931 = Bundle(cluster=w1498, "STATUS"="T-RISE PASS") -> (w1500:T4)  [unwired: 2 in]
                            n932 = local write "RESULT LAB02-2"(TRUE) -> ()
                            n933 = local write "DISP LAB02-2"(w1500) -> ()
                          }
                        }
                      }
                      frame False {
                      }
                    }
                  }
                }
              }
              frame #4 {
                # "LAB03-1"
                n934 = Equal?(x=w1503, y=2) -> (x = y?=w1506:bool)
                n935 = local read "DISP LAB03-1"() -> (w1508:T4)
                n936 = Unbundle(w1508) -> ("STATUS"=w1509:string)  [unwired: 2 out]
                n937 = Equal?(x=w1509, y="RUN") -> (x = y?=w1505:bool)
                n938 = And(x=w1505, y=w1506) -> (x .and. y?=w1504:bool)
                n939 = case shown="True" w1504 {
                  tunnel: w1508 -> [_ w1512]
                  tunnel: w1502 -> [_ w1515]
                  frame False {
                  }
                  frame True {
                    n940 = local read "SET LAB03-1"() -> (w1514:T5)
                    n941 = local read "DATA LAB03-1"() -> (w1511:refnum<k1>)
                    n942 = Unbundle(w1512) -> ("CYCLE"=w1516:dbl)  [unwired: 2 out]
                    n943 = Unbundle(w1514) -> ("T-RISE mins"=w1513:dbl)  [unwired: 4 out]
                    n944 = Greater Or Equal?(x=w1516, y=w1515) -> (x >= y?=w1517:bool)
                    n945 = case shown="True" w1517 {
                      tunnel: w1513 -> [w1520 _]
                      tunnel: w1512 -> [w1519 _]
                      tunnel: w1511 -> [w1518 _]
                      frame True {
                        n946 = stacked-sequence {
                          tunnel: w1520 -> [_ _]
                          tunnel: w1519 -> [_ w1523]
                          tunnel: w1518 -> [w1522 _]
                          frame #0 {
                            n947 = Close File(refnum=w1522) -> (error out=w1521:errorcluster)  [unwired: 1 in, 1 out]
                            n948 = local write "data file error"(w1521) -> ()
                          }
                          frame #1 {
                            n949 = Bundle(cluster=w1523, "STATUS"="T-RISE PASS") -> (w1525:T4)  [unwired: 2 in]
                            n950 = local write "RESULT LAB03-1"(TRUE) -> ()
                            n951 = local write "DISP LAB03-1"(w1525) -> ()
                          }
                        }
                      }
                      frame False {
                      }
                    }
                  }
                }
              }
              frame #5 {
                # "LAB03-2"
                n952 = Equal?(x=w1528, y=2) -> (x = y?=w1531:bool)
                n953 = local read "DISP LAB03-2"() -> (w1533:T4)
                n954 = Unbundle(w1533) -> ("STATUS"=w1534:string)  [unwired: 2 out]
                n955 = Equal?(x=w1534, y="RUN") -> (x = y?=w1530:bool)
                n956 = And(x=w1530, y=w1531) -> (x .and. y?=w1529:bool)
                n957 = case shown="True" w1529 {
                  tunnel: w1533 -> [_ w1537]
                  tunnel: w1527 -> [_ w1540]
                  frame False {
                  }
                  frame True {
                    n958 = local read "SET LAB03-2"() -> (w1539:T5)
                    n959 = local read "DATA LAB03-2"() -> (w1536:refnum<k1>)
                    n960 = Unbundle(w1537) -> ("CYCLE"=w1541:dbl)  [unwired: 2 out]
                    n961 = Unbundle(w1539) -> ("T-RISE mins"=w1538:dbl)  [unwired: 4 out]
                    n962 = Greater Or Equal?(x=w1541, y=w1540) -> (x >= y?=w1542:bool)
                    n963 = case shown="True" w1542 {
                      tunnel: w1538 -> [w1545 _]
                      tunnel: w1537 -> [w1544 _]
                      tunnel: w1536 -> [w1543 _]
                      frame True {
                        n964 = stacked-sequence {
                          tunnel: w1545 -> [_ _]
                          tunnel: w1544 -> [_ w1548]
                          tunnel: w1543 -> [w1547 _]
                          frame #0 {
                            n965 = Close File(refnum=w1547) -> (error out=w1546:errorcluster)  [unwired: 1 in, 1 out]
                            n966 = local write "data file error"(w1546) -> ()
                          }
                          frame #1 {
                            n967 = Bundle(cluster=w1548, "STATUS"="T-RISE PASS") -> (w1550:T4)  [unwired: 2 in]
                            n968 = local write "RESULT LAB03-2"(TRUE) -> ()
                            n969 = local write "DISP LAB03-2"(w1550) -> ()
                          }
                        }
                      }
                      frame False {
                      }
                    }
                  }
                }
              }
              frame #6 {
                # "LAB04-1"
                n970 = Equal?(x=w1553, y=2) -> (x = y?=w1556:bool)
                n971 = local read "DISP LAB04-1"() -> (w1558:T4)
                n972 = Unbundle(w1558) -> ("STATUS"=w1559:string)  [unwired: 2 out]
                n973 = Equal?(x=w1559, y="RUN") -> (x = y?=w1555:bool)
                n974 = And(x=w1555, y=w1556) -> (x .and. y?=w1554:bool)
                n975 = case shown="True" w1554 {
                  tunnel: w1558 -> [_ w1562]
                  tunnel: w1552 -> [_ w1565]
                  frame False {
                  }
                  frame True {
                    n976 = local read "SET LAB04-1"() -> (w1564:T5)
                    n977 = local read "DATA LAB04-1"() -> (w1561:refnum<k1>)
                    n978 = Unbundle(w1562) -> ("CYCLE"=w1566:dbl)  [unwired: 2 out]
                    n979 = Unbundle(w1564) -> ("T-RISE mins"=w1563:dbl)  [unwired: 4 out]
                    n980 = Greater Or Equal?(x=w1566, y=w1565) -> (x >= y?=w1567:bool)
                    n981 = case shown="True" w1567 {
                      tunnel: w1563 -> [w1570 _]
                      tunnel: w1562 -> [w1569 _]
                      tunnel: w1561 -> [w1568 _]
                      frame True {
                        n982 = stacked-sequence {
                          tunnel: w1570 -> [_ _]
                          tunnel: w1569 -> [_ w1573]
                          tunnel: w1568 -> [w1572 _]
                          frame #0 {
                            n983 = Close File(refnum=w1572) -> (error out=w1571:errorcluster)  [unwired: 1 in, 1 out]
                            n984 = local write "data file error"(w1571) -> ()
                          }
                          frame #1 {
                            n985 = Bundle(cluster=w1573, "STATUS"="T-RISE PASS") -> (w1575:T4)  [unwired: 2 in]
                            n986 = local write "RESULT LAB04-1"(TRUE) -> ()
                            n987 = local write "DISP LAB04-1"(w1575) -> ()
                          }
                        }
                      }
                      frame False {
                      }
                    }
                  }
                }
              }
              frame #7 {
                # "LAB04-2"
                n988 = Equal?(x=w1578, y=2) -> (x = y?=w1581:bool)
                n989 = local read "DISP LAB04-2"() -> (w1583:T4)
                n990 = Unbundle(w1583) -> ("STATUS"=w1584:string)  [unwired: 2 out]
                n991 = Equal?(x=w1584, y="RUN") -> (x = y?=w1580:bool)
                n992 = And(x=w1580, y=w1581) -> (x .and. y?=w1579:bool)
                n993 = case shown="True" w1579 {
                  tunnel: w1583 -> [_ w1587]
                  tunnel: w1577 -> [_ w1590]
                  frame False {
                  }
                  frame True {
                    n994 = local read "SET LAB04-2"() -> (w1589:T5)
                    n995 = local read "DATA LAB04-2"() -> (w1586:refnum<k1>)
                    n996 = Unbundle(w1587) -> ("CYCLE"=w1591:dbl)  [unwired: 2 out]
                    n997 = Unbundle(w1589) -> ("T-RISE mins"=w1588:dbl)  [unwired: 4 out]
                    n998 = Greater Or Equal?(x=w1591, y=w1590) -> (x >= y?=w1592:bool)
                    n999 = case shown="True" w1592 {
                      tunnel: w1588 -> [w1595 _]
                      tunnel: w1587 -> [w1594 _]
                      tunnel: w1586 -> [w1593 _]
                      frame True {
                        n1000 = stacked-sequence {
                          tunnel: w1595 -> [_ _]
                          tunnel: w1594 -> [_ w1598]
                          tunnel: w1593 -> [w1597 _]
                          frame #0 {
                            n1001 = Close File(refnum=w1597) -> (error out=w1596:errorcluster)  [unwired: 1 in, 1 out]
                            n1002 = local write "data file error"(w1596) -> ()
                          }
                          frame #1 {
                            n1003 = Bundle(cluster=w1598, "STATUS"="T-RISE PASS") -> (w1600:T4)  [unwired: 2 in]
                            n1004 = local write "RESULT LAB04-2"(TRUE) -> ()
                            n1005 = local write "DISP LAB04-2"(w1600) -> ()
                          }
                        }
                      }
                      frame False {
                      }
                    }
                  }
                }
              }
              frame #8 {
                # "LAB05-1"
                n1006 = Equal?(x=w1603, y=2) -> (x = y?=w1606:bool)
                n1007 = local read "DISP LAB05-1"() -> (w1608:T4)
                n1008 = Unbundle(w1608) -> ("STATUS"=w1609:string)  [unwired: 2 out]
                n1009 = Equal?(x=w1609, y="RUN") -> (x = y?=w1605:bool)
                n1010 = And(x=w1605, y=w1606) -> (x .and. y?=w1604:bool)
                n1011 = case shown="True" w1604 {
                  tunnel: w1608 -> [_ w1612]
                  tunnel: w1602 -> [_ w1615]
                  frame False {
                  }
                  frame True {
                    n1012 = local read "SET LAB05-1"() -> (w1614:T5)
                    n1013 = local read "DATA LAB05-1"() -> (w1611:refnum<k1>)
                    n1014 = Unbundle(w1612) -> ("CYCLE"=w1616:dbl)  [unwired: 2 out]
                    n1015 = Unbundle(w1614) -> ("T-RISE mins"=w1613:dbl)  [unwired: 4 out]
                    n1016 = Greater Or Equal?(x=w1616, y=w1615) -> (x >= y?=w1617:bool)
                    n1017 = case shown="True" w1617 {
                      tunnel: w1613 -> [w1620 _]
                      tunnel: w1612 -> [w1619 _]
                      tunnel: w1611 -> [w1618 _]
                      frame True {
                        n1018 = stacked-sequence {
                          tunnel: w1620 -> [_ _]
                          tunnel: w1619 -> [_ w1623]
                          tunnel: w1618 -> [w1622 _]
                          frame #0 {
                            n1019 = Close File(refnum=w1622) -> (error out=w1621:errorcluster)  [unwired: 1 in, 1 out]
                            n1020 = local write "data file error"(w1621) -> ()
                          }
                          frame #1 {
                            n1021 = Bundle(cluster=w1623, "STATUS"="T-RISE PASS") -> (w1625:T4)  [unwired: 2 in]
                            n1022 = local write "RESULT LAB05-1"(TRUE) -> ()
                            n1023 = local write "DISP LAB05-1"(w1625) -> ()
                          }
                        }
                      }
                      frame False {
                      }
                    }
                  }
                }
              }
              frame #9 {
                # "LAB05-2"
                n1024 = Equal?(x=w1628, y=2) -> (x = y?=w1631:bool)
                n1025 = local read "DISP LAB05-2"() -> (w1633:T4)
                n1026 = Unbundle(w1633) -> ("STATUS"=w1634:string)  [unwired: 2 out]
                n1027 = Equal?(x=w1634, y="RUN") -> (x = y?=w1630:bool)
                n1028 = And(x=w1630, y=w1631) -> (x .and. y?=w1629:bool)
                n1029 = case shown="True" w1629 {
                  tunnel: w1633 -> [_ w1637]
                  tunnel: w1627 -> [_ w1640]
                  frame False {
                  }
                  frame True {
                    n1030 = local read "SET LAB05-2"() -> (w1639:T5)
                    n1031 = local read "DATA LAB05-2"() -> (w1636:refnum<k1>)
                    n1032 = Unbundle(w1637) -> ("CYCLE"=w1641:dbl)  [unwired: 2 out]
                    n1033 = Unbundle(w1639) -> ("T-RISE mins"=w1638:dbl)  [unwired: 4 out]
                    n1034 = Greater Or Equal?(x=w1641, y=w1640) -> (x >= y?=w1642:bool)
                    n1035 = case shown="True" w1642 {
                      tunnel: w1638 -> [w1645 _]
                      tunnel: w1637 -> [w1644 _]
                      tunnel: w1636 -> [w1643 _]
                      frame True {
                        n1036 = stacked-sequence {
                          tunnel: w1645 -> [_ _]
                          tunnel: w1644 -> [_ w1648]
                          tunnel: w1643 -> [w1647 _]
                          frame #0 {
                            n1037 = Close File(refnum=w1647) -> (error out=w1646:errorcluster)  [unwired: 1 in, 1 out]
                            n1038 = local write "data file error"(w1646) -> ()
                          }
                          frame #1 {
                            n1039 = Bundle(cluster=w1648, "STATUS"="T-RISE PASS") -> (w1650:T4)  [unwired: 2 in]
                            n1040 = local write "RESULT LAB05-2"(TRUE) -> ()
                            n1041 = local write "DISP LAB05-2"(w1650) -> ()
                          }
                        }
                      }
                      frame False {
                      }
                    }
                  }
                }
              }
            }
          }
          frame #6 {
            # "end test & close test files"
            n1042 = stacked-sequence {
              tunnel: w1661 -> [_ _ _ _ _ _ _ _ _ _]
              tunnel: w1662 -> [_ _ _ _ _ _ _ _ _ _]
              tunnel: w1660 -> [_ _ _ _ _ _ _ _ _ _]
              tunnel: w1659 -> [_ _ _ _ _ _ _ _ _ _]
              tunnel: w1658 -> [_ _ _ _ _ _ _ _ _ _]
              tunnel: w1657 -> [_ _ _ _ _ _ _ _ _ _]
              tunnel: w1656 -> [_ _ _ _ _ _ _ _ _ _]
              tunnel: w1655 -> [_ _ _ _ _ _ _ _ _ _]
              tunnel: w1654 -> [_ _ _ _ _ _ _ _ _ _]
              tunnel: w1653 -> [_ _ _ _ _ _ _ _ _ _]
              frame #0 {
                # "LAB01-1"
                n1043 = local read "DISP LAB01-1"() -> (w1666:T4)
                n1044 = local read "run lab01-1"() -> (w1663:bool)
                n1045 = local read "DATA LAB01-1"() -> (w1664:refnum<k1>)
                n1046 = Unbundle(w1666) -> ("CYCLE"=w1667:dbl, "STATUS"=w1665:string)  [unwired: 1 out]
                n1047 = case shown="True" w1663 {
                  tunnel: w1667 -> [_ w1671]
                  tunnel: w1666 -> [_ w1670]
                  tunnel: w1665 -> [_ w1669]
                  tunnel: w1664 -> [_ w1668]
                  frame False {
                  }
                  frame True {
                    n1048 = Not Equal?(x=w1669, y="RUN") -> (x != y?=w1672:bool)
                    n1049 = Greater?(x=w1671, y=2.0) -> (0:w1674:bool)
                    n1050 = And(x=w1674, y=w1672) -> (x .and. y?=w1673:bool)
                    n1051 = case shown="True" w1673 {
                      tunnel: w1670 -> [_ w1678]
                      tunnel: w1668 -> [_ w1677]
                      frame False {
                      }
                      frame True {
                        n1052 = stacked-sequence {
                          tunnel: w1678 -> [w1681 _ _]
                          tunnel: w1677 -> [_ _ _]
                          frame #0 {
                            n1053 = local write "mail control"("END") -> ()
                            n1054 = Bundle(cluster=w1681) -> (w1680:T4)  [unwired: 3 in]
                            n1055 = local write "DISP LAB01-1"(w1680) -> ()
                          }
                          frame #1 {
                            n1056 = local read "DATA LAB01-1"() -> (w1683:refnum<k1>)
                            n1057 = Close File(refnum=w1683) -> (error out=w1682:errorcluster)  [unwired: 1 in, 1 out]
                            n1058 = local write "data file error"(w1682) -> ()
                          }
                          frame #2 {
                            w1684 = FALSE
                            n1059 = local write "run lab01-1"(w1684) -> ()
                            n1060 = local write "RUN LAB01-1"(w1684) -> ()
                            n1061 = call "Save data file to network drive v1.vi"("panel id"="LAB01-1") -> ("network file save error"=w1685:errorcluster)  [unwired: 9 in, 1 out]
                            n1062 = local write "data file error"(w1685) -> ()
                          }
                        }
                      }
                    }
                  }
                }
              }
              frame #1 {
                # "LAB01-2"
                n1063 = local read "run lab01-2"() -> (w1687:bool)
                n1064 = case shown="True" w1687 {
                  frame False {
                  }
                  frame True {
                    n1065 = local read "DISP LAB01-2"() -> (w1694:T4)
                    n1066 = local read "DATA LAB01-2"() -> (w1693:refnum<k1>)
                    n1067 = Unbundle(w1694) -> ("CYCLE"=w1690:dbl, "STATUS"=w1695:string)  [unwired: 1 out]
                    n1068 = Not Equal?(x=w1695, y="RUN") -> (x != y?=w1689:bool)
                    n1069 = Greater?(x=w1690, y=2.0) -> (0:w1691:bool)
                    n1070 = And(x=w1691, y=w1689) -> (x .and. y?=w1688:bool)
                    n1071 = case shown="True" w1688 {
                      tunnel: w1694 -> [_ w1698]
                      tunnel: w1693 -> [_ w1697]
                      frame False {
                      }
                      frame True {
                        n1072 = stacked-sequence {
                          tunnel: w1698 -> [w1701 _ _]
                          tunnel: w1697 -> [_ w1704 _]
                          frame #0 {
                            w1699 = FALSE
                            n1073 = local write "mail control"("END") -> ()
                            n1074 = Bundle(cluster=w1701) -> (w1702:T4)  [unwired: 3 in]
                            n1075 = local write "RUN LAB01-2"(w1699) -> ()
                            n1076 = local write "run lab01-2"(w1699) -> ()
                            n1077 = local write "DISP LAB01-2"(w1702) -> ()
                          }
                          frame #1 {
                            n1078 = Close File(refnum=w1704) -> (error out=w1703:errorcluster)  [unwired: 1 in, 1 out]
                            n1079 = local write "data file error"(w1703) -> ()
                          }
                          frame #2 {
                            n1080 = call "Save data file to network drive v1.vi"("panel id"="LAB01-2") -> ("network file save error"=w1705:errorcluster)  [unwired: 9 in, 1 out]
                            n1081 = local write "data file error"(w1705) -> ()
                          }
                        }
                      }
                    }
                  }
                }
              }
              frame #2 {
                # "LAB02-1"
                n1082 = local read "run lab02-1"() -> (w1707:bool)
                n1083 = case shown="True" w1707 {
                  frame False {
                  }
                  frame True {
                    n1084 = local read "DISP LAB02-1"() -> (w1714:T4)
                    n1085 = Unbundle(w1714) -> ("CYCLE"=w1710:dbl, "STATUS"=w1715:string)  [unwired: 1 out]
                    n1086 = local read "DATA LAB02-1"() -> (w1713:refnum<k1>)
                    n1087 = Not Equal?(x=w1715, y="RUN") -> (x != y?=w1709:bool)
                    n1088 = Greater?(x=w1710, y=2.0) -> (0:w1711:bool)
                    n1089 = And(x=w1711, y=w1709) -> (x .and. y?=w1708:bool)
                    n1090 = case shown="True" w1708 {
                      tunnel: w1714 -> [_ w1718]
                      tunnel: w1713 -> [_ w1717]
                      frame False {
                      }
                      frame True {
                        n1091 = stacked-sequence {
                          tunnel: w1718 -> [w1721 _ _]
                          tunnel: w1717 -> [_ w1724 _]
                          frame #0 {
                            w1719 = FALSE
                            n1092 = local write "mail control"("END") -> ()
                            n1093 = Bundle(cluster=w1721) -> (w1722:T4)  [unwired: 3 in]
                            n1094 = local write "RUN LAB02-1"(w1719) -> ()
                            n1095 = local write "run lab02-1"(w1719) -> ()
                            n1096 = local write "DISP LAB02-1"(w1722) -> ()
                          }
                          frame #1 {
                            n1097 = Close File(refnum=w1724) -> (error out=w1723:errorcluster)  [unwired: 1 in, 1 out]
                            n1098 = local write "data file error"(w1723) -> ()
                          }
                          frame #2 {
                            n1099 = call "Save data file to network drive v1.vi"("panel id"="LAB02-1") -> ("network file save error"=w1725:errorcluster)  [unwired: 9 in, 1 out]
                            n1100 = local write "data file error"(w1725) -> ()
                          }
                        }
                      }
                    }
                  }
                }
              }
              frame #3 {
                # "LAB02-2"
                n1101 = local read "run lab02-2"() -> (w1727:bool)
                n1102 = case shown="True" w1727 {
                  frame False {
                  }
                  frame True {
                    n1103 = local read "DISP LAB02-2"() -> (w1734:T4)
                    n1104 = local read "DATA LAB02-2"() -> (w1733:refnum<k1>)
                    n1105 = Unbundle(w1734) -> ("CYCLE"=w1730:dbl, "STATUS"=w1735:string)  [unwired: 1 out]
                    n1106 = Not Equal?(x=w1735, y="RUN") -> (x != y?=w1729:bool)
                    n1107 = Greater?(x=w1730, y=2.0) -> (0:w1731:bool)
                    n1108 = And(x=w1731, y=w1729) -> (x .and. y?=w1728:bool)
                    n1109 = case shown="True" w1728 {
                      tunnel: w1734 -> [_ w1738]
                      tunnel: w1733 -> [_ w1737]
                      frame False {
                      }
                      frame True {
                        n1110 = stacked-sequence {
                          tunnel: w1738 -> [w1741 _ _]
                          tunnel: w1737 -> [_ w1744 _]
                          frame #0 {
                            w1739 = FALSE
                            n1111 = local write "mail control"("END") -> ()
                            n1112 = Bundle(cluster=w1741) -> (w1742:T4)  [unwired: 3 in]
                            n1113 = local write "run lab02-2"(w1739) -> ()
                            n1114 = local write "RUN LAB02-2"(w1739) -> ()
                            n1115 = local write "DISP LAB02-2"(w1742) -> ()
                          }
                          frame #1 {
                            n1116 = Close File(refnum=w1744) -> (error out=w1743:errorcluster)  [unwired: 1 in, 1 out]
                            n1117 = local write "data file error"(w1743) -> ()
                          }
                          frame #2 {
                            n1118 = call "Save data file to network drive v1.vi"("panel id"="LAB02-2") -> ("network file save error"=w1745:errorcluster)  [unwired: 9 in, 1 out]
                            n1119 = local write "data file error"(w1745) -> ()
                          }
                        }
                      }
                    }
                  }
                }
              }
              frame #4 {
                # "LAB03-1"
                n1120 = local read "run lab03-1"() -> (w1747:bool)
                n1121 = case shown="True" w1747 {
                  frame False {
                  }
                  frame True {
                    n1122 = local read "DISP LAB03-1"() -> (w1754:T4)
                    n1123 = local read "DATA LAB03-1"() -> (w1753:refnum<k1>)
                    n1124 = Unbundle(w1754) -> ("CYCLE"=w1750:dbl, "STATUS"=w1755:string)  [unwired: 1 out]
                    n1125 = Not Equal?(x=w1755, y="RUN") -> (x != y?=w1749:bool)
                    n1126 = Greater?(x=w1750, y=2.0) -> (0:w1751:bool)
                    n1127 = And(x=w1751, y=w1749) -> (x .and. y?=w1748:bool)
                    n1128 = case shown="True" w1748 {
                      tunnel: w1754 -> [_ w1758]
                      tunnel: w1753 -> [_ w1757]
                      frame False {
                      }
                      frame True {
                        n1129 = stacked-sequence {
                          tunnel: w1758 -> [w1761 _ _]
                          tunnel: w1757 -> [_ w1764 _]
                          frame #0 {
                            w1759 = FALSE
                            n1130 = local write "mail control"("END") -> ()
                            n1131 = Bundle(cluster=w1761) -> (w1762:T4)  [unwired: 3 in]
                            n1132 = local write "run lab03-1"(w1759) -> ()
                            n1133 = local write "RUN LAB03-1"(w1759) -> ()
                            n1134 = local write "DISP LAB03-1"(w1762) -> ()
                          }
                          frame #1 {
                            n1135 = Close File(refnum=w1764) -> (error out=w1763:errorcluster)  [unwired: 1 in, 1 out]
                            n1136 = local write "data file error"(w1763) -> ()
                          }
                          frame #2 {
                            n1137 = call "Save data file to network drive v1.vi"("panel id"="LAB03-1") -> ("network file save error"=w1765:errorcluster)  [unwired: 9 in, 1 out]
                            n1138 = local write "data file error"(w1765) -> ()
                          }
                        }
                      }
                    }
                  }
                }
              }
              frame #5 {
                # "LAB03-2"
                n1139 = local read "run lab03-2"() -> (w1767:bool)
                n1140 = case shown="True" w1767 {
                  frame False {
                  }
                  frame True {
                    n1141 = local read "DISP LAB03-2"() -> (w1774:T4)
                    n1142 = Unbundle(w1774) -> ("CYCLE"=w1770:dbl, "STATUS"=w1775:string)  [unwired: 1 out]
                    n1143 = local read "DATA LAB03-2"() -> (w1773:refnum<k1>)
                    n1144 = Not Equal?(x=w1775, y="RUN") -> (x != y?=w1769:bool)
                    n1145 = Greater?(x=w1770, y=2.0) -> (0:w1771:bool)
                    n1146 = And(x=w1771, y=w1769) -> (x .and. y?=w1768:bool)
                    n1147 = case shown="True" w1768 {
                      tunnel: w1774 -> [_ w1778]
                      tunnel: w1773 -> [_ w1777]
                      frame False {
                      }
                      frame True {
                        n1148 = stacked-sequence {
                          tunnel: w1778 -> [w1781 _ _]
                          tunnel: w1777 -> [_ w1784 _]
                          frame #0 {
                            w1779 = FALSE
                            n1149 = local write "mail control"("END") -> ()
                            n1150 = Bundle(cluster=w1781) -> (w1782:T4)  [unwired: 3 in]
                            n1151 = local write "RUN LAB03-2"(w1779) -> ()
                            n1152 = local write "DISP LAB03-2"(w1782) -> ()
                            n1153 = local write "run lab03-2"(w1779) -> ()
                          }
                          frame #1 {
                            n1154 = Close File(refnum=w1784) -> (error out=w1783:errorcluster)  [unwired: 1 in, 1 out]
                            n1155 = local write "data file error"(w1783) -> ()
                          }
                          frame #2 {
                            n1156 = call "Save data file to network drive v1.vi"("panel id"="LAB03-2") -> ("network file save error"=w1785:errorcluster)  [unwired: 9 in, 1 out]
                            n1157 = local write "data file error"(w1785) -> ()
                          }
                        }
                      }
                    }
                  }
                }
              }
              frame #6 {
                # "LAB04-1"
                n1158 = local read "run lab04-1"() -> (w1787:bool)
                n1159 = case shown="True" w1787 {
                  frame False {
                  }
                  frame True {
                    n1160 = local read "DISP LAB04-1"() -> (w1794:T4)
                    n1161 = Unbundle(w1794) -> ("CYCLE"=w1790:dbl, "STATUS"=w1795:string)  [unwired: 1 out]
                    n1162 = local read "DATA LAB04-1"() -> (w1793:refnum<k1>)
                    n1163 = Not Equal?(x=w1795, y="RUN") -> (x != y?=w1789:bool)
                    n1164 = Greater?(x=w1790, y=2.0) -> (0:w1791:bool)
                    n1165 = And(x=w1791, y=w1789) -> (x .and. y?=w1788:bool)
                    n1166 = case shown="True" w1788 {
                      tunnel: w1794 -> [_ w1798]
                      tunnel: w1793 -> [_ w1797]
                      frame False {
                      }
                      frame True {
                        n1167 = stacked-sequence {
                          tunnel: w1798 -> [w1801 _ _]
                          tunnel: w1797 -> [_ w1804 _]
                          frame #0 {
                            w1799 = FALSE
                            n1168 = local write "mail control"("END") -> ()
                            n1169 = Bundle(cluster=w1801) -> (w1802:T4)  [unwired: 3 in]
                            n1170 = local write "RUN LAB04-1"(w1799) -> ()
                            n1171 = local write "run lab04-1"(w1799) -> ()
                            n1172 = local write "DISP LAB04-1"(w1802) -> ()
                          }
                          frame #1 {
                            n1173 = Close File(refnum=w1804) -> (error out=w1803:errorcluster)  [unwired: 1 in, 1 out]
                            n1174 = local write "data file error"(w1803) -> ()
                          }
                          frame #2 {
                            n1175 = call "Save data file to network drive v1.vi"("panel id"="LAB04-1") -> ("network file save error"=w1805:errorcluster)  [unwired: 9 in, 1 out]
                            n1176 = local write "data file error"(w1805) -> ()
                          }
                        }
                      }
                    }
                  }
                }
              }
              frame #7 {
                # "LAB04-2"
                n1177 = local read "run lab04-2"() -> (w1807:bool)
                n1178 = case shown="True" w1807 {
                  frame False {
                  }
                  frame True {
                    n1179 = local read "DISP LAB04-2"() -> (w1814:T4)
                    n1180 = Unbundle(w1814) -> ("CYCLE"=w1810:dbl, "STATUS"=w1815:string)  [unwired: 1 out]
                    n1181 = Not Equal?(x=w1815, y="RUN") -> (x != y?=w1809:bool)
                    n1182 = local read "DATA LAB04-2"() -> (w1813:refnum<k1>)
                    n1183 = Greater?(x=w1810, y=2.0) -> (0:w1811:bool)
                    n1184 = And(x=w1811, y=w1809) -> (x .and. y?=w1808:bool)
                    n1185 = case shown="True" w1808 {
                      tunnel: w1814 -> [_ w1818]
                      tunnel: w1813 -> [_ w1817]
                      frame False {
                      }
                      frame True {
                        n1186 = stacked-sequence {
                          tunnel: w1818 -> [w1821 _ _]
                          tunnel: w1817 -> [_ w1824 _]
                          frame #0 {
                            w1819 = FALSE
                            n1187 = local write "mail control"("END") -> ()
                            n1188 = Bundle(cluster=w1821) -> (w1822:T4)  [unwired: 3 in]
                            n1189 = local write "RUN LAB04-2"(w1819) -> ()
                            n1190 = local write "run lab04-2"(w1819) -> ()
                            n1191 = local write "DISP LAB04-2"(w1822) -> ()
                          }
                          frame #1 {
                            n1192 = Close File(refnum=w1824) -> (error out=w1823:errorcluster)  [unwired: 1 in, 1 out]
                            n1193 = local write "data file error"(w1823) -> ()
                          }
                          frame #2 {
                            n1194 = call "Save data file to network drive v1.vi"("panel id"="LAB04-2") -> ("network file save error"=w1825:errorcluster)  [unwired: 9 in, 1 out]
                            n1195 = local write "data file error"(w1825) -> ()
                          }
                        }
                      }
                    }
                  }
                }
              }
              frame #8 {
                # "LAB05-1"
                n1196 = local read "run lab05-1"() -> (w1827:bool)
                n1197 = case shown="True" w1827 {
                  frame False {
                  }
                  frame True {
                    n1198 = local read "DISP LAB05-1"() -> (w1834:T4)
                    n1199 = Unbundle(w1834) -> ("CYCLE"=w1830:dbl, "STATUS"=w1835:string)  [unwired: 1 out]
                    n1200 = Not Equal?(x=w1835, y="RUN") -> (x != y?=w1829:bool)
                    n1201 = local read "DATA LAB05-1"() -> (w1833:refnum<k1>)
                    n1202 = Greater?(x=w1830, y=2.0) -> (0:w1831:bool)
                    n1203 = And(x=w1831, y=w1829) -> (x .and. y?=w1828:bool)
                    n1204 = case shown="True" w1828 {
                      tunnel: w1834 -> [_ w1838]
                      tunnel: w1833 -> [_ w1837]
                      frame False {
                      }
                      frame True {
                        n1205 = stacked-sequence {
                          tunnel: w1838 -> [w1841 _ _]
                          tunnel: w1837 -> [_ w1844 _]
                          frame #0 {
                            w1839 = FALSE
                            n1206 = local write "mail control"("END") -> ()
                            n1207 = Bundle(cluster=w1841) -> (w1842:T4)  [unwired: 3 in]
                            n1208 = local write "RUN LAB05-1"(w1839) -> ()
                            n1209 = local write "run lab05-1"(w1839) -> ()
                            n1210 = local write "DISP LAB05-1"(w1842) -> ()
                          }
                          frame #1 {
                            n1211 = Close File(refnum=w1844) -> (error out=w1843:errorcluster)  [unwired: 1 in, 1 out]
                            n1212 = local write "data file error"(w1843) -> ()
                          }
                          frame #2 {
                            n1213 = call "Save data file to network drive v1.vi"("panel id"="LAB05-1") -> ("network file save error"=w1845:errorcluster)  [unwired: 9 in, 1 out]
                            n1214 = local write "data file error"(w1845) -> ()
                          }
                        }
                      }
                    }
                  }
                }
              }
              frame #9 {
                # "LAB05-2"
                n1215 = local read "run lab05-2"() -> (w1847:bool)
                n1216 = case shown="True" w1847 {
                  frame False {
                  }
                  frame True {
                    n1217 = local read "DISP LAB05-2"() -> (w1854:T4)
                    n1218 = Unbundle(w1854) -> ("CYCLE"=w1850:dbl, "STATUS"=w1855:string)  [unwired: 1 out]
                    n1219 = Not Equal?(x=w1855, y="RUN") -> (x != y?=w1849:bool)
                    n1220 = local read "DATA LAB05-2"() -> (w1853:refnum<k1>)
                    n1221 = Greater?(x=w1850, y=2.0) -> (0:w1851:bool)
                    n1222 = And(x=w1851, y=w1849) -> (x .and. y?=w1848:bool)
                    n1223 = case shown="True" w1848 {
                      tunnel: w1854 -> [_ w1858]
                      tunnel: w1853 -> [_ w1857]
                      frame False {
                      }
                      frame True {
                        n1224 = stacked-sequence {
                          tunnel: w1858 -> [w1861 _ _]
                          tunnel: w1857 -> [_ w1864 _]
                          frame #0 {
                            w1859 = FALSE
                            n1225 = local write "mail control"("END") -> ()
                            n1226 = Bundle(cluster=w1861) -> (w1862:T4)  [unwired: 3 in]
                            n1227 = local write "RUN LAB05-2"(w1859) -> ()
                            n1228 = local write "run lab05-2"(w1859) -> ()
                            n1229 = local write "DISP LAB05-2"(w1862) -> ()
                          }
                          frame #1 {
                            n1230 = Close File(refnum=w1864) -> (error out=w1863:errorcluster)  [unwired: 1 in, 1 out]
                            n1231 = local write "data file error"(w1863) -> ()
                          }
                          frame #2 {
                            n1232 = call "Save data file to network drive v1.vi"("panel id"="LAB05-2") -> ("network file save error"=w1865:errorcluster)  [unwired: 9 in, 1 out]
                            n1233 = local write "data file error"(w1865) -> ()
                          }
                        }
                      }
                    }
                  }
                }
              }
            }
            n1234 = local read "Network Directory"() -> (w1652:path)
            n1235 = global write "Global 1.vi" "Network Drive"(w1652) -> ()
          }
          frame #7 {
            # "disable functions"
            n1236 = stacked-sequence {
              tunnel: w1876 -> [w1890 _ w1946]
              tunnel: w1875 -> [w1885 _ w1945]
              tunnel: w1874 -> [w1884 _ w1944]
              tunnel: w1873 -> [w1882 _ w1943]
              tunnel: w1872 -> [w1883 _ w1942]
              tunnel: w1871 -> [_ w1907 w1941]
              tunnel: w1870 -> [_ w1908 w1940]
              tunnel: w1869 -> [_ w1909 w1939]
              tunnel: w1868 -> [_ w1910 w1938]
              tunnel: w1867 -> [_ w1911 w1937]
              frame #0 {
                n1237 = Select(t=2, s=w1882, f=0) -> (s? t:f=w1878:i32)
                n1238 = Select(t=2, s=w1884, f=0) -> (s? t:f=w1879:i32)
                n1239 = Select(t=2, s=w1883, f=0) -> (s? t:f=w1877:i32)
                n1240 = Select(t=2, s=w1890, f=0) -> (s? t:f=w1881:i32)
                n1241 = Select(t=2, s=w1885, f=0) -> (s? t:f=w1880:i32)
                n1242 = property on="SELECT LAB02-2" class="RadioBtnsControl (strict)"("DisabledEnum"=w1878) -> ()  [unwired: 2 in, 2 out]
                n1243 = property on="SELECT LAB02-1" class="RadioBtnsControl (strict)"("DisabledEnum"=w1879) -> ()  [unwired: 2 in, 2 out]
                n1244 = property on="SELECT LAB03-1" class="RadioBtnsControl (strict)"("DisabledEnum"=w1877) -> ()  [unwired: 2 in, 2 out]
                n1245 = property on="SELECT LAB01-1" class="RadioBtnsControl (strict)"("DisabledEnum"=w1881) -> ()  [unwired: 2 in, 2 out]
                n1246 = property on="SELECT LAB01-2" class="RadioBtnsControl (strict)"("DisabledEnum"=w1880) -> ()  [unwired: 2 in, 2 out]
                n1247 = Not(x=w1890) -> (.not. x?=w1891:bool)
                n1248 = property on="RESULT LAB01-1" class="Bool (strict)"("Visible"=w1891) -> ()  [unwired: 2 in, 2 out]
                n1249 = Not(x=w1885) -> (.not. x?=w1889:bool)
                n1250 = Not(x=w1884) -> (.not. x?=w1888:bool)
                n1251 = Not(x=w1882) -> (.not. x?=w1887:bool)
                n1252 = property on="RESULT LAB01-2" class="Bool (strict)"("Visible"=w1889) -> ()  [unwired: 2 in, 2 out]
                n1253 = Not(x=w1883) -> (.not. x?=w1886:bool)
                n1254 = property on="RESULT LAB02-1" class="Bool (strict)"("Visible"=w1888) -> ()  [unwired: 2 in, 2 out]
                n1255 = property on="RESULT LAB02-2" class="Bool (strict)"("Visible"=w1887) -> ()  [unwired: 2 in, 2 out]
                n1256 = property on="RESULT LAB03-1" class="Bool (strict)"("Visible"=w1886) -> ()  [unwired: 2 in, 2 out]
                n1257 = property on="SET LAB01-1" class="Clust (strict)"("DisabledEnum"=w1881) -> ()  [unwired: 2 in, 2 out]
                n1258 = property on="SET LAB01-2" class="Clust (strict)"("DisabledEnum"=w1880) -> ()  [unwired: 2 in, 2 out]
                n1259 = property on="SET LAB02-1" class="Clust (strict)"("DisabledEnum"=w1879) -> ()  [unwired: 2 in, 2 out]
                n1260 = property on="SET LAB02-2" class="Clust (strict)"("DisabledEnum"=w1878) -> ()  [unwired: 2 in, 2 out]
                n1261 = property on="SET LAB03-1" class="Clust (strict)"("DisabledEnum"=w1877) -> ()  [unwired: 2 in, 2 out]
                n1262 = property on="O/I  LAB01-1" class="Bool (strict)"("DisabledEnum"=w1881) -> ()  [unwired: 2 in, 2 out]
                n1263 = property on="O/I  LAB01-2" class="Bool (strict)"("DisabledEnum"=w1880) -> ()  [unwired: 2 in, 2 out]
                n1264 = property on="O/I  LAB02-1" class="Bool (strict)"("DisabledEnum"=w1879) -> ()  [unwired: 2 in, 2 out]
                n1265 = property on="O/1  LAB02-2" class="Bool (strict)"("DisabledEnum"=w1878) -> ()  [unwired: 2 in, 2 out]
                n1266 = property on="O/I  LAB03-1" class="Bool (strict)"("DisabledEnum"=w1877) -> ()  [unwired: 2 in, 2 out]
              }
              frame #1 {
                n1267 = Select(t=2, s=w1911, f=0) -> (s? t:f=w1902:i32)
                n1268 = Select(t=2, s=w1910, f=0) -> (s? t:f=w1903:i32)
                n1269 = Select(t=2, s=w1907, f=0) -> (s? t:f=w1906:i32)
                n1270 = Select(t=2, s=w1908, f=0) -> (s? t:f=w1905:i32)
                n1271 = Select(t=2, s=w1909, f=0) -> (s? t:f=w1904:i32)
                n1272 = property on="SELECT LAB05-2" class="RadioBtnsControl (strict)"("DisabledEnum"=w1902) -> ()  [unwired: 2 in, 2 out]
                n1273 = property on="SELECT LAB05-1" class="RadioBtnsControl (strict)"("DisabledEnum"=w1903) -> ()  [unwired: 2 in, 2 out]
                n1274 = property on="SELECT LAB03-2" class="RadioBtnsControl (strict)"("DisabledEnum"=w1906) -> ()  [unwired: 2 in, 2 out]
                n1275 = property on="SELECT LAB04-1" class="RadioBtnsControl (strict)"("DisabledEnum"=w1905) -> ()  [unwired: 2 in, 2 out]
                n1276 = property on="SELECT LAB04-2" class="RadioBtnsControl (strict)"("DisabledEnum"=w1904) -> ()  [unwired: 2 in, 2 out]
                n1277 = property on="SET LAB05-2" class="Clust (strict)"("DisabledEnum"=w1902) -> ()  [unwired: 2 in, 2 out]
                n1278 = property on="SET LAB05-1" class="Clust (strict)"("DisabledEnum"=w1903) -> ()  [unwired: 2 in, 2 out]
                n1279 = property on="SET LAB03-2" class="Clust (strict)"("DisabledEnum"=w1906) -> ()  [unwired: 2 in, 2 out]
                n1280 = property on="SET LAB04-1" class="Clust (strict)"("DisabledEnum"=w1905) -> ()  [unwired: 2 in, 2 out]
                n1281 = property on="SET LAB04-2" class="Clust (strict)"("DisabledEnum"=w1904) -> ()  [unwired: 2 in, 2 out]
                n1282 = property on="O/I  LAB05-2" class="Bool (strict)"("DisabledEnum"=w1902) -> ()  [unwired: 2 in, 2 out]
                n1283 = property on="O/I  LAB05-1" class="Bool (strict)"("DisabledEnum"=w1903) -> ()  [unwired: 2 in, 2 out]
                n1284 = property on="O/I  LAB04-1" class="Bool (strict)"("DisabledEnum"=w1905) -> ()  [unwired: 2 in, 2 out]
                n1285 = property on="O/I  LAB04-2" class="Bool (strict)"("DisabledEnum"=w1904) -> ()  [unwired: 2 in, 2 out]
                n1286 = property on="O/I  LAB03-2" class="Bool (strict)"("DisabledEnum"=w1906) -> ()  [unwired: 2 in, 2 out]
                n1287 = Not(x=w1911) -> (.not. x?=w1912:bool)
                n1288 = Not(x=w1910) -> (.not. x?=w1913:bool)
                n1289 = Not(x=w1909) -> (.not. x?=w1914:bool)
                n1290 = property on="RESULT LAB05-2" class="Bool (strict)"("Visible"=w1912) -> ()  [unwired: 2 in, 2 out]
                n1291 = property on="RESULT LAB05-1" class="Bool (strict)"("Visible"=w1913) -> ()  [unwired: 2 in, 2 out]
                n1292 = Not(x=w1908) -> (.not. x?=w1915:bool)
                n1293 = property on="RESULT LAB04-2" class="Bool (strict)"("Visible"=w1914) -> ()  [unwired: 2 in, 2 out]
                n1294 = Not(x=w1907) -> (.not. x?=w1916:bool)
                n1295 = property on="RESULT LAB04-1" class="Bool (strict)"("Visible"=w1915) -> ()  [unwired: 2 in, 2 out]
                n1296 = property on="RESULT LAB03-2" class="Bool (strict)"("Visible"=w1916) -> ()  [unwired: 2 in, 2 out]
              }
              frame #2 {
                # "disable calibrate if any test running"
                n1297 = Or(x=w1938, y=w1937) -> (x .or. y?=w1931:bool)
                n1298 = Or(x=w1940, y=w1939) -> (x .or. y?=w1933:bool)
                n1299 = Or(x=w1944, y=w1943) -> (x .or. y?=w1935:bool)
                n1300 = Or(x=w1942, y=w1941) -> (x .or. y?=w1934:bool)
                n1301 = Or(x=w1946, y=w1945) -> (x .or. y?=w1936:bool)
                n1302 = Or(x=w1934, y=w1933) -> (x .or. y?=w1932:bool)
                n1303 = Or(x=w1936, y=w1935) -> (x .or. y?=w1930:bool)
                n1304 = Or(x=w1932, y=w1931) -> (x .or. y?=w1929:bool)
                n1305 = Or(x=w1930, y=w1929) -> (x .or. y?=w1928:bool)
                n1306 = case shown="False" w1928 {
                  tunnel: [0 2] -> w1927
                  frame False {
                  }
                  frame True {
                  }
                }
                n1307 = property on="TO (string):" class="Str"("DisabledEnum"=w1927) -> ()  [unwired: 2 in, 2 out]
                n1308 = property on="Network Directory" class="Path"("DisabledEnum"=w1927) -> ()  [unwired: 2 in, 2 out]
                n1309 = property on="MAIL SETTINGS" class="Clust (strict)"("DisabledEnum"=w1927) -> ()  [unwired: 2 in, 2 out]
                n1310 = property on="CALIBRATE" class="Bool (strict)"("DisabledEnum"=w1927) -> ()  [unwired: 2 in, 2 out]
                n1311 = property on="SHOW ADMIN PAGE" class="Bool (strict)"("DisabledEnum"=w1927) -> ()  [unwired: 2 in, 2 out]
              }
            }
          }
          frame #8 {
            # "drive jigs"
            n1312 = stacked-sequence {
              frame #0 {
                # "jig on"
                n1313 = local read "jig cycle"() -> (w1949:dbl)
                n1314 = Equal?(x=w1949, y=0) -> (x = y?=w1951:bool)
                n1315 = case shown="True" w1951 {
                  frame False {
                  }
                  frame True {
                    n1316 = local read "RUN LAB01-1"() -> (w1952:bool)
                    n1317 = local read "RUN LAB01-2"() -> (w1953:bool)
                    n1318 = local read "RUN LAB03-1"() -> (w1959:bool)
                    n1319 = local read "RUN LAB03-2"() -> (w1958:bool)
                    n1320 = local read "RUN LAB02-1"() -> (w1961:bool)
                    n1321 = local read "RUN LAB02-2"() -> (w1960:bool)
                    n1322 = local read "RUN LAB04-1"() -> (w1957:bool)
                    n1323 = local read "RUN LAB04-2"() -> (w1956:bool)
                    n1324 = local read "RUN LAB05-1"() -> (w1955:bool)
                    n1325 = local read "RUN LAB05-2"() -> (w1954:bool)
                    n1326 = local write "JIG LAB05-1"(w1955) -> ()
                    n1327 = local write "JIG LAB05-2"(w1954) -> ()
                    n1328 = local write "JIG LAB04-2"(w1956) -> ()
                    n1329 = local write "JIG LAB02-1"(w1961) -> ()
                    n1330 = local write "JIG LAB03-1"(w1959) -> ()
                    n1331 = local write "JIG LAB04-1"(w1957) -> ()
                    n1332 = local write "JIG LAB03-2"(w1958) -> ()
                    n1333 = local write "JIG LAB02-2"(w1960) -> ()
                    n1334 = local write "JIG LAB01-1"(w1952) -> ()
                    n1335 = local write "JIG LAB01-2"(w1953) -> ()
                  }
                }
              }
              frame #1 {
                # "jig off"
                n1336 = local read "jig cycle"() -> (w1964:dbl)
                n1337 = local read "on loops"() -> (w1963:dbl)
                n1338 = Equal?(x=w1964, y=w1963) -> (x = y?=w1962:bool)
                n1339 = case shown="True" w1962 {
                  frame False {
                  }
                  frame True {
                    w2015 = FALSE
                    w2016 = TRUE
                    w2014 = 2
                    n1340 = local read "SELECT LAB05-2"() -> (w2005:T3)
                    n1341 = local read "SELECT LAB04-2"() -> (w2007:T3)
                    n1342 = local read "SELECT LAB04-1"() -> (w2008:T3)
                    n1343 = local read "SELECT LAB05-1"() -> (w2006:T3)
                    n1344 = local read "SELECT LAB03-2"() -> (w2009:T3)
                    n1345 = local read "SELECT LAB02-1"() -> (w2012:T3)
                    n1346 = local read "SELECT LAB03-1"() -> (w2010:T3)
                    n1347 = local read "SELECT LAB02-2"() -> (w2011:T3)
                    n1348 = local read "SELECT LAB01-2"() -> (w2013:T3)
                    n1349 = local read "RUN LAB05-1"() -> (w1975:bool)
                    n1350 = local read "RUN LAB05-2"() -> (w1974:bool)
                    n1351 = local read "RUN LAB04-2"() -> (w1976:bool)
                    n1352 = local read "RUN LAB04-1"() -> (w1977:bool)
                    n1353 = local read "RUN LAB01-1"() -> (w1993:bool)
                    n1354 = local read "RUN LAB01-2"() -> (w1982:bool)
                    n1355 = local read "RUN LAB03-2"() -> (w1978:bool)
                    n1356 = local read "SELECT LAB01-1"() -> (w2017:T3)
                    n1357 = local read "RUN LAB03-1"() -> (w1979:bool)
                    n1358 = local read "RUN LAB02-1"() -> (w1981:bool)
                    n1359 = local read "RUN LAB02-2"() -> (w1980:bool)
                    n1360 = Equal?(x=w2014, y=w2010) -> (x = y?=w1988:bool)
                    n1361 = Equal?(x=w2014, y=w2009) -> (x = y?=w1987:bool)
                    n1362 = Equal?(x=w2014, y=w2008) -> (x = y?=w1986:bool)
                    n1363 = Equal?(x=w2014, y=w2007) -> (x = y?=w1985:bool)
                    n1364 = Equal?(x=w2014, y=w2006) -> (x = y?=w1984:bool)
                    n1365 = Equal?(x=w2014, y=w2005) -> (x = y?=w1983:bool)
                    n1366 = Equal?(x=w2014, y=w2017) -> (x = y?=w1994:bool)
                    n1367 = Equal?(x=w2014, y=w2012) -> (x = y?=w1990:bool)
                    n1368 = Equal?(x=w2014, y=w2011) -> (x = y?=w1989:bool)
                    n1369 = Equal?(x=w2014, y=w2013) -> (x = y?=w1991:bool)
                    n1370 = And(x=w1985, y=w1976) -> (x .and. y?=w1967:bool)
                    n1371 = And(x=w1988, y=w1979) -> (x .and. y?=w1970:bool)
                    n1372 = And(x=w1986, y=w1977) -> (x .and. y?=w1968:bool)
                    n1373 = And(x=w1983, y=w1974) -> (x .and. y?=w1965:bool)
                    n1374 = And(x=w1989, y=w1980) -> (x .and. y?=w1971:bool)
                    n1375 = And(x=w1987, y=w1978) -> (x .and. y?=w1969:bool)
                    n1376 = And(x=w1984, y=w1975) -> (x .and. y?=w1966:bool)
                    n1377 = And(x=w1991, y=w1982) -> (x .and. y?=w1973:bool)
                    n1378 = And(x=w1994, y=w1993) -> (x .and. y?=w1992:bool)
                    n1379 = And(x=w1990, y=w1981) -> (x .and. y?=w1972:bool)
                    n1380 = Select(t=w2016, s=w1992, f=w2015) -> (s? t:f=w1995:bool)
                    n1381 = Select(t=w2016, s=w1973, f=w2015) -> (s? t:f=w1996:bool)
                    n1382 = Select(t=w2016, s=w1972, f=w2015) -> (s? t:f=w1997:bool)
                    n1383 = Select(t=w2016, s=w1971, f=w2015) -> (s? t:f=w1998:bool)
                    n1384 = Select(t=w2016, s=w1970, f=w2015) -> (s? t:f=w1999:bool)
                    n1385 = Select(t=w2016, s=w1969, f=w2015) -> (s? t:f=w2000:bool)
                    n1386 = Select(t=w2016, s=w1968, f=w2015) -> (s? t:f=w2001:bool)
                    n1387 = Select(t=w2016, s=w1967, f=w2015) -> (s? t:f=w2002:bool)
                    n1388 = Select(t=w2016, s=w1966, f=w2015) -> (s? t:f=w2003:bool)
                    n1389 = Select(t=w2016, s=w1965, f=w2015) -> (s? t:f=w2004:bool)
                    n1390 = local write "JIG LAB03-2"(w2000) -> ()
                    n1391 = local write "JIG LAB02-1"(w1997) -> ()
                    n1392 = local write "JIG LAB02-2"(w1998) -> ()
                    n1393 = local write "JIG LAB01-2"(w1996) -> ()
                    n1394 = local write "JIG LAB03-1"(w1999) -> ()
                    n1395 = local write "JIG LAB01-1"(w1995) -> ()
                    n1396 = local write "JIG LAB05-2"(w2004) -> ()
                    n1397 = local write "JIG LAB04-1"(w2001) -> ()
                    n1398 = local write "JIG LAB05-1"(w2003) -> ()
                    n1399 = local write "JIG LAB04-2"(w2002) -> ()
                  }
                }
              }
            }
          }
          frame #9 {
            # "drive digital output"
            n1400 = local read "O/I  LAB05-2"() -> (w2023:bool)
            n1401 = local read "O/I  LAB05-1"() -> (w2025:bool)
            n1402 = local read "JIG LAB05-2"() -> (w2022:bool)
            n1403 = local read "O/I  LAB04-2"() -> (w2027:bool)
            n1404 = local read "JIG LAB05-1"() -> (w2024:bool)
            n1405 = local read "JIG LAB04-2"() -> (w2026:bool)
            n1406 = local read "O/1  LAB02-2"() -> (w2034:bool)
            n1407 = local read "O/I  LAB03-1"() -> (w2032:bool)
            n1408 = local read "O/I  LAB04-1"() -> (w2028:bool)
            n1409 = local read "O/I  LAB02-1"() -> (w2036:bool)
            n1410 = local read "O/I  LAB03-2"() -> (w2030:bool)
            n1411 = local read "JIG LAB04-1"() -> (w2021:bool)
            n1412 = local read "JIG LAB03-2"() -> (w2029:bool)
            n1413 = local read "O/I  LAB01-2"() -> (w2038:bool)
            n1414 = local read "JIG LAB02-1"() -> (w2035:bool)
            n1415 = local read "JIG LAB02-2"() -> (w2033:bool)
            n1416 = local read "JIG LAB03-1"() -> (w2031:bool)
            n1417 = local read "O/I  LAB01-1"() -> (w2040:bool)
            n1418 = local read "JIG LAB01-2"() -> (w2037:bool)
            n1419 = local read "JIG LAB01-1"() -> (w2039:bool)
            n1420 = Build Array(w2027, w2026, w2025, w2024, w2023, w2022) -> (w2018:bool[])
            n1421 = Build Array(w2033, w2032, w2031, w2030, w2029, w2028, w2021) -> (w2019:bool[])
            n1422 = Build Array(w2040, w2039, w2038, w2037, w2036, w2035, w2034) -> (w2020:bool[])
            n1423 = call "sub vi - Drive Relays All v6.vi"("Array #2"=w2018, "Array #1"=w2019, "Array #0"=w2020) -> ()  [unwired: 8 in, 1 out]
          }
          frame #10 {
            # "get temperature values"
            n1424 = stacked-sequence {
              frame #0 {
                n1425 = local read "jig cycle"() -> (w2041:dbl)
                n1426 = local read "on loops"() -> (w2044:dbl)
                n1427 = local read "jig cycle"() -> (w2046:dbl)
                n1428 = Add(x=w2044, y=2) -> (x+y=w2045:dbl)
                n1429 = Equal?(x=w2046, y=0) -> (x = y?=w2047:bool)
                n1430 = Equal?(x=w2041, y=w2045) -> (x = y?=w2042:bool)
                n1431 = case shown="True" w2047 {
                  frame False {
                  }
                  frame True {
                    w2059 = FALSE
                    w2060 = TRUE
                    n1432 = local write "TEMP update"(TRUE) -> ()
                    n1433 = call "sub vi - GET ALL TEMP v3.vi"("LA01-EN"=w2060, "LA02-EN"=w2060, "LA03-EN"=w2060, "LA04-EN"=w2059, "LA05-EN"=w2059, "Gen Cal Value"=1.0) -> ("LA01 TEMP"=w2058:T27, "LA02 TEMP"=w2056:T27, "LA03 TEMP"=w2055:T27)  [unwired: 4 in, 3 out]
                    n1434 = local write "LAB03 TEMP"(w2055) -> ()
                    n1435 = local write "LAB02 TEMP"(w2056) -> ()
                    n1436 = local write "LAB01 TEMP"(w2058) -> ()
                  }
                }
                n1437 = case shown="True" w2042 {
                  frame False {
                  }
                  frame True {
                    w2052 = TRUE
                    w2053 = FALSE
                    n1438 = local write "TEMP update"(TRUE) -> ()
                    n1439 = call "sub vi - GET ALL TEMP v3.vi"("LA01-EN"=w2053, "LA02-EN"=w2053, "LA03-EN"=w2053, "LA04-EN"=w2052, "LA05-EN"=w2052, "Gen Cal Value"=1.0) -> ("LA04 TEMP"=w2050:T27, "LA05 TEMP"=w2049:T27)  [unwired: 4 in, 4 out]
                    n1440 = local write "LAB04 TEMP"(w2050) -> ()
                    n1441 = local write "LAB05 TEMP"(w2049) -> ()
                  }
                }
              }
              frame #1 {
                n1442 = local read "CAL LAB01"() -> (w2078:T7)
                n1443 = local read "LAB01 TEMP"() -> (w2079:T10)
                n1444 = Unbundle By Name(w2079) -> ("T1 Live"=w2069:dbl, "T1 Neut"=w2068:dbl, "T2 Live"=w2067:dbl, "T2 Neut"=w2066:dbl)  [unwired: 2 out]
                n1445 = Unbundle By Name(w2078) -> ("1 (TL) cal"=w2065:dbl, "1 (TN) cal"=w2064:dbl, "2 (TL) cal"=w2063:dbl, "2 (TN) cal"=w2062:dbl)  [unwired: 6 out]
                n1446 = Multiply(x=w2069, y=w2065) -> (x*y=w2075:dbl)
                n1447 = Multiply(x=w2068, y=w2064) -> (x*y=w2074:dbl)
                n1448 = Multiply(x=w2067, y=w2063) -> (x*y=w2071:dbl)
                n1449 = Multiply(x=w2066, y=w2062) -> (x*y=w2070:dbl)
                n1450 = local read "SIG LAB01-2"() -> (w2073:T2)
                n1451 = local read "SIG LAB01-1"() -> (w2077:T2)
                n1452 = Bundle By Name(cluster=w2077, "Tmp Live"=w2075, "Tmp Neut"=w2074) -> (w2076:T2)
                n1453 = Bundle By Name(cluster=w2073, "Tmp Live"=w2071, "Tmp Neut"=w2070) -> (w2072:T2)
                n1454 = local write "SIG LAB01-1"(w2076) -> ()
                n1455 = local write "SIG LAB01-2"(w2072) -> ()
              }
              frame #2 {
                n1456 = local read "CAL LAB02"() -> (w2096:T8)
                n1457 = local read "LAB02 TEMP"() -> (w2097:T10)
                n1458 = Unbundle By Name(w2097) -> ("T1 Live"=w2087:dbl, "T1 Neut"=w2086:dbl, "T2 Live"=w2085:dbl, "T2 Neut"=w2084:dbl)  [unwired: 2 out]
                n1459 = Unbundle By Name(w2096) -> ("1 (TL) cal"=w2083:dbl, "1 (TN) cal"=w2082:dbl, "2 (TL) cal"=w2081:dbl, "2 (TN) cal"=w2080:dbl)  [unwired: 6 out]
                n1460 = Multiply(x=w2087, y=w2083) -> (x*y=w2093:dbl)
                n1461 = Multiply(x=w2086, y=w2082) -> (x*y=w2092:dbl)
                n1462 = Multiply(x=w2085, y=w2081) -> (x*y=w2089:dbl)
                n1463 = Multiply(x=w2084, y=w2080) -> (x*y=w2088:dbl)
                n1464 = local read "SIG LAB02-2"() -> (w2091:T2)
                n1465 = local read "SIG LAB02-1"() -> (w2095:T2)
                n1466 = Bundle By Name(cluster=w2095, "Tmp Live"=w2093, "Tmp Neut"=w2092) -> (w2094:T2)
                n1467 = Bundle By Name(cluster=w2091, "Tmp Live"=w2089, "Tmp Neut"=w2088) -> (w2090:T2)
                n1468 = local write "SIG LAB02-1"(w2094) -> ()
                n1469 = local write "SIG LAB02-2"(w2090) -> ()
              }
              frame #3 {
                n1470 = local read "CAL LAB03"() -> (w2114:T7)
                n1471 = local read "LAB03 TEMP"() -> (w2115:T10)
                n1472 = Unbundle By Name(w2115) -> ("T1 Live"=w2105:dbl, "T1 Neut"=w2104:dbl, "T2 Live"=w2103:dbl, "T2 Neut"=w2102:dbl)  [unwired: 2 out]
                n1473 = Unbundle By Name(w2114) -> ("1 (TL) cal"=w2101:dbl, "1 (TN) cal"=w2100:dbl, "2 (TL) cal"=w2099:dbl, "2 (TN) cal"=w2098:dbl)  [unwired: 6 out]
                n1474 = Multiply(x=w2105, y=w2101) -> (x*y=w2111:dbl)
                n1475 = Multiply(x=w2104, y=w2100) -> (x*y=w2110:dbl)
                n1476 = Multiply(x=w2103, y=w2099) -> (x*y=w2107:dbl)
                n1477 = Multiply(x=w2102, y=w2098) -> (x*y=w2106:dbl)
                n1478 = local read "SIG LAB03-2"() -> (w2109:T2)
                n1479 = local read "SIG LAB03-1"() -> (w2113:T2)
                n1480 = Bundle By Name(cluster=w2113, "Tmp Live"=w2111, "Tmp Neut"=w2110) -> (w2112:T2)
                n1481 = Bundle By Name(cluster=w2109, "Tmp Live"=w2107, "Tmp Neut"=w2106) -> (w2108:T2)
                n1482 = local write "SIG LAB03-1"(w2112) -> ()
                n1483 = local write "SIG LAB03-2"(w2108) -> ()
              }
              frame #4 {
                n1484 = local read "CAL LAB04"() -> (w2132:T7)
                n1485 = local read "LAB04 TEMP"() -> (w2133:T10)
                n1486 = Unbundle By Name(w2133) -> ("T1 Live"=w2123:dbl, "T1 Neut"=w2122:dbl, "T2 Live"=w2121:dbl, "T2 Neut"=w2120:dbl)  [unwired: 2 out]
                n1487 = Unbundle By Name(w2132) -> ("1 (TL) cal"=w2119:dbl, "1 (TN) cal"=w2118:dbl, "2 (TL) cal"=w2117:dbl, "2 (TN) cal"=w2116:dbl)  [unwired: 6 out]
                n1488 = Multiply(x=w2123, y=w2119) -> (x*y=w2129:dbl)
                n1489 = Multiply(x=w2122, y=w2118) -> (x*y=w2128:dbl)
                n1490 = Multiply(x=w2121, y=w2117) -> (x*y=w2125:dbl)
                n1491 = Multiply(x=w2120, y=w2116) -> (x*y=w2124:dbl)
                n1492 = local read "SIG LAB04-2"() -> (w2127:T2)
                n1493 = local read "SIG LAB04-1"() -> (w2131:T2)
                n1494 = Bundle By Name(cluster=w2131, "Tmp Live"=w2129, "Tmp Neut"=w2128) -> (w2130:T2)
                n1495 = Bundle By Name(cluster=w2127, "Tmp Live"=w2125, "Tmp Neut"=w2124) -> (w2126:T2)
                n1496 = local write "SIG LAB04-1"(w2130) -> ()
                n1497 = local write "SIG LAB04-2"(w2126) -> ()
              }
              frame #5 {
                n1498 = local read "CAL LAB05"() -> (w2150:T7)
                n1499 = local read "LAB05 TEMP"() -> (w2151:T10)
                n1500 = Unbundle By Name(w2151) -> ("T1 Live"=w2141:dbl, "T1 Neut"=w2140:dbl, "T2 Live"=w2139:dbl, "T2 Neut"=w2138:dbl)  [unwired: 2 out]
                n1501 = Unbundle By Name(w2150) -> ("1 (TL) cal"=w2137:dbl, "1 (TN) cal"=w2136:dbl, "2 (TL) cal"=w2135:dbl, "2 (TN) cal"=w2134:dbl)  [unwired: 6 out]
                n1502 = Multiply(x=w2141, y=w2137) -> (x*y=w2147:dbl)
                n1503 = Multiply(x=w2140, y=w2136) -> (x*y=w2146:dbl)
                n1504 = Multiply(x=w2139, y=w2135) -> (x*y=w2143:dbl)
                n1505 = Multiply(x=w2138, y=w2134) -> (x*y=w2142:dbl)
                n1506 = local read "SIG LAB05-2"() -> (w2145:T2)
                n1507 = local read "SIG LAB05-1"() -> (w2149:T2)
                n1508 = Bundle By Name(cluster=w2149, "Tmp Live"=w2147, "Tmp Neut"=w2146) -> (w2148:T2)
                n1509 = Bundle By Name(cluster=w2145, "Tmp Live"=w2143, "Tmp Neut"=w2142) -> (w2144:T2)
                n1510 = local write "SIG LAB05-1"(w2148) -> ()
                n1511 = local write "SIG LAB05-2"(w2144) -> ()
              }
            }
          }
          frame #11 {
            # "get analog values"
            n1512 = local read "on loops"() -> (w2158:dbl)
            n1513 = local read "jig cycle"() -> (w2155:dbl)
            n1514 = Add(x=w2158, y=1) -> (x+y=w2156:dbl)
            n1515 = Equal?(x=w2155, y=1) -> (x = y?=w2153:bool)
            n1516 = Equal?(x=w2155, y=w2156) -> (x = y?=w2154:bool)
            n1517 = Or(x=w2153, y=w2154) -> (x .or. y?=w2152:bool)
            n1518 = case shown="True" w2152 {
              frame False {
              }
              frame True {
                n1519 = call "sub vi - Read Analog All v8.vi"() -> ("Analog loop time"=w2166:dbl, "array GRAPH"=w2165:dynamicdata[], "LAB01"=w2164:T28, "LAB02"=w2163:T29, "LAB03"=w2162:T30, "LAB04"=w2161:T31, "array ERROR"=w2167:errorcluster[], "LAB05"=w2160:T32)  [unwired: 8 in]
                n1520 = stacked-sequence {
                  tunnel: w2167 -> [w2170 _ _ _ _ _]
                  tunnel: w2166 -> [w2169 _ _ _ _ _]
                  tunnel: w2165 -> [w2168 _ _ _ _ _]
                  tunnel: w2164 -> [_ w2215 _ _ _ _]
                  tunnel: w2163 -> [_ _ w2216 _ _ _]
                  tunnel: w2162 -> [_ _ _ w2241 _ _]
                  tunnel: w2161 -> [_ _ _ _ w2264 _]
                  tunnel: w2160 -> [_ _ _ _ _ w2289]
                  frame #0 {
                    n1521 = local write "AI update"(TRUE) -> ()
                    n1522 = Index Array(array=w2168, index=6) -> (element=→"LAB04-1 (GRAPH)":dynamicdata)
                    n1523 = Index Array(array=w2168, index=7) -> (element=→"LAB04-2 (GRAPH)":dynamicdata)
                    n1524 = Index Array(array=w2168, index=9) -> (element=→"LAB05-2 (GRAPH)":dynamicdata)
                    n1525 = Index Array(array=w2168, index=8) -> (element=→"LAB05-1 (GRAPH)":dynamicdata)
                    n1526 = Index Array(array=w2168, index=5) -> (element=→"LAB03-2 (GRAPH)":dynamicdata)
                    n1527 = Index Array(array=w2168, index=0) -> (element=→"LAB01-1 (GRAPH)":dynamicdata)
                    n1528 = Index Array(array=w2168, index=1) -> (element=→"LAB01-2 (GRAPH)":dynamicdata)
                    n1529 = Index Array(array=w2168, index=2) -> (element=→"LAB02-1 (GRAPH)":dynamicdata)
                    n1530 = Index Array(array=w2168, index=3) -> (element=→"LAB02-2 (GRAPH)":dynamicdata)
                    n1531 = Index Array(array=w2168, index=4) -> (element=→"LAB03-1 (GRAPH)":dynamicdata)
                    "AI loop time" <- w2169
                    "Analog Error Array" <- w2170
                  }
                  frame #1 {
                    n1532 = local read "CAL LAB01"() -> (w2214:T7)
                    n1533 = Unbundle By Name(w2215) -> ("LAB01-1 (A)"=w2213:dbl, "LAB01-1 (V)"=w2212:dbl, "LAB01-1 (PF)"=w2211:dbl, "LAB01-2 (A)"=w2210:dbl, "LAB01-2 (V)"=w2209:dbl, "LAB01-2 (PF)"=w2208:dbl)
                    n1534 = Unbundle By Name(w2214) -> ("1  (A) cal"=w2207:dbl, "1 (V) cal"=w2206:dbl, "1 (PF) cal"=w2205:dbl, "2 (A) cal"=w2204:dbl, "2 (V) cal"=w2203:dbl, "2 (PF) cal"=w2202:dbl)  [unwired: 4 out]
                    n1535 = Multiply(x=w2213, y=w2207) -> (x*y=w2200:dbl)
                    n1536 = Multiply(x=w2212, y=w2206) -> (x*y=w2199:dbl)
                    n1537 = Multiply(x=w2211, y=w2205) -> (x*y=w2198:dbl)
                    n1538 = Multiply(x=w2210, y=w2204) -> (x*y=w2194:dbl)
                    n1539 = Multiply(x=w2209, y=w2203) -> (x*y=w2193:dbl)
                    n1540 = Multiply(x=w2208, y=w2202) -> (x*y=w2192:dbl)
                    n1541 = local read "SIG LAB01-1"() -> (w2201:T2)
                    n1542 = local read "SIG LAB01-2"() -> (w2196:T2)
                    n1543 = Bundle By Name(cluster=w2201, "AMPS"=w2200, "VOLTS"=w2199, "PF"=w2198) -> (w2197:T2)
                    n1544 = Bundle By Name(cluster=w2196, "AMPS"=w2194, "VOLTS"=w2193, "PF"=w2192) -> (w2195:T2)
                    n1545 = local write "SIG LAB01-2"(w2195) -> ()
                    n1546 = local write "SIG LAB01-1"(w2197) -> ()
                  }
                  frame #2 {
                    n1547 = local read "CAL LAB02"() -> (w2239:T8)
                    n1548 = Unbundle By Name(w2216) -> ("LAB02-1 (A)"=w2238:dbl, "LAB02-1 (V)"=w2237:dbl, "LAB02-1 (PF)"=w2236:dbl, "LAB02-2 (A)"=w2235:dbl, "LAB02-2 (V)"=w2234:dbl, "LAB02-2 (PF)"=w2233:dbl)
                    n1549 = Unbundle By Name(w2239) -> ("1 (A) cal"=w2232:dbl, "1 (V) cal"=w2231:dbl, "1 (PF) cal"=w2230:dbl, "2 (A) cal"=w2229:dbl, "2 (V) cal"=w2228:dbl, "2 (PF) cal"=w2227:dbl)  [unwired: 4 out]
                    n1550 = Multiply(x=w2238, y=w2232) -> (x*y=w2225:dbl)
                    n1551 = Multiply(x=w2237, y=w2231) -> (x*y=w2224:dbl)
                    n1552 = Multiply(x=w2236, y=w2230) -> (x*y=w2223:dbl)
                    n1553 = Multiply(x=w2235, y=w2229) -> (x*y=w2219:dbl)
                    n1554 = Multiply(x=w2234, y=w2228) -> (x*y=w2218:dbl)
                    n1555 = Multiply(x=w2233, y=w2227) -> (x*y=w2217:dbl)
                    n1556 = local read "SIG LAB02-1"() -> (w2226:T2)
                    n1557 = local read "SIG LAB02-2"() -> (w2221:T2)
                    n1558 = Bundle By Name(cluster=w2226, "AMPS"=w2225, "VOLTS"=w2224, "PF"=w2223) -> (w2222:T2)
                    n1559 = Bundle By Name(cluster=w2221, "AMPS"=w2219, "VOLTS"=w2218, "PF"=w2217) -> (w2220:T2)
                    n1560 = local write "SIG LAB02-2"(w2220) -> ()
                    n1561 = local write "SIG LAB02-1"(w2222) -> ()
                  }
                  frame #3 {
                    n1562 = local read "CAL LAB03"() -> (w2263:T7)
                    n1563 = Unbundle By Name(w2241) -> ("LAB03-1 (A)"=w2262:dbl, "LAB03-1 (V)"=w2261:dbl, "LAB03-1 (PF)"=w2260:dbl, "LAB03-2 (A)"=w2259:dbl, "LAB03-2 (V)"=w2258:dbl, "LAB03-2 (PF)"=w2257:dbl)
                    n1564 = Unbundle By Name(w2263) -> ("1  (A) cal"=w2256:dbl, "1 (V) cal"=w2255:dbl, "1 (PF) cal"=w2254:dbl, "2 (A) cal"=w2253:dbl, "2 (V) cal"=w2252:dbl, "2 (PF) cal"=w2251:dbl)  [unwired: 4 out]
                    n1565 = Multiply(x=w2262, y=w2256) -> (x*y=w2249:dbl)
                    n1566 = Multiply(x=w2261, y=w2255) -> (x*y=w2240:dbl)
                    n1567 = Multiply(x=w2260, y=w2254) -> (x*y=w2248:dbl)
                    n1568 = Multiply(x=w2259, y=w2253) -> (x*y=w2244:dbl)
                    n1569 = Multiply(x=w2258, y=w2252) -> (x*y=w2243:dbl)
                    n1570 = Multiply(x=w2257, y=w2251) -> (x*y=w2242:dbl)
                    n1571 = local read "SIG LAB03-1"() -> (w2250:T2)
                    n1572 = local read "SIG LAB03-2"() -> (w2246:T2)
                    n1573 = Bundle By Name(cluster=w2250, "AMPS"=w2249, "VOLTS"=w2240, "PF"=w2248) -> (w2247:T2)
                    n1574 = Bundle By Name(cluster=w2246, "AMPS"=w2244, "VOLTS"=w2243, "PF"=w2242) -> (w2245:T2)
                    n1575 = local write "SIG LAB03-2"(w2245) -> ()
                    n1576 = local write "SIG LAB03-1"(w2247) -> ()
                  }
                  frame #4 {
                    n1577 = local read "CAL LAB04"() -> (w2287:T7)
                    n1578 = Unbundle By Name(w2264) -> ("LAB04-1 (A)"=w2286:dbl, "LAB04-1 (V)"=w2285:dbl, "LAB04-1 (PF)"=w2284:dbl, "LAB04-2 (A)"=w2283:dbl, "LAB04-2 (V)"=w2282:dbl, "LAB04-2 (PF)"=w2281:dbl)
                    n1579 = Unbundle By Name(w2287) -> ("1  (A) cal"=w2280:dbl, "1 (V) cal"=w2279:dbl, "1 (PF) cal"=w2278:dbl, "2 (A) cal"=w2277:dbl, "2 (V) cal"=w2276:dbl, "2 (PF) cal"=w2275:dbl)  [unwired: 4 out]
                    n1580 = Multiply(x=w2286, y=w2280) -> (x*y=w2273:dbl)
                    n1581 = Multiply(x=w2285, y=w2279) -> (x*y=w2272:dbl)
                    n1582 = Multiply(x=w2284, y=w2278) -> (x*y=w2271:dbl)
                    n1583 = Multiply(x=w2283, y=w2277) -> (x*y=w2267:dbl)
                    n1584 = Multiply(x=w2282, y=w2276) -> (x*y=w2266:dbl)
                    n1585 = Multiply(x=w2281, y=w2275) -> (x*y=w2265:dbl)
                    n1586 = local read "SIG LAB04-1"() -> (w2274:T2)
                    n1587 = local read "SIG LAB04-2"() -> (w2269:T2)
                    n1588 = Bundle By Name(cluster=w2274, "AMPS"=w2273, "VOLTS"=w2272, "PF"=w2271) -> (w2270:T2)
                    n1589 = Bundle By Name(cluster=w2269, "AMPS"=w2267, "VOLTS"=w2266, "PF"=w2265) -> (w2268:T2)
                    n1590 = local write "SIG LAB04-2"(w2268) -> ()
                    n1591 = local write "SIG LAB04-1"(w2270) -> ()
                  }
                  frame #5 {
                    n1592 = local read "CAL LAB05"() -> (w2311:T7)
                    n1593 = Unbundle By Name(w2289) -> ("LAB05-1 (A)"=w2310:dbl, "LAB05-1 (V)"=w2288:dbl, "LAB05-1 (PF)"=w2309:dbl, "LAB05-2 (A)"=w2308:dbl, "LAB05-2 (V)"=w2307:dbl, "LAB05-2 (PF)"=w2306:dbl)
                    n1594 = Unbundle By Name(w2311) -> ("1  (A) cal"=w2305:dbl, "1 (V) cal"=w2304:dbl, "1 (PF) cal"=w2303:dbl, "2 (A) cal"=w2302:dbl, "2 (V) cal"=w2301:dbl, "2 (PF) cal"=w2300:dbl)  [unwired: 4 out]
                    n1595 = Multiply(x=w2310, y=w2305) -> (x*y=w2298:dbl)
                    n1596 = Multiply(x=w2288, y=w2304) -> (x*y=w2297:dbl)
                    n1597 = Multiply(x=w2309, y=w2303) -> (x*y=w2296:dbl)
                    n1598 = Multiply(x=w2308, y=w2302) -> (x*y=w2292:dbl)
                    n1599 = Multiply(x=w2307, y=w2301) -> (x*y=w2291:dbl)
                    n1600 = Multiply(x=w2306, y=w2300) -> (x*y=w2290:dbl)
                    n1601 = local read "SIG LAB05-1"() -> (w2299:T2)
                    n1602 = local read "SIG LAB05-2"() -> (w2294:T2)
                    n1603 = Bundle By Name(cluster=w2299, "AMPS"=w2298, "VOLTS"=w2297, "PF"=w2296) -> (w2295:T2)
                    n1604 = Bundle By Name(cluster=w2294, "AMPS"=w2292, "VOLTS"=w2291, "PF"=w2290) -> (w2293:T2)
                    n1605 = local write "SIG LAB05-2"(w2293) -> ()
                    n1606 = local write "SIG LAB05-1"(w2295) -> ()
                  }
                }
              }
            }
          }
          frame #12 {
            # "save test data to file"
            n1607 = local read "on loops"() -> (w2328:dbl)
            n1608 = local read "jig cycle"() -> (w2325:dbl)
            n1609 = Add(x=w2328, y=2) -> (x+y=w2326:dbl)
            n1610 = Equal?(x=w2325, y=1) -> (x = y?=w2323:bool)
            n1611 = Equal?(x=w2325, y=w2326) -> (x = y?=w2324:bool)
            n1612 = Or(x=w2323, y=w2324) -> (x .or. y?=w2322:bool)
            n1613 = case shown="True" w2322 {
              tunnel: w2321 -> [_ w2339]
              tunnel: w2320 -> [_ w2338]
              tunnel: w2319 -> [_ w2337]
              tunnel: w2318 -> [_ w2336]
              tunnel: w2317 -> [_ w2335]
              tunnel: w2316 -> [_ w2334]
              tunnel: w2315 -> [_ w2333]
              tunnel: w2314 -> [_ w2332]
              tunnel: w2313 -> [_ w2331]
              tunnel: w2312 -> [_ w2330]
              frame False {
              }
              frame True {
                n1614 = stacked-sequence {
                  tunnel: w2339 -> [w2340 _ _ _ _ _ _ _ _ _]
                  tunnel: w2338 -> [_ w2347 _ _ _ _ _ _ _ _]
                  tunnel: w2337 -> [_ _ w2354 _ _ _ _ _ _ _]
                  tunnel: w2336 -> [_ _ _ w2361 _ _ _ _ _ _]
                  tunnel: w2335 -> [_ _ _ _ w2368 _ _ _ _ _]
                  tunnel: w2334 -> [_ _ _ _ _ w2375 _ _ _ _]
                  tunnel: w2333 -> [_ _ _ _ _ _ w2382 _ _ _]
                  tunnel: w2332 -> [_ _ _ _ _ _ _ w2389 _ _]
                  tunnel: w2331 -> [_ _ _ _ _ _ _ _ w2396 _]
                  tunnel: w2330 -> [_ _ _ _ _ _ _ _ _ w2403]
                  frame #0 {
                    # "LAB01-1"
                    n1615 = case shown="True" w2340 {
                      frame False {
                      }
                      frame True {
                        n1616 = local read "DISP LAB01-1"() -> (w2344:T4)
                        n1617 = local read "SIG LAB01-1"() -> (w2345:T2)
                        n1618 = local read "SET LAB01-1"() -> (w2346:T5)
                        n1619 = Bundle("SET LAB01-1"=w2346, "SIG LAB01-1"=w2345, "DISP LAB01-1"=w2344) -> (w2343:T18)  [unwired: 1 in]
                        n1620 = local read "DATA LAB01-1"() -> (w2342:refnum<k1>)
                        n1621 = Write Datalog(6:w2343, 7:w2342) -> (0:w2341:errorcluster)  [unwired: 1 in, 1 out]
                        n1622 = local write "data file error"(w2341) -> ()
                      }
                    }
                  }
                  frame #1 {
                    # "LAB01-2"
                    n1623 = case shown="True" w2347 {
                      frame False {
                      }
                      frame True {
                        n1624 = local read "SET LAB01-2"() -> (w2353:T5)
                        n1625 = local read "DISP LAB01-2"() -> (w2351:T4)
                        n1626 = local read "SIG LAB01-2"() -> (w2352:T2)
                        n1627 = local read "DATA LAB01-2"() -> (w2350:refnum<k1>)
                        n1628 = Bundle("SET LAB01-2"=w2353, "SIG LAB01-2"=w2352, "DISP LAB01-2"=w2351) -> (w2349:T33)  [unwired: 1 in]
                        n1629 = Write Datalog(6:w2349, 7:w2350) -> (0:w2348:errorcluster)  [unwired: 1 in, 1 out]
                        n1630 = local write "data file error"(w2348) -> ()
                      }
                    }
                  }
                  frame #2 {
                    # "LAB02-1"
                    n1631 = case shown="True" w2354 {
                      frame False {
                      }
                      frame True {
                        n1632 = local read "DISP LAB02-1"() -> (w2359:T4)
                        n1633 = local read "SIG LAB02-1"() -> (w2358:T2)
                        n1634 = local read "SET LAB02-1"() -> (w2360:T5)
                        n1635 = local read "DATA LAB02-1"() -> (w2357:refnum<k1>)
                        n1636 = Bundle("SET LAB02-1"=w2360, "SIG LAB02-1"=w2358, "DISP LAB02-1"=w2359) -> (w2356:T19)  [unwired: 1 in]
                        n1637 = Write Datalog(6:w2356, 7:w2357) -> (0:w2355:errorcluster)  [unwired: 1 in, 1 out]
                        n1638 = local write "data file error"(w2355) -> ()
                      }
                    }
                  }
                  frame #3 {
                    # "LAB02-2"
                    n1639 = case shown="True" w2361 {
                      frame False {
                      }
                      frame True {
                        n1640 = local read "DISP LAB02-2"() -> (w2365:T4)
                        n1641 = local read "SIG LAB02-2"() -> (w2366:T2)
                        n1642 = local read "SET LAB02-2"() -> (w2367:T5)
                        n1643 = local read "DATA LAB02-2"() -> (w2363:refnum<k1>)
                        n1644 = Bundle("SET LAB02-2"=w2367, "SIG LAB02-2"=w2366, "DISP LAB02-2"=w2365) -> (w2364:T20)  [unwired: 1 in]
                        n1645 = Write Datalog(6:w2364, 7:w2363) -> (0:w2362:errorcluster)  [unwired: 1 in, 1 out]
                        n1646 = local write "data file error"(w2362) -> ()
                      }
                    }
                  }
                  frame #4 {
                    # "LAB03-1"
                    n1647 = case shown="True" w2368 {
                      frame False {
                      }
                      frame True {
                        n1648 = local read "DISP LAB03-1"() -> (w2372:T4)
                        n1649 = local read "SIG LAB03-1"() -> (w2373:T2)
                        n1650 = local read "SET LAB03-1"() -> (w2374:T5)
                        n1651 = local read "DATA LAB03-1"() -> (w2370:refnum<k1>)
                        n1652 = Bundle("SET LAB03-1"=w2374, "SIG LAB03-1"=w2373, "DISP LAB03-1"=w2372) -> (w2371:T21)  [unwired: 1 in]
                        n1653 = Write Datalog(6:w2371, 7:w2370) -> (0:w2369:errorcluster)  [unwired: 1 in, 1 out]
                        n1654 = local write "data file error"(w2369) -> ()
                      }
                    }
                  }
                  frame #5 {
                    # "LAB03-2"
                    n1655 = case shown="True" w2375 {
                      frame False {
                      }
                      frame True {
                        n1656 = local read "DISP LAB03-2"() -> (w2379:T4)
                        n1657 = local read "SIG LAB03-2"() -> (w2380:T2)
                        n1658 = local read "SET LAB03-2"() -> (w2381:T5)
                        n1659 = local read "DATA LAB03-2"() -> (w2377:refnum<k1>)
                        n1660 = Bundle("SET LAB03-2"=w2381, "SIG LAB03-2"=w2380, "DISP LAB03-2"=w2379) -> (w2378:T22)  [unwired: 1 in]
                        n1661 = Write Datalog(6:w2378, 7:w2377) -> (0:w2376:errorcluster)  [unwired: 1 in, 1 out]
                        n1662 = local write "data file error"(w2376) -> ()
                      }
                    }
                  }
                  frame #6 {
                    # "LAB04-1"
                    n1663 = case shown="True" w2382 {
                      frame False {
                      }
                      frame True {
                        n1664 = local read "DISP LAB04-1"() -> (w2386:T4)
                        n1665 = local read "SIG LAB04-1"() -> (w2387:T2)
                        n1666 = local read "SET LAB04-1"() -> (w2388:T5)
                        n1667 = local read "DATA LAB04-1"() -> (w2384:refnum<k1>)
                        n1668 = Bundle("SET LAB04-1"=w2388, "SIG LAB04-1"=w2387, "DISP LAB04-1"=w2386) -> (w2385:T23)  [unwired: 1 in]
                        n1669 = Write Datalog(6:w2385, 7:w2384) -> (0:w2383:errorcluster)  [unwired: 1 in, 1 out]
                        n1670 = local write "data file error"(w2383) -> ()
                      }
                    }
                  }
                  frame #7 {
                    # "LAB04-2"
                    n1671 = case shown="True" w2389 {
                      frame False {
                      }
                      frame True {
                        n1672 = local read "DISP LAB04-2"() -> (w2393:T4)
                        n1673 = local read "SIG LAB04-2"() -> (w2394:T2)
                        n1674 = local read "SET LAB04-2"() -> (w2395:T5)
                        n1675 = local read "DATA LAB04-2"() -> (w2391:refnum<k1>)
                        n1676 = Bundle("SET LAB04-2"=w2395, "SIG LAB04-2"=w2394, "DISP LAB04-2"=w2393) -> (w2392:T24)  [unwired: 1 in]
                        n1677 = Write Datalog(6:w2392, 7:w2391) -> (0:w2390:errorcluster)  [unwired: 1 in, 1 out]
                        n1678 = local write "data file error"(w2390) -> ()
                      }
                    }
                  }
                  frame #8 {
                    # "LAB05-1"
                    n1679 = case shown="True" w2396 {
                      frame False {
                      }
                      frame True {
                        n1680 = local read "DISP LAB05-1"() -> (w2400:T4)
                        n1681 = local read "SIG LAB05-1"() -> (w2401:T2)
                        n1682 = local read "SET LAB05-1"() -> (w2402:T5)
                        n1683 = local read "DATA LAB05-1"() -> (w2398:refnum<k1>)
                        n1684 = Bundle("SET LAB05-1"=w2402, "SIG LAB05-1"=w2401, "DISP LAB05-1"=w2400) -> (w2399:T25)  [unwired: 1 in]
                        n1685 = Write Datalog(6:w2399, 7:w2398) -> (0:w2397:errorcluster)  [unwired: 1 in, 1 out]
                        n1686 = local write "data file error"(w2397) -> ()
                      }
                    }
                  }
                  frame #9 {
                    # "LAB05-2"
                    n1687 = case shown="True" w2403 {
                      frame False {
                      }
                      frame True {
                        n1688 = local read "DISP LAB05-2"() -> (w2407:T4)
                        n1689 = local read "SIG LAB05-2"() -> (w2408:T2)
                        n1690 = local read "SET LAB05-2"() -> (w2409:T5)
                        n1691 = local read "DATA LAB05-2"() -> (w2405:refnum<k1>)
                        n1692 = Bundle("SET LAB05-2"=w2409, "SIG LAB05-2"=w2408, "DISP LAB05-2"=w2407) -> (w2406:T26)  [unwired: 1 in]
                        n1693 = Write Datalog(6:w2406, 7:w2405) -> (0:w2404:errorcluster)  [unwired: 1 in, 1 out]
                        n1694 = local write "data file error"(w2404) -> ()
                      }
                    }
                  }
                }
              }
            }
          }
          frame #13 {
            # "check for amps fail"
            # "check for cycle test & temperature rise fail conditions"
            n1695 = local read "on loops"() -> (w2435:dbl)
            n1696 = local read "jig cycle"() -> (w2432:dbl)
            n1697 = local read "jig cycle"() -> (w2437:dbl)
            n1698 = Add(x=w2435, y=3.0) -> (x+y=w2433:dbl)
            n1699 = Equal?(x=w2432, y=w2433) -> (x = y?=w2428:bool)
            n1700 = Equal?(x=w2437, y=1.0) -> (x = y?=w2430:bool)
            n1701 = stacked-sequence {
              tunnel: w2431 -> [w2440 _ _ _ _ _ _ _ _ _]
              tunnel: w2430 -> [w2441 w2461 w2481 w2501 w2521 w2541 w2561 w2581 w2601 w2621]
              tunnel: w2429 -> [w2438 _ _ _ _ _ _ _ _ _]
              tunnel: w2428 -> [w2439 w2460 w2480 w2500 w2520 w2540 w2560 w2580 w2600 w2620]
              tunnel: w2427 -> [_ w2459 _ _ _ _ _ _ _ _]
              tunnel: w2426 -> [_ w2458 _ _ _ _ _ _ _ _]
              tunnel: w2425 -> [_ _ w2479 _ _ _ _ _ _ _]
              tunnel: w2424 -> [_ _ w2478 _ _ _ _ _ _ _]
              tunnel: w2423 -> [_ _ _ w2499 _ _ _ _ _ _]
              tunnel: w2422 -> [_ _ _ w2498 _ _ _ _ _ _]
              tunnel: w2421 -> [_ _ _ _ w2519 _ _ _ _ _]
              tunnel: w2420 -> [_ _ _ _ w2518 _ _ _ _ _]
              tunnel: w2419 -> [_ _ _ _ _ w2539 _ _ _ _]
              tunnel: w2418 -> [_ _ _ _ _ w2538 _ _ _ _]
              tunnel: w2417 -> [_ _ _ _ _ _ w2559 _ _ _]
              tunnel: w2416 -> [_ _ _ _ _ _ w2558 _ _ _]
              tunnel: w2415 -> [_ _ _ _ _ _ _ w2579 _ _]
              tunnel: w2414 -> [_ _ _ _ _ _ _ w2578 _ _]
              tunnel: w2413 -> [_ _ _ _ _ _ _ _ w2599 _]
              tunnel: w2412 -> [_ _ _ _ _ _ _ _ w2598 _]
              tunnel: w2411 -> [_ _ _ _ _ _ _ _ _ w2619]
              tunnel: w2410 -> [_ _ _ _ _ _ _ _ _ w2618]
              frame #0 {
                # "LAB01-1"
                n1702 = case shown="True" w2438 {
                  tunnel: w2441 -> [_ w2454]
                  tunnel: w2440 -> [_ w2451]
                  tunnel: w2439 -> [_ w2450]
                  frame False {
                  }
                  frame True {
                    n1703 = local read "TEMP START LAB01-1"() -> (w2456:cluster{"TL":dbl, "TN":dbl})
                    n1704 = local read "RESULT LAB01-1"() -> (w2444:bool)
                    n1705 = local read "FAIL LAB01-1"() -> (w2447:cluster{"LO":dbl, "HI":dbl})
                    n1706 = local read "DATA LAB01-1"() -> (w2455:refnum<k1>)
                    n1707 = local read "SET LAB01-1"() -> (w2452:T5)
                    n1708 = local read "DISP LAB01-1"() -> (w2453:T4)
                    n1709 = local read "SIG LAB01-1"() -> (w2457:T2)
                    n1710 = Bundle("FAIL LAB01-1"=w2447, "SIG LAB01-1"=w2457, "TEMP START LAB01-1"=w2456, "DISP LAB01-1"=w2453, "SET LAB01-1"=w2452, "DATA LAB01-1"=w2455) -> (w2442:T34)  [unwired: 1 in]
                    n1711 = call "sub vi - cycle&temp fail v5.vi"("Amps Lo?"=w2454, "Input Cluster"=w2442, "SELECT"=w2451, "Amps Hi?"=w2450, "Result In"=w2444) -> ("(FAIL) out"=w2446:cluster{"FAIL LO":dbl, "FAIL HI":dbl}, "(DISP) out"=w2449:T4, "T-RISE"=w2443:cluster{"T-RISE (L)":dbl, "T-RISE (N)":dbl}, "Result Out"=w2445:bool, "file error"=w2448:errorcluster)  [unwired: 10 in]
                    n1712 = local write "TEMP RISE LAB01-1"(w2443) -> ()
                    n1713 = local write "FAIL LAB01-1"(w2446) -> ()
                    n1714 = local write "DISP LAB01-1"(w2449) -> ()
                    n1715 = local write "RESULT LAB01-1"(w2445) -> ()
                    n1716 = local write "data file error"(w2448) -> ()
                  }
                }
              }
              frame #1 {
                # "LAB01-2"
                n1717 = case shown="True" w2459 {
                  tunnel: w2461 -> [_ w2474]
                  tunnel: w2458 -> [_ w2471]
                  tunnel: w2460 -> [_ w2470]
                  frame False {
                  }
                  frame True {
                    n1718 = local read "TEMP START LAB01-2"() -> (w2476:cluster{"TL":dbl, "TN":dbl})
                    n1719 = local read "FAIL LAB01-2"() -> (w2467:cluster{"LO":dbl, "HI":dbl})
                    n1720 = local read "DATA LAB01-2"() -> (w2475:refnum<k1>)
                    n1721 = local read "SET LAB01-2"() -> (w2472:T5)
                    n1722 = local read "DISP LAB01-2"() -> (w2473:T4)
                    n1723 = local read "RESULT LAB01-2"() -> (w2464:bool)
                    n1724 = local read "SIG LAB01-2"() -> (w2477:T2)
                    n1725 = Bundle("FAIL LAB01-2"=w2467, "SIG LAB01-2"=w2477, "TEMP START LAB01-2"=w2476, "DISP LAB01-2"=w2473, "SET LAB01-2"=w2472, "DATA LAB01-2"=w2475) -> (w2462:T35)  [unwired: 1 in]
                    n1726 = call "sub vi - cycle&temp fail v5.vi"("Amps Lo?"=w2474, "Input Cluster"=w2462, "SELECT"=w2471, "Amps Hi?"=w2470, "Result In"=w2464) -> ("(FAIL) out"=w2466:cluster{"FAIL LO":dbl, "FAIL HI":dbl}, "(DISP) out"=w2469:T4, "T-RISE"=w2463:cluster{"T-RISE (L)":dbl, "T-RISE (N)":dbl}, "Result Out"=w2465:bool, "file error"=w2468:errorcluster)  [unwired: 10 in]
                    n1727 = local write "TEMP RISE LAB01-2"(w2463) -> ()
                    n1728 = local write "FAIL LAB01-2"(w2466) -> ()
                    n1729 = local write "DISP LAB01-2"(w2469) -> ()
                    n1730 = local write "RESULT LAB01-2"(w2465) -> ()
                    n1731 = local write "data file error"(w2468) -> ()
                  }
                }
              }
              frame #2 {
                # "LAB02-1"
                n1732 = case shown="True" w2479 {
                  tunnel: w2481 -> [_ w2494]
                  tunnel: w2478 -> [_ w2491]
                  tunnel: w2480 -> [_ w2490]
                  frame False {
                  }
                  frame True {
                    n1733 = local read "TEMP START LAB02-1"() -> (w2496:cluster{"TL":dbl, "TN":dbl})
                    n1734 = local read "FAIL LAB02-1"() -> (w2487:cluster{"LO":dbl, "HI":dbl})
                    n1735 = local read "DATA LAB02-1"() -> (w2495:refnum<k1>)
                    n1736 = local read "SET LAB02-1"() -> (w2492:T5)
                    n1737 = local read "DISP LAB02-1"() -> (w2493:T4)
                    n1738 = local read "SIG LAB02-1"() -> (w2497:T2)
                    n1739 = local read "RESULT LAB02-1"() -> (w2484:bool)
                    n1740 = Bundle("FAIL LAB02-1"=w2487, "SIG LAB02-1"=w2497, "TEMP START LAB02-1"=w2496, "DISP LAB02-1"=w2493, "SET LAB02-1"=w2492, "DATA LAB02-1"=w2495) -> (w2482:T36)  [unwired: 1 in]
                    n1741 = call "sub vi - cycle&temp fail v5.vi"("Amps Lo?"=w2494, "Input Cluster"=w2482, "SELECT"=w2491, "Amps Hi?"=w2490, "Result In"=w2484) -> ("(FAIL) out"=w2486:cluster{"FAIL LO":dbl, "FAIL HI":dbl}, "(DISP) out"=w2489:T4, "T-RISE"=w2483:cluster{"T-RISE (L)":dbl, "T-RISE (N)":dbl}, "Result Out"=w2485:bool, "file error"=w2488:errorcluster)  [unwired: 10 in]
                    n1742 = local write "TEMP RISE LAB02-1"(w2483) -> ()
                    n1743 = local write "FAIL LAB02-1"(w2486) -> ()
                    n1744 = local write "DISP LAB02-1"(w2489) -> ()
                    n1745 = local write "RESULT LAB02-1"(w2485) -> ()
                    n1746 = local write "data file error"(w2488) -> ()
                  }
                }
              }
              frame #3 {
                # "LAB02-2"
                n1747 = case shown="True" w2499 {
                  tunnel: w2501 -> [_ w2514]
                  tunnel: w2498 -> [_ w2511]
                  tunnel: w2500 -> [_ w2510]
                  frame False {
                  }
                  frame True {
                    n1748 = local read "TEMP START LAB02-2"() -> (w2516:cluster{"TL":dbl, "TN":dbl})
                    n1749 = local read "FAIL LAB02-2"() -> (w2507:cluster{"LO":dbl, "HI":dbl})
                    n1750 = local read "DATA LAB02-2"() -> (w2515:refnum<k1>)
                    n1751 = local read "SET LAB02-2"() -> (w2512:T5)
                    n1752 = local read "DISP LAB02-2"() -> (w2513:T4)
                    n1753 = local read "SIG LAB02-2"() -> (w2517:T2)
                    n1754 = local read "RESULT LAB02-2"() -> (w2504:bool)
                    n1755 = Bundle("FAIL LAB02-2"=w2507, "SIG LAB02-2"=w2517, "TEMP START LAB02-2"=w2516, "DISP LAB02-2"=w2513, "SET LAB02-2"=w2512, "DATA LAB02-2"=w2515) -> (w2502:T37)  [unwired: 1 in]
                    n1756 = call "sub vi - cycle&temp fail v5.vi"("Amps Lo?"=w2514, "Input Cluster"=w2502, "SELECT"=w2511, "Amps Hi?"=w2510, "Result In"=w2504) -> ("(FAIL) out"=w2506:cluster{"FAIL LO":dbl, "FAIL HI":dbl}, "(DISP) out"=w2509:T4, "T-RISE"=w2503:cluster{"T-RISE (L)":dbl, "T-RISE (N)":dbl}, "Result Out"=w2505:bool, "file error"=w2508:errorcluster)  [unwired: 10 in]
                    n1757 = local write "TEMP RISE LAB02-2"(w2503) -> ()
                    n1758 = local write "FAIL LAB02-2"(w2506) -> ()
                    n1759 = local write "DISP LAB02-2"(w2509) -> ()
                    n1760 = local write "RESULT LAB02-2"(w2505) -> ()
                    n1761 = local write "data file error"(w2508) -> ()
                  }
                }
              }
              frame #4 {
                # "LAB03-1"
                n1762 = case shown="True" w2519 {
                  tunnel: w2521 -> [_ w2534]
                  tunnel: w2518 -> [_ w2531]
                  tunnel: w2520 -> [_ w2530]
                  frame False {
                  }
                  frame True {
                    n1763 = local read "TEMP START LAB03-1"() -> (w2536:cluster{"TL":dbl, "TN":dbl})
                    n1764 = local read "FAIL LAB03-1"() -> (w2527:cluster{"LO":dbl, "HI":dbl})
                    n1765 = local read "DATA LAB03-1"() -> (w2535:refnum<k1>)
                    n1766 = local read "SET LAB03-1"() -> (w2532:T5)
                    n1767 = local read "DISP LAB03-1"() -> (w2533:T4)
                    n1768 = local read "SIG LAB03-1"() -> (w2537:T2)
                    n1769 = local read "RESULT LAB03-1"() -> (w2524:bool)
                    n1770 = Bundle("FAIL LAB03-1"=w2527, "SIG LAB03-1"=w2537, "TEMP START LAB03-1"=w2536, "DISP LAB03-1"=w2533, "SET LAB03-1"=w2532, "DATA LAB03-1"=w2535) -> (w2522:T38)  [unwired: 1 in]
                    n1771 = call "sub vi - cycle&temp fail v5.vi"("Amps Lo?"=w2534, "Input Cluster"=w2522, "SELECT"=w2531, "Amps Hi?"=w2530, "Result In"=w2524) -> ("(FAIL) out"=w2526:cluster{"FAIL LO":dbl, "FAIL HI":dbl}, "(DISP) out"=w2529:T4, "T-RISE"=w2523:cluster{"T-RISE (L)":dbl, "T-RISE (N)":dbl}, "Result Out"=w2525:bool, "file error"=w2528:errorcluster)  [unwired: 10 in]
                    n1772 = local write "TEMP RISE LAB03-1"(w2523) -> ()
                    n1773 = local write "FAIL LAB03-1"(w2526) -> ()
                    n1774 = local write "DISP LAB03-1"(w2529) -> ()
                    n1775 = local write "RESULT LAB03-1"(w2525) -> ()
                    n1776 = local write "data file error"(w2528) -> ()
                  }
                }
              }
              frame #5 {
                # "LAB03-2"
                n1777 = case shown="True" w2539 {
                  tunnel: w2541 -> [_ w2554]
                  tunnel: w2538 -> [_ w2551]
                  tunnel: w2540 -> [_ w2550]
                  frame False {
                  }
                  frame True {
                    n1778 = local read "TEMP START LAB03-2"() -> (w2556:cluster{"TL":dbl, "TN":dbl})
                    n1779 = local read "FAIL LAB03-2"() -> (w2547:cluster{"LO":dbl, "HI":dbl})
                    n1780 = local read "DATA LAB03-2"() -> (w2555:refnum<k1>)
                    n1781 = local read "SET LAB03-2"() -> (w2552:T5)
                    n1782 = local read "DISP LAB03-2"() -> (w2553:T4)
                    n1783 = local read "RESULT LAB03-2"() -> (w2544:bool)
                    n1784 = local read "SIG LAB03-2"() -> (w2557:T2)
                    n1785 = Bundle("FAIL LAB03-2"=w2547, "SIG LAB03-2"=w2557, "TEMP START LAB03-2"=w2556, "DISP LAB03-2"=w2553, "SET LAB03-2"=w2552, "DATA LAB03-2"=w2555) -> (w2542:T39)  [unwired: 1 in]
                    n1786 = call "sub vi - cycle&temp fail v5.vi"("Amps Lo?"=w2554, "Input Cluster"=w2542, "SELECT"=w2551, "Amps Hi?"=w2550, "Result In"=w2544) -> ("(FAIL) out"=w2546:cluster{"FAIL LO":dbl, "FAIL HI":dbl}, "(DISP) out"=w2549:T4, "T-RISE"=w2543:cluster{"T-RISE (L)":dbl, "T-RISE (N)":dbl}, "Result Out"=w2545:bool, "file error"=w2548:errorcluster)  [unwired: 10 in]
                    n1787 = local write "FAIL LAB03-2"(w2546) -> ()
                    n1788 = local write "TEMP RISE LAB03-2"(w2543) -> ()
                    n1789 = local write "DISP LAB03-2"(w2549) -> ()
                    n1790 = local write "RESULT LAB03-2"(w2545) -> ()
                    n1791 = local write "data file error"(w2548) -> ()
                  }
                }
              }
              frame #6 {
                # "LAB04-1"
                n1792 = case shown="True" w2559 {
                  tunnel: w2561 -> [_ w2574]
                  tunnel: w2558 -> [_ w2571]
                  tunnel: w2560 -> [_ w2570]
                  frame False {
                  }
                  frame True {
                    n1793 = local read "TEMP START LAB04-1"() -> (w2576:cluster{"TL":dbl, "TN":dbl})
                    n1794 = local read "FAIL LAB04-1"() -> (w2567:cluster{"LO":dbl, "HI":dbl})
                    n1795 = local read "DATA LAB04-1"() -> (w2575:refnum<k1>)
                    n1796 = local read "SET LAB04-1"() -> (w2572:T5)
                    n1797 = local read "DISP LAB04-1"() -> (w2573:T4)
                    n1798 = local read "SIG LAB04-1"() -> (w2577:T2)
                    n1799 = local read "RESULT LAB04-1"() -> (w2564:bool)
                    n1800 = Bundle("FAIL LAB04-1"=w2567, "SIG LAB04-1"=w2577, "TEMP START LAB04-1"=w2576, "DISP LAB04-1"=w2573, "SET LAB04-1"=w2572, "DATA LAB04-1"=w2575) -> (w2562:T40)  [unwired: 1 in]
                    n1801 = call "sub vi - cycle&temp fail v5.vi"("Amps Lo?"=w2574, "Input Cluster"=w2562, "SELECT"=w2571, "Amps Hi?"=w2570, "Result In"=w2564) -> ("(FAIL) out"=w2566:cluster{"FAIL LO":dbl, "FAIL HI":dbl}, "(DISP) out"=w2569:T4, "T-RISE"=w2563:cluster{"T-RISE (L)":dbl, "T-RISE (N)":dbl}, "Result Out"=w2565:bool, "file error"=w2568:errorcluster)  [unwired: 10 in]
                    n1802 = local write "TEMP RISE LAB04-1"(w2563) -> ()
                    n1803 = local write "FAIL LAB04-1"(w2566) -> ()
                    n1804 = local write "DISP LAB04-1"(w2569) -> ()
                    n1805 = local write "RESULT LAB04-1"(w2565) -> ()
                    n1806 = local write "data file error"(w2568) -> ()
                  }
                }
              }
              frame #7 {
                # "LAB04-2"
                n1807 = case shown="True" w2579 {
                  tunnel: w2581 -> [_ w2594]
                  tunnel: w2578 -> [_ w2591]
                  tunnel: w2580 -> [_ w2590]
                  frame False {
                  }
                  frame True {
                    n1808 = local read "TEMP START LAB04-2"() -> (w2596:cluster{"TL":dbl, "TN":dbl})
                    n1809 = local read "FAIL LAB04-2"() -> (w2587:cluster{"LO":dbl, "HI":dbl})
                    n1810 = local read "DATA LAB04-2"() -> (w2595:refnum<k1>)
                    n1811 = local read "SET LAB04-2"() -> (w2592:T5)
                    n1812 = local read "DISP LAB04-2"() -> (w2593:T4)
                    n1813 = local read "SIG LAB04-2"() -> (w2597:T2)
                    n1814 = local read "RESULT LAB04-2"() -> (w2584:bool)
                    n1815 = Bundle("FAIL LAB04-2"=w2587, "SIG LAB04-2"=w2597, "TEMP START LAB04-2"=w2596, "DISP LAB04-2"=w2593, "SET LAB04-2"=w2592, "DATA LAB04-2"=w2595) -> (w2582:T41)  [unwired: 1 in]
                    n1816 = call "sub vi - cycle&temp fail v5.vi"("Amps Lo?"=w2594, "Input Cluster"=w2582, "SELECT"=w2591, "Amps Hi?"=w2590, "Result In"=w2584) -> ("(FAIL) out"=w2586:cluster{"FAIL LO":dbl, "FAIL HI":dbl}, "(DISP) out"=w2589:T4, "T-RISE"=w2583:cluster{"T-RISE (L)":dbl, "T-RISE (N)":dbl}, "Result Out"=w2585:bool, "file error"=w2588:errorcluster)  [unwired: 10 in]
                    n1817 = local write "TEMP RISE LAB04-2"(w2583) -> ()
                    n1818 = local write "FAIL LAB04-2"(w2586) -> ()
                    n1819 = local write "DISP LAB04-2"(w2589) -> ()
                    n1820 = local write "RESULT LAB04-2"(w2585) -> ()
                    n1821 = local write "data file error"(w2588) -> ()
                  }
                }
              }
              frame #8 {
                # "LAB05-1"
                n1822 = case shown="True" w2599 {
                  tunnel: w2601 -> [_ w2614]
                  tunnel: w2598 -> [_ w2611]
                  tunnel: w2600 -> [_ w2610]
                  frame False {
                  }
                  frame True {
                    n1823 = local read "TEMP START LAB05-1"() -> (w2616:cluster{"TL":dbl, "TN":dbl})
                    n1824 = local read "FAIL LAB05-1"() -> (w2607:cluster{"LO":dbl, "HI":dbl})
                    n1825 = local read "DATA LAB05-1"() -> (w2615:refnum<k1>)
                    n1826 = local read "SET LAB05-1"() -> (w2612:T5)
                    n1827 = local read "DISP LAB05-1"() -> (w2613:T4)
                    n1828 = local read "SIG LAB05-1"() -> (w2617:T2)
                    n1829 = local read "RESULT LAB05-1"() -> (w2604:bool)
                    n1830 = Bundle("FAIL LAB05-1"=w2607, "SIG LAB05-1"=w2617, "TEMP START LAB05-1"=w2616, "DISP LAB05-1"=w2613, "SET LAB05-1"=w2612, "DATA LAB05-1"=w2615) -> (w2602:T42)  [unwired: 1 in]
                    n1831 = call "sub vi - cycle&temp fail v5.vi"("Amps Lo?"=w2614, "Input Cluster"=w2602, "SELECT"=w2611, "Amps Hi?"=w2610, "Result In"=w2604) -> ("(FAIL) out"=w2606:cluster{"FAIL LO":dbl, "FAIL HI":dbl}, "(DISP) out"=w2609:T4, "T-RISE"=w2603:cluster{"T-RISE (L)":dbl, "T-RISE (N)":dbl}, "Result Out"=w2605:bool, "file error"=w2608:errorcluster)  [unwired: 10 in]
                    n1832 = local write "TEMP RISE LAB05-1"(w2603) -> ()
                    n1833 = local write "FAIL LAB05-1"(w2606) -> ()
                    n1834 = local write "DISP LAB05-1"(w2609) -> ()
                    n1835 = local write "RESULT LAB05-1"(w2605) -> ()
                    n1836 = local write "data file error"(w2608) -> ()
                  }
                }
              }
              frame #9 {
                # "LAB05-2"
                n1837 = case shown="True" w2619 {
                  tunnel: w2621 -> [_ w2634]
                  tunnel: w2618 -> [_ w2631]
                  tunnel: w2620 -> [_ w2630]
                  frame False {
                  }
                  frame True {
                    n1838 = local read "TEMP START LAB05-2"() -> (w2636:cluster{"TL":dbl, "TN":dbl})
                    n1839 = local read "FAIL LAB05-2"() -> (w2627:cluster{"LO":dbl, "HI":dbl})
                    n1840 = local read "DATA LAB05-2"() -> (w2635:refnum<k1>)
                    n1841 = local read "SET LAB05-2"() -> (w2632:T5)
                    n1842 = local read "DISP LAB05-2"() -> (w2633:T4)
                    n1843 = local read "SIG LAB05-2"() -> (w2637:T2)
                    n1844 = local read "RESULT LAB05-2"() -> (w2624:bool)
                    n1845 = Bundle("FAIL LAB05-2"=w2627, "SIG LAB05-2"=w2637, "TEMP START LAB05-2"=w2636, "DISP LAB05-2"=w2633, "SET LAB05-2"=w2632, "DATA LAB05-2"=w2635) -> (w2622:T43)  [unwired: 1 in]
                    n1846 = call "sub vi - cycle&temp fail v5.vi"("Amps Lo?"=w2634, "Input Cluster"=w2622, "SELECT"=w2631, "Amps Hi?"=w2630, "Result In"=w2624) -> ("(FAIL) out"=w2626:cluster{"FAIL LO":dbl, "FAIL HI":dbl}, "(DISP) out"=w2629:T4, "T-RISE"=w2623:cluster{"T-RISE (L)":dbl, "T-RISE (N)":dbl}, "Result Out"=w2625:bool, "file error"=w2628:errorcluster)  [unwired: 10 in]
                    n1847 = local write "TEMP RISE LAB05-2"(w2623) -> ()
                    n1848 = local write "FAIL LAB05-2"(w2626) -> ()
                    n1849 = local write "DISP LAB05-2"(w2629) -> ()
                    n1850 = local write "RESULT LAB05-2"(w2625) -> ()
                    n1851 = local write "data file error"(w2628) -> ()
                  }
                }
              }
            }
          }
          frame #14 {
            # "run calibration routine"
            n1852 = local read "CALIBRATE"() -> (w2638:bool)
            n1853 = case shown="True" w2638 {
              frame False {
              }
              frame True {
                n1854 = stacked-sequence {
                  seq-local: [w2639 _ _] -> [_ w2641 _]
                  frame #0 {
                    n1855 = call "CALIBRATION PASSWORD"() -> ("PASSWORD"=w2639:string)  [unwired: 17 in, 2 out]
                  }
                  frame #1 {
                    n1856 = Equal?(x=w2641, y="7777") -> (x = y?=w2640:bool)
                    n1857 = case shown="True" w2640 {
                      frame False {
                      }
                      frame True {
                        n1858 = stacked-sequence {
                          frame #0 {
                            n1859 = call "sub vi - calibration v1.vi"() -> ()  [unwired: 12 in]
                          }
                          frame #1 {
                            n1860 = call "sub vi - get calibration values v1.vi"() -> ("LAB01 (CAL)"=w2647:T7, "LAB02 (CAL)"=w2646:T8, "LAB03 (CAL)"=w2645:T7, "LAB04 (CAL)"=w2644:T7, "calibration file error out"=w2648:errorcluster, "LAB05 (CAL)"=w2643:T7)  [unwired: 10 in]
                            n1861 = local write "calibration file error out"(w2648) -> ()
                            n1862 = local write "CAL LAB04"(w2644) -> ()
                            n1863 = local write "CAL LAB05"(w2643) -> ()
                            n1864 = local write "CAL LAB01"(w2647) -> ()
                            n1865 = local write "CAL LAB02"(w2646) -> ()
                            n1866 = local write "CAL LAB03"(w2645) -> ()
                          }
                        }
                      }
                    }
                  }
                  frame #2 {
                    n1867 = local write "CALIBRATE"(FALSE) -> ()
                  }
                }
              }
            }
          }
          frame #15 {
            # "save certain settings to file"
            n1868 = String To Path(string="c:\\crabtree\\Set Up\\") -> (path=w2651:path)
            n1869 = Build Path(base path=w2651, name or relative path="settings.bin") -> (appended path=w2653:path)
            n1870 = Build Path(base path=w2651, name or relative path="mail.bin") -> (appended path=w2650:path)
            n1871 = Create Folder(path (use dialog)=w2651) -> (error out=w2656:errorcluster)  [unwired: 2 in, 2 out]
            n1872 = call <vilib>:"Clear Errors.vi"("error in (no error)"=w2656) -> ()  [unwired: 6 in, 1 out]
            n1873 = stacked-sequence {
              seq-local: [w2658 _] -> [_ w2671]
              tunnel: w2653 -> [_ w2672]
              tunnel: w2650 -> [_ w2670]
              frame #0 {
                n1874 = local read "C drive data root dir"() -> (w2657:path)
                n1875 = local read "Network Directory"() -> (w2663:path)
                n1876 = local read "SET LAB05-2"() -> (w2662:T5)
                n1877 = local read "SET LAB05-1"() -> (w2661:T5)
                n1878 = local read "SET LAB04-2"() -> (w2660:T5)
                n1879 = local read "SET LAB03-2"() -> (w2664:T5)
                n1880 = local read "SET LAB04-1"() -> (w2659:T5)
                n1881 = local read "SET LAB03-1"() -> (w2665:T5)
                n1882 = local read "SET LAB02-2"() -> (w2666:T5)
                n1883 = local read "SET LAB02-1"() -> (w2667:T5)
                n1884 = local read "SET LAB01-2"() -> (w2668:T5)
                n1885 = local read "SET LAB01-1"() -> (w2669:T5)
                n1886 = Bundle("SET LAB01-1"=w2669, "SET LAB01-2"=w2668, "SET LAB02-1"=w2667, "SET LAB02-2"=w2666, "SET LAB03-1"=w2665, "SET LAB03-2"=w2664, "SET LAB04-1"=w2659, "SET LAB04-2"=w2660, "SET LAB05-1"=w2661, "SET LAB05-2"=w2662, "Network Directory"=w2663, "C drive data root dir"=w2657) -> (w2658:T16)  [unwired: 1 in]
              }
              frame #1 {
                n1887 = event shown="[1] \"SET LAB01-1\", \"SET LAB01-2\", \"SET LAB02-1\", \"SET LAB02-2\", \"SET LAB03-1\", \"SET LAB03-2\", \"SET LAB04-1\", \"SET LAB04-2\", \"SET LAB05-1\", \"SET LAB05-2\", \"Network Directory\", \"C drive data root dir\": Value Change" {
                  selector: _ -> [_ _ _]
                  dyn-events: _ -> [_ _ _]
                  timeout: 10.0 -> [_ _ _]
                  tunnel: w2672 -> [_ w2674 _]
                  tunnel: w2671 -> [_ w2675 _]
                  tunnel: w2670 -> [_ _ w2686]
                  event Timeout {
                    n1888 = event-data() -> ()  [unwired: 1 in, 3 out]
                  }
                  event "SET LAB01-1", "SET LAB01-2", "SET LAB02-1", "SET LAB02-2", "SET LAB03-1", "SET LAB03-2", "SET LAB04-1", "SET LAB04-2", "SET LAB05-1", "SET LAB05-2", "Network Directory", "C drive data root dir": Value Change {
                    n1889 = event-data() -> ()  [unwired: 1 in, 6 out]
                    n1890 = Open/Create/Replace File(file path (use dialog)=w2674, operation (0:open)=T15."replace or create") -> (refnum out=w2680:refnum<file>, error out=w2679:errorcluster)  [unwired: 4 in, 1 out]
                    n1891 = Write to Binary File(file (use dialog)=w2680, data=w2675, error in=w2679) -> (refnum out=w2678:refnum<file>, error out=w2677:errorcluster)  [unwired: 3 in, 1 out]
                    n1892 = Close File(refnum=w2678, error in=w2677) -> (error out=w2676:errorcluster)  [unwired: 1 out]
                    n1893 = local write "data file error"(w2676) -> ()
                  }
                  event "MAIL SETTINGS.OUT SERVER ADDRESS", "MAIL SETTINGS.FROM ACCOUNT", "MAIL SETTINGS.USER NAME", "MAIL SETTINGS.PASSWORD", "Auto Mail Send", "TO (string):": Value Change {
                    n1894 = event-data() -> ()  [unwired: 1 in, 6 out]
                    n1895 = local read "MAIL SETTINGS"() -> (w2685:T6)
                    n1896 = local read "Auto Mail Send"() -> (w2683:bool)
                    n1897 = local read "TO (string):"() -> (w2682:string)
                    n1898 = Open/Create/Replace File(file path (use dialog)=w2686, operation (0:open)=T15."replace or create") -> (refnum out=w2691:refnum<file>, error out=w2690:errorcluster)  [unwired: 4 in, 1 out]
                    n1899 = Bundle("MAIL SETTINGS"=w2685, "Auto Mail Send"=w2683, "TO (string):"=w2682) -> (w2684:T44)  [unwired: 1 in]
                    n1900 = Write to Binary File(file (use dialog)=w2691, data=w2684, error in=w2690) -> (refnum out=w2689:refnum<file>, error out=w2688:errorcluster)  [unwired: 3 in, 1 out]
                    n1901 = Close File(refnum=w2689, error in=w2688) -> (error out=w2687:errorcluster)  [unwired: 1 out]
                    n1902 = local write "data file error"(w2687) -> ()
                  }
                }
              }
            }
          }
          frame #16 {
            # "mail control"
            n1903 = local read "MAIL SETTINGS"() -> (w2708:T6)
            n1904 = local read "Auto Mail Send"() -> (w2694:bool)
            n1905 = Unbundle(w2708) -> ("OUT SERVER ADDRESS"=w2707:string, "FROM ACCOUNT"=w2706:string, "TEST MAIL"=w2705:bool)  [unwired: 4 out]
            n1906 = stacked-sequence {
              tunnel: "TO (string):" -> [_ w2747]
              tunnel: w2708 -> [w2713 w2746]
              tunnel: w2707 -> [w2712 w2745]
              tunnel: w2706 -> [w2711 w2744]
              tunnel: w2705 -> [w2710 _]
              tunnel: w2694 -> [_ w2743]
              tunnel: w2704 -> [_ w2742]
              tunnel: w2703 -> [_ w2741]
              tunnel: w2702 -> [_ w2740]
              tunnel: w2701 -> [_ w2739]
              tunnel: w2700 -> [_ w2738]
              tunnel: w2699 -> [_ w2737]
              tunnel: w2698 -> [_ w2736]
              tunnel: w2697 -> [_ w2735]
              tunnel: w2696 -> [_ w2734]
              tunnel: w2695 -> [_ w2733]
              tunnel: "TO (string):" -> [w2709 _]
              frame #0 {
                # "mail test"
                n1907 = case shown="True" w2710 {
                  tunnel: w2713 -> [_ w2717]
                  tunnel: w2709 -> [_ w2716]
                  tunnel: w2712 -> [_ w2715]
                  tunnel: w2711 -> [_ w2714]
                  frame False {
                  }
                  frame True {
                    n1908 = stacked-sequence {
                      seq-local: [_ _ w2727 _] -> [_ _ _ w2728]
                      tunnel: w2717 -> [w2720 _ _ w2732]
                      tunnel: w2716 -> [_ _ w2725 _]
                      tunnel: w2715 -> [_ _ w2723 _]
                      tunnel: w2714 -> [_ _ w2724 _]
                      frame #0 {
                        n1909 = Bundle(cluster=w2720, "TEST MAIL STATUS"="TEST START") -> (w2718:T6)  [unwired: 6 in]
                        n1910 = local write "MAIL SETTINGS"(w2718) -> ()
                      }
                      frame #1 {
                        n1911 = Wait (ms)(milliseconds to wait=500) -> ()  [unwired: 1 out]
                      }
                      frame #2 {
                        n1912 = call "sub vi - send mail with attach v5.vi"("TO:"=w2725, "subject"="MAIL TEST FROM LAB PANEL", "from"=w2724, "out going server"=w2723, "message"="TEST MESSAGE") -> ("error out"=w2727:errorcluster)  [unwired: 10 in]
                      }
                      frame #3 {
                        n1913 = Bundle(cluster=w2732, "TEST MAIL"=FALSE, "TEST MAIL STATUS"="TEST END", "mail error"=w2728) -> (w2730:T6)  [unwired: 4 in]
                        n1914 = local write "MAIL SETTINGS"(w2730) -> ()
                      }
                    }
                  }
                }
              }
              frame #1 {
                # "mail report"
                n1915 = stacked-sequence {
                  seq-local: [_ w2812 _ _] -> [_ _ _ w2980]
                  seq-local: [_ _ w2893 _] -> [_ _ _ w2970]
                  seq-local: [w2757 _ _ _] -> [_ w2806 _ _]
                  seq-local: [w2756 _ _ _] -> [_ w2805 _ _]
                  seq-local: [w2754 _ _ _] -> [_ w2803 _ _]
                  seq-local: [w2755 _ _ _] -> [_ w2804 _ _]
                  seq-local: [w2753 _ _ _] -> [_ w2802 _ _]
                  seq-local: [w2752 _ _ _] -> [_ w2797 _ _]
                  seq-local: [w2751 _ _ _] -> [_ w2798 _ _]
                  seq-local: [w2750 _ _ _] -> [_ w2799 _ _]
                  seq-local: [w2749 _ _ _] -> [_ w2800 _ _]
                  seq-local: [w2748 _ _ _] -> [_ w2801 _ _]
                  tunnel: w2747 -> [_ _ _ w2981]
                  tunnel: w2746 -> [_ _ _ w2964]
                  tunnel: w2745 -> [_ _ _ w2978]
                  tunnel: w2744 -> [_ _ _ w2977]
                  tunnel: w2743 -> [w2788 _ _ w2972]
                  tunnel: w2742 -> [_ _ w2923 _]
                  tunnel: w2741 -> [_ _ w2920 _]
                  tunnel: w2740 -> [_ _ w2919 _]
                  tunnel: w2739 -> [_ _ w2918 _]
                  tunnel: w2738 -> [_ _ w2917 _]
                  tunnel: w2737 -> [_ _ w2916 _]
                  tunnel: w2736 -> [_ _ w2915 _]
                  tunnel: w2735 -> [_ _ w2914 _]
                  tunnel: w2734 -> [_ _ w2913 _]
                  tunnel: w2733 -> [_ _ w2912 _]
                  frame #0 {
                    n1916 = case shown="False" w2788 {
                      frame False {
                        n1917 = local write "mail control"("") -> ()
                      }
                      frame True {
                      }
                    }
                    n1918 = local read "SET LAB01-1"() -> (w2787:T5)
                    n1919 = local read "SET LAB01-2"() -> (w2786:T5)
                    n1920 = local read "SET LAB02-1"() -> (w2785:T5)
                    n1921 = local read "SET LAB02-2"() -> (w2784:T5)
                    n1922 = local read "SET LAB03-1"() -> (w2783:T5)
                    n1923 = local read "SET LAB04-1"() -> (w2781:T5)
                    n1924 = local read "SET LAB05-1"() -> (w2779:T5)
                    n1925 = local read "SET LAB03-2"() -> (w2782:T5)
                    n1926 = local read "SET LAB04-2"() -> (w2780:T5)
                    n1927 = local read "SET LAB05-2"() -> (w2778:T5)
                    n1928 = Unbundle(w2783) -> ("DESCRIPTION"=w2763:string)  [unwired: 4 out]
                    n1929 = Unbundle(w2782) -> ("DESCRIPTION"=w2762:string)  [unwired: 4 out]
                    n1930 = Unbundle(w2781) -> ("DESCRIPTION"=w2761:string)  [unwired: 4 out]
                    n1931 = Unbundle(w2778) -> ("DESCRIPTION"=w2758:string)  [unwired: 4 out]
                    n1932 = Unbundle(w2784) -> ("DESCRIPTION"=w2764:string)  [unwired: 4 out]
                    n1933 = Unbundle(w2780) -> ("DESCRIPTION"=w2760:string)  [unwired: 4 out]
                    n1934 = Unbundle(w2787) -> ("DESCRIPTION"=w2776:string)  [unwired: 4 out]
                    n1935 = Unbundle(w2785) -> ("DESCRIPTION"=w2765:string)  [unwired: 4 out]
                    n1936 = Unbundle(w2779) -> ("DESCRIPTION"=w2759:string)  [unwired: 4 out]
                    n1937 = Unbundle(w2786) -> ("DESCRIPTION"=w2766:string)  [unwired: 4 out]
                    n1938 = Concatenate Strings("[LAB05-1/", w2758) -> (w2748:string)
                    n1939 = Concatenate Strings("[LAB05-2/", w2759) -> (w2749:string)
                    n1940 = Concatenate Strings("[LAB04-2/", w2760) -> (w2750:string)
                    n1941 = Concatenate Strings("[LAB03-2/", w2762) -> (w2752:string)
                    n1942 = Concatenate Strings("[LAB04-1/", w2761) -> (w2751:string)
                    n1943 = Concatenate Strings("[LAB03-1/", w2763) -> (w2753:string)
                    n1944 = Concatenate Strings("[LAB01-2/", w2766) -> (w2756:string)
                    n1945 = Concatenate Strings("[LAB02-2/", w2764) -> (w2754:string)
                    n1946 = Concatenate Strings("[LAB01-1/", w2776) -> (w2757:string)
                    n1947 = Concatenate Strings("[LAB02-1/", w2765) -> (w2755:string)
                  }
                  frame #1 {
                    w2810 = "/"
                    w2811 = 2.0
                    n1948 = local read "DISP LAB01-2"() -> (w2891:T4)
                    n1949 = local read "DISP LAB01-1"() -> (w2892:T4)
                    n1950 = local read "DISP LAB02-1"() -> (w2890:T4)
                    n1951 = local read "DISP LAB03-2"() -> (w2887:T4)
                    n1952 = local read "DISP LAB02-2"() -> (w2889:T4)
                    n1953 = local read "DISP LAB03-1"() -> (w2888:T4)
                    n1954 = local read "DISP LAB04-2"() -> (w2885:T4)
                    n1955 = local read "DISP LAB04-1"() -> (w2886:T4)
                    n1956 = local read "DISP LAB05-1"() -> (w2884:T4)
                    n1957 = local read "DISP LAB05-2"() -> (w2883:T4)
                    n1958 = Unbundle(w2891) -> ("CYCLE"=w2875:dbl, "MINS"=w2874:dbl, "STATUS"=w2871:string)
                    n1959 = Unbundle(w2892) -> ("CYCLE"=w2880:dbl, "MINS"=w2879:dbl, "STATUS"=w2876:string)
                    n1960 = Unbundle(w2890) -> ("CYCLE"=w2868:dbl, "MINS"=w2867:dbl, "STATUS"=w2866:string)
                    n1961 = Unbundle(w2887) -> ("CYCLE"=w2855:dbl, "MINS"=w2854:dbl, "STATUS"=w2851:string)
                    n1962 = Unbundle(w2888) -> ("CYCLE"=w2860:dbl, "MINS"=w2859:dbl, "STATUS"=w2856:string)
                    n1963 = Unbundle(w2889) -> ("CYCLE"=w2865:dbl, "MINS"=w2864:dbl, "STATUS"=w2861:string)
                    n1964 = Unbundle(w2886) -> ("CYCLE"=w2850:dbl, "MINS"=w2849:dbl, "STATUS"=w2846:string)
                    n1965 = Unbundle(w2885) -> ("CYCLE"=w2845:dbl, "MINS"=w2844:dbl, "STATUS"=w2841:string)
                    n1966 = Unbundle(w2884) -> ("CYCLE"=w2840:dbl, "MINS"=w2839:dbl, "STATUS"=w2836:string)
                    n1967 = Unbundle(w2883) -> ("CYCLE"=w2882:dbl, "MINS"=w2881:dbl, "STATUS"=w2833:string)
                    n1968 = Number To Decimal String(number=w2868) -> (decimal integer string=w2870:string)  [unwired: 1 in]
                    n1969 = Number To Decimal String(number=w2865) -> (decimal integer string=w2863:string)  [unwired: 1 in]
                    n1970 = Number To Decimal String(number=w2860) -> (decimal integer string=w2858:string)  [unwired: 1 in]
                    n1971 = Number To Decimal String(number=w2875) -> (decimal integer string=w2873:string)  [unwired: 1 in]
                    n1972 = Number To Decimal String(number=w2855) -> (decimal integer string=w2853:string)  [unwired: 1 in]
                    n1973 = Number To Decimal String(number=w2880) -> (decimal integer string=w2878:string)  [unwired: 1 in]
                    n1974 = Number To Decimal String(number=w2882) -> (decimal integer string=w2835:string)  [unwired: 1 in]
                    n1975 = Number To Decimal String(number=w2850) -> (decimal integer string=w2848:string)  [unwired: 1 in]
                    n1976 = Number To Decimal String(number=w2845) -> (decimal integer string=w2843:string)  [unwired: 1 in]
                    n1977 = Number To Decimal String(number=w2840) -> (decimal integer string=w2838:string)  [unwired: 1 in]
                    n1978 = Number To Fractional String(number=w2867, precision (6)=w2811) -> (F-format string=w2869:string)  [unwired: 2 in]
                    n1979 = Number To Fractional String(number=w2854, precision (6)=w2811) -> (F-format string=w2852:string)  [unwired: 2 in]
                    n1980 = Number To Fractional String(number=w2864, precision (6)=w2811) -> (F-format string=w2862:string)  [unwired: 2 in]
                    n1981 = Number To Fractional String(number=w2859, precision (6)=w2811) -> (F-format string=w2857:string)  [unwired: 2 in]
                    n1982 = Number To Fractional String(number=w2844, precision (6)=w2811) -> (F-format string=w2842:string)  [unwired: 2 in]
                    n1983 = Number To Fractional String(number=w2849, precision (6)=w2811) -> (F-format string=w2847:string)  [unwired: 2 in]
                    n1984 = Number To Fractional String(number=w2874, precision (6)=w2811) -> (F-format string=w2872:string)  [unwired: 2 in]
                    n1985 = Number To Fractional String(number=w2839, precision (6)=w2811) -> (F-format string=w2837:string)  [unwired: 2 in]
                    n1986 = Number To Fractional String(number=w2879, precision (6)=w2811) -> (F-format string=w2877:string)  [unwired: 2 in]
                    n1987 = Number To Fractional String(number=w2881, precision (6)=w2811) -> (F-format string=w2834:string)  [unwired: 2 in]
                    n1988 = Concatenate Strings(w2810, w2853, w2810, w2852, w2810, w2851) -> (w2827:string)
                    n1989 = Concatenate Strings(w2810, w2848, w2810, w2847, w2810, w2846) -> (w2826:string)
                    n1990 = Concatenate Strings(w2810, w2843, w2810, w2842, w2810, w2841) -> (w2825:string)
                    n1991 = Concatenate Strings(w2810, w2838, w2810, w2837, w2810, w2836) -> (w2824:string)
                    n1992 = Concatenate Strings(w2810, w2835, w2810, w2834, w2810, w2833) -> (w2823:string)
                    n1993 = Concatenate Strings(w2810, w2878, w2810, w2877, w2810, w2876) -> (w2832:string)
                    n1994 = Concatenate Strings(w2810, w2858, w2810, w2857, w2810, w2856) -> (w2828:string)
                    n1995 = Concatenate Strings(w2810, w2873, w2810, w2872, w2810, w2871) -> (w2831:string)
                    n1996 = Concatenate Strings(w2810, w2870, w2810, w2869, w2810, w2866) -> (w2830:string)
                    n1997 = Concatenate Strings(w2810, w2863, w2810, w2862, w2810, w2861) -> (w2829:string)
                    n1998 = Concatenate Strings("]", "\r") -> (w2807:string)
                    n1999 = Concatenate Strings(w2802, w2828, w2807) -> (w2818:string)
                    n2000 = Concatenate Strings(w2804, w2830, w2807) -> (w2820:string)
                    n2001 = Concatenate Strings(w2803, w2829, w2807) -> (w2819:string)
                    n2002 = Concatenate Strings(w2799, w2825, w2807) -> (w2815:string)
                    n2003 = Concatenate Strings(w2800, w2824, w2807) -> (w2816:string)
                    n2004 = Concatenate Strings(w2798, w2826, w2807) -> (w2814:string)
                    n2005 = Concatenate Strings(w2797, w2827, w2807) -> (w2813:string)
                    n2006 = Concatenate Strings(w2801, w2823, w2807) -> (w2817:string)
                    n2007 = Concatenate Strings(w2805, w2831, w2807) -> (w2821:string)
                    n2008 = Concatenate Strings(w2806, w2832, w2807) -> (w2822:string)
                    n2009 = Concatenate Strings(w2822, w2821, w2820, w2819, w2818, w2813, w2814, w2815, w2816, w2817) -> (w2790:string)
                    n2010 = Concatenate Strings("[PANEL/", "DESC/", "CYCLES/", "MINS/", "STATUS]", "\r", w2790) -> (w2812:string)
                    "MAIL REPORT" <- w2812
                  }
                  frame #2 {
                    w2921 = "END"
                    n2011 = local read "mail control"() -> (w2922:string)
                    n2012 = case shown="False" w2917 {
                      tunnel: w2922 -> [w2946 _]
                      tunnel: w2921 -> [w2945 _]
                      tunnel: [w2944 FALSE] -> w2907
                      frame False {
                        n2013 = Equal?(x=w2946, y=w2945) -> (x = y?=w2944:bool)
                      }
                      frame True {
                      }
                    }
                    n2014 = case shown="False" w2923 {
                      tunnel: w2922 -> [w2962 _]
                      tunnel: w2921 -> [w2961 _]
                      tunnel: [w2960 FALSE] -> w2911
                      frame False {
                        n2015 = Equal?(x=w2962, y=w2961) -> (x = y?=w2960:bool)
                      }
                      frame True {
                      }
                    }
                    n2016 = case shown="False" w2920 {
                      tunnel: w2922 -> [w2958 _]
                      tunnel: w2921 -> [w2957 _]
                      tunnel: [w2956 FALSE] -> w2910
                      frame False {
                        n2017 = Equal?(x=w2958, y=w2957) -> (x = y?=w2956:bool)
                      }
                      frame True {
                      }
                    }
                    n2018 = case shown="False" w2918 {
                      tunnel: w2922 -> [w2950 _]
                      tunnel: w2921 -> [w2949 _]
                      tunnel: [w2948 FALSE] -> w2908
                      frame False {
                        n2019 = Equal?(x=w2950, y=w2949) -> (x = y?=w2948:bool)
                      }
                      frame True {
                      }
                    }
                    n2020 = case shown="False" w2919 {
                      tunnel: w2922 -> [w2954 _]
                      tunnel: w2921 -> [w2953 _]
                      tunnel: [w2952 FALSE] -> w2909
                      frame False {
                        n2021 = Equal?(x=w2954, y=w2953) -> (x = y?=w2952:bool)
                      }
                      frame True {
                      }
                    }
                    n2022 = Or(x=w2909, y=w2908) -> (x .or. y?=w2900:bool)
                    n2023 = Or(x=w2911, y=w2910) -> (x .or. y?=w2901:bool)
                    n2024 = Or(x=w2901, y=w2900) -> (x .or. y?=w2896:bool)
                    n2025 = case shown="False" w2913 {
                      tunnel: w2922 -> [w2930 _]
                      tunnel: w2921 -> [w2929 _]
                      tunnel: [w2928 FALSE] -> w2902
                      frame False {
                        n2026 = Equal?(x=w2930, y=w2929) -> (x = y?=w2928:bool)
                      }
                      frame True {
                      }
                    }
                    n2027 = case shown="False" w2912 {
                      tunnel: w2922 -> [w2926 _]
                      tunnel: w2921 -> [w2925 _]
                      tunnel: [w2924 FALSE] -> w2906
                      frame False {
                        n2028 = Equal?(x=w2926, y=w2925) -> (x = y?=w2924:bool)
                      }
                      frame True {
                      }
                    }
                    n2029 = case shown="False" w2914 {
                      tunnel: w2922 -> [w2934 _]
                      tunnel: w2921 -> [w2933 _]
                      tunnel: [w2932 FALSE] -> w2903
                      frame False {
                        n2030 = Equal?(x=w2934, y=w2933) -> (x = y?=w2932:bool)
                      }
                      frame True {
                      }
                    }
                    n2031 = case shown="False" w2916 {
                      tunnel: w2922 -> [w2942 _]
                      tunnel: w2921 -> [w2941 _]
                      tunnel: [w2940 FALSE] -> w2905
                      frame False {
                        n2032 = Equal?(x=w2942, y=w2941) -> (x = y?=w2940:bool)
                      }
                      frame True {
                      }
                    }
                    n2033 = case shown="False" w2915 {
                      tunnel: w2922 -> [w2938 _]
                      tunnel: w2921 -> [w2937 _]
                      tunnel: [w2936 FALSE] -> w2904
                      frame False {
                        n2034 = Equal?(x=w2938, y=w2937) -> (x = y?=w2936:bool)
                      }
                      frame True {
                      }
                    }
                    n2035 = Or(x=w2905, y=w2904) -> (x .or. y?=w2899:bool)
                    n2036 = Or(x=w2903, y=w2902) -> (x .or. y?=w2898:bool)
                    n2037 = Or(x=w2906, y=w2907) -> (x .or. y?=w2894:bool)
                    n2038 = Or(x=w2899, y=w2898) -> (x .or. y?=w2897:bool)
                    n2039 = Or(x=w2896, y=w2897) -> (x .or. y?=w2895:bool)
                    n2040 = Or(x=w2895, y=w2894) -> (x .or. y?=w2893:bool)
                  }
                  frame #3 {
                    n2041 = local read "on loops"() -> (w2976:dbl)
                    n2042 = local read "jig cycle"() -> (w2973:dbl)
                    n2043 = local read "Send Mail Now"() -> (w2967:bool)
                    n2044 = Add(x=w2976, y=3.0) -> (x+y=w2974:dbl)
                    n2045 = Equal?(x=w2973, y=w2974) -> (x = y?=w2968:bool)
                    n2046 = And(x=w2968, y=w2967) -> (x .and. y?=w2966:bool)
                    n2047 = And(x=w2972, y=w2968) -> (x .and. y?=w2971:bool)
                    n2048 = And(x=w2971, y=w2970) -> (x .and. y?=w2969:bool)
                    n2049 = Or(x=w2969, y=w2966) -> (x .or. y?=w2965:bool)
                    n2050 = case shown="True" w2965 {
                      tunnel: w2981 -> [_ w2987]
                      tunnel: w2980 -> [_ w2986]
                      tunnel: "Lab Panel Test Status" -> [_ w2985]
                      tunnel: w2978 -> [_ w2984]
                      tunnel: w2977 -> [_ w2983]
                      tunnel: w2964 -> [_ w2982]
                      frame False {
                      }
                      frame True {
                        n2051 = stacked-sequence {
                          tunnel: w2987 -> [w2995 _]
                          tunnel: w2986 -> [w2994 _]
                          tunnel: w2985 -> [w2993 _]
                          tunnel: w2984 -> [w2992 _]
                          tunnel: w2983 -> [w2991 _]
                          tunnel: w2982 -> [w2990 _]
                          frame #0 {
                            n2052 = call "sub vi - send mail with attach v5.vi"("TO:"=w2995, "subject"=w2993, "from"=w2991, "out going server"=w2992, "message"=w2994) -> ("error out"=w2989:errorcluster)  [unwired: 10 in]
                            n2053 = Bundle(cluster=w2990, "mail error"=w2989) -> (w2988:T6)  [unwired: 6 in]
                            n2054 = local write "MAIL SETTINGS"(w2988) -> ()
                          }
                          frame #1 {
                            n2055 = local write "mail control"("") -> ()
                            n2056 = local write "Send Mail Now"(FALSE) -> ()
                          }
                        }
                      }
                    }
                  }
                }
              }
            }
          }
        }
        n2057 = node-c288() -> ()  [unwired: 1 in, 1 out]
        "loops" <- w165
        "stop2" <- "stop"
      }
      n2058 = node-c288(w142) -> ()  [unwired: 1 out]
    }
  }
